vi "OP_Print_TPS_cluster20171206.vi"() -> ()   [LabVIEW 2013]
uses:
  <vilib>/addons/database/Connection.llb/DB Tools Open Connec (Path).vi
  <vilib>/addons/database/Connection.llb/Conn Execute.vi
  <vilib>/addons/database/Recordset.llb/Rec Fetch Recordset Data (R).vi
  <vilib>/addons/database/Recordset.llb/Rec Destroy - Connection.vi
  <userlib>/caLab/Private/Get_PV-1D.vi
  <vilib>/Utility/file.llb/Write To Spreadsheet File (string).vi
  <userlib>/caLab/Private/Get_PV.vi
  <vilib>/addons/database/NI_Database_API.lvlib
panel:
  in  "WindowsMediaPlayer":refnum<k7>(container)
  in  "Vol.":i32(slide)=12 min=0 max=100 step=1 scale=0.0..100.0
  out "index":i32
  in  "Play Button":bool
  in  "Skip Forward Button":bool
  in  "Skip Back Button":bool
  in  "Pause Button":bool
  out "appended path":path=path "C:/Users/TPSOP/Desktop/新增資料夾 (2)/musics/1.mp3"
  out "status":string="就緒"
  out "error out":errorcluster
  out "new picture":picture
  in  "T:Slow\nF:Fast":bool
  in  "Switch Tab":bool=TRUE
  out "Tab Control":enum32{"_____", "           "}(tab)
  out "Cluster":T1={"SR Fill Pattern"=[], "Beam Current(mA"=320.769453, "Beam Lifetime(min)"=354.3939151043138, "Beamsize X(um)"=63.15189373514937, "Beamsize Y(um)"=38.03691397287648, "Tune X(from BPM)"=0.1487279843444227, "Tune Y(from BPM)"=0.2309197651663405, "Mode"="Top-Up", "NuX(from BBF) "=0.15142063757609414, "NuY(from BBF)"=0.22496346361412184, "IU22-23gap(R)"=7.0, "IU22-05gap(R)"=7.372, "IU22-05M"=TRUE, "IU22A-09gap(R)"=8.05, "IU22A-09M"=TRUE, "IU22B-09gap(R)"=40.001, "IU22B-09M"=FALSE, "IUT22-21gap(R)"=7.0, "IUT22-21M"=TRUE, "IU22-23M"=TRUE, "IU22A-25gap(R)"=7.0, "IU22A-25M"=TRUE, "IU22B-25gap(R)"=40.0, "IU22B-25M"=FALSE, "EPU48A-41gap(R)"=65.00055, "EPU48A-41gM"=FALSE, "EPU48B-41gap(R)"=27.450000000000003, "EPU48B-41gM"=TRUE, "EPU46-45gap(R)"=44.99850000000001, "EPU46-45gM"=FALSE, "EPU48A-41phase(R)"=0.00055, "EPU48B-41phase(R)"=0.0, "EPU46-45phase(R)"=5e-05, "Grid volt.(V)[S]"=33.0, "Gun mode"="MBM", "Mod.3 HV(kV)[S]"=35.37999999999996, "SR"="SR_DMB_2017_1024_0300LOCO.data", "BR"="Booster_2017_1023_0900.data", "LI"="Linac_2017_0413_1015.data", "LTB"="LTB_JT_2017_0828_1050.data", "BTS"="BTS_2017_1023_0900.data", "RF2 remote"=TRUE, "RF2 OP mode"=TRUE, "RF2 phase.[S]"=-42.0, "RF Freq.(s)"=499655365.67399085, "RF2 gap volt[S]"=1600.0, "RF3 remote"=TRUE, "RF3 OP mode"=TRUE, "RF3 phase.[S]"=1.1999999999999995, "RF3 gap volt.[S]"=1600.0, "BBF V"=TRUE, "BBF H"=TRUE, "BR ext. kicker1(kV)"=17.666, "BR ext. kicker2(kV)"=17.666, "BR ext. sep.1(V)"=322.14, "BR ext. sep.2(V)"=441.1, "BR inj. sep.(V)"=104.95, "BR inj. kicker(kV)"=13.449999999999969, "SR kicker4(kV)"=7.945, "SR kicker3(kV)"=8.02, "SR kicker2(kV)"=8.142, "SR kicker1(kV)"=8.1, "SR inj. sep.2(V)"=397.2, "SR inj. sep.1(V)"=398.04, "Bucket Start"=100.0, "Bucket Last"=450.0, "Bucket Step"=10.0, "Orbit ILK(P)"=TRUE, "IU22-05 Hutch Enable"=TRUE, "IU22A-09M Hutch Enable"=TRUE, "IUT22-21M Hutch Enable"=TRUE, "IU22-23M Hutch Enable"=TRUE, "IU22A-25M Hutch Enable"=TRUE, "EPU48A-41M Hutch Enable"=TRUE, "EPU46-45M Hutch Enable"=FALSE, "EPU46-45 FE Enable"=TRUE, "EPU48A-41 FE Enable"=TRUE, "IU22A-25 FE Enable"=TRUE, "IU22-23 FE Enable"=TRUE, "IUT22-21 FE Enable"=TRUE, "IU22A-09 FE Enable"=TRUE, "IU22-05 FE Enable"=TRUE, "EPU48A-41pM"=FALSE, "EPU48B-41pM"=TRUE, "EPU46-45pM"=FALSE, "Gun volt.(V)[S]"=23.5, "Width count"=75.0, "2ns step"=2.0, "10ps delay"=150.0, "phase shifter"=130.0015, "Taper"=1.0899999999999999, "05XBPMX 1"=14.279, "09XBPMX 1"=-34.837, "21XBPMX 1"=-36.466, "23XBPMX 1"=-38.547000000000004, "25XBPMX 1"=-40.08, "41XBPMX 1"=-513.551, "45XBPMX 1"=-12.86, "05XBPMY 1"=51.999, "09XBPMY 1"=30.004, "21XBPMY 1"=-4.771, "23XBPMY 1"=19.080000000000002, "25XBPMY 1"=-4.366, "41XBPMY 1"=309.241, "45XBPMY 1"=1.842, "FOFB H"="On", "FOFB V"="On", "time string"="15:45:09", "date"="2017/10/28", "date (last kicker ON)"="", "time string (last kicker ON)"="", "Radio Buttons 2"=enum."absolute", "09XBPMX 2"="23.77", "09XBPMY 2"="-18.01", "05XBPMY 2"="-459.85", "05XBPMX 2"="-403.56", "21XBPMY 2"="-134.87", "21XBPMX 2"="-31.92", "23XBPMY 2"="233.82", "23XBPMX 2"="11.09", "25XBPMY 2"="5171.53", "25XBPMX 2"="2152.43", "41XBPMY 2"=" closed", "41XBPMX 2"=" PAB ", "45XBPMX 2"=" Hutch ", "45XBPMY 2"=" closed", "05 mode"="Follow", "09A mode"="Follow", "09B mode"="Follow", "21 mode"="Follow", "23 mode"="Follow", "25A mode"="Follow", "25B mode"="Follow", "41A mode"="Follow", "41B mode"="Follow", "46 mode"="Follow", "BeamCurrent History"={"BPM NO.  1_172"=array[4319 elements], array[4319 elements]}, "SR Beam Current in            hours"=12.0, "RF FB"="On", "gap value："=0, "BR Fill Pattern"=[], "time string (last INJ) "="", "BPMX Graph 2"={"Array of X axis  平均分配至各段"=[1.0, 1.1666666666666667, 1.3333333333333333, 1.5, 1.6666666666666665, 1.8333333333333333, 2.0, 2.142857142857143, 2.2857142857142856, 2.4285714285714284, 2.571428571428571, 2.7142857142857144, 2.857142857142857, 3.0, 3.142857142857143, 3.2857142857142856, 3.4285714285714284, 3.571428571428571, 3.7142857142857144, 3.857142857142857, 4.0, 4.125, 4.25, 4.375, 4.5, 4.625, 4.75, 4.875, 5.0, 5.125, 5.25, 5.375, 5.5, 5.625, 5.75, 5.875, 6.0, 6.142857142857143, 6.285714285714286, 6.428571428571429, 6.571428571428571, 6.714285714285714, 6.857142857142857, 7.0, 7.142857142857143, 7.285714285714286, 7.428571428571429, 7.571428571428571, 7.714285714285714, 7.857142857142857, 8.0, 8.142857142857142, 8.285714285714286, 8.428571428571429, 8.571428571428571, 8.714285714285714, 8.857142857142858, 9.0, 9.142857142857142, 9.285714285714286, 9.428571428571429, 9.571428571428571, 9.714285714285714, 9.857142857142858, 10.0, 10.142857142857142, 10.285714285714286, 10.428571428571429, 10.571428571428571, 10.714285714285714, 10.857142857142858, 11.0, 11.142857142857142, 11.285714285714286, 11.428571428571429, 11.571428571428571, 11.714285714285714, 11.857142857142858, 12.0, 12.125, 12.25, 12.375, 12.5, 12.625, 12.75, 12.875, 13.0, 13.125, 13.25, 13.375, 13.5, 13.625, 13.75, 13.875, 14.0, 14.142857142857142, 14.285714285714286, 14.428571428571429, 14.571428571428571, 14.714285714285714, 14.857142857142858, 15.0, 15.142857142857142, 15.285714285714286, 15.428571428571429, 15.571428571428571, 15.714285714285714, 15.857142857142858, 16.0, 16.142857142857142, 16.285714285714285, 16.428571428571427, 16.571428571428573, 16.714285714285715, 16.857142857142858, 17.0, 17.142857142857142, 17.285714285714285, 17.428571428571427, 17.571428571428573, 17.714285714285715, 17.857142857142858, 18.0, 18.142857142857142, 18.285714285714285, 18.428571428571427, 18.571428571428573, 18.714285714285715, 18.857142857142858, 19.0, 19.142857142857142, 19.285714285714285, 19.428571428571427, 19.571428571428573, 19.714285714285715, 19.857142857142858, 20.0, 20.125, 20.25, 20.375, 20.5, 20.625, 20.75, 20.875, 21.0, 21.125, 21.25, 21.375, 21.5, 21.625, 21.75, 21.875, 22.0, 22.142857142857142, 22.285714285714285, 22.428571428571427, 22.571428571428573, 22.714285714285715, 22.857142857142858, 23.0, 23.142857142857142, 23.285714285714285, 23.428571428571427, 23.571428571428573, 23.714285714285715, 23.857142857142858, 24.0, 24.166666666666668, 24.333333333333332, 24.5, 24.666666666666668, 24.833333333333332], [-104.35000000000001, -27.61, -81.269, 31.074, 6.062, -136.0, 99.494, -88.141, -46.889, -165.06900000000002, 6.021, -84.98, 1.75, -8.811, 8.532, -133.949, -96.848, 24.799, 5.059, -100.301, 144.643, -9.353, 21.271, -55.053000000000004, 53.308, 191.175, 158.868, 222.566, -123.501, -26.869, 534.8770000000001, 573.141, -225.076, -6.779, 120.711, -75.419, 85.256, 50.948, -59.4, -203.09900000000002, -20.847, 130.465, -112.508, 76.115, 15.039, -35.207, -105.659, -16.897000000000002, 68.91, -141.159, 107.378, 144.351, -55.053000000000004, -193.076, 129.21, 58.157000000000004, -162.566, 153.643, 28.149, 9.358, -84.211, 85.112, 22.422, -31.252, 89.379, -47.49, 54.793, -68.275, 110.611, -118.584, -371.90500000000003, -20.115000000000002, -329.103, -249.097, -146.817, 118.556, -25.749, -98.32600000000001, 55.269, -122.093, 50.967, -55.89, 88.019, -0.462, -608.1560000000001, -139.752, -304.999, -215.022, 93.23400000000001, 44.699, -65.235, 37.049, -3.491, -169.852, 216.458, 50.398, -92.285, -132.13400000000001, -12.869, 66.74, -188.53300000000002, 148.653, -5.112, -71.334, -177.681, 41.168, -12.532, -184.913, 194.919, 52.414, -75.628, -80.415, -36.814, 105.73100000000001, -104.36800000000001, 110.101, 49.669000000000004, -67.327, -157.372, 29.624000000000002, 22.156, -105.663, 47.799, 11.591000000000001, -75.285, -79.821, 34.331, -24.937, -158.703, 177.15, 200.872, -165.849, -60.67, 20.183, -15.311, -111.206, 107.58800000000001, 26.489, 69.547, -41.230000000000004, 81.986, 54.43, 253.076, 378.43600000000004, -117.003, -304.999, 131.013, 2.21, -158.435, 94.489, 63.017, -82.94500000000001, 99.147, 65.752, -37.261, -102.577, 41.791000000000004, 66.599, -163.73, 160.137, -7.15, -51.275, -140.353, 33.772, 54.203, -147.597, 128.696, 58.22, -47.144, -184.493, 56.980000000000004, 67.437, -54.227000000000004, -0.031]}, "BPMY Graph 2"={"Array of X axis  平均分配至各段"=[1.0, 1.1666666666666667, 1.3333333333333333, 1.5, 1.6666666666666665, 1.8333333333333333, 2.0, 2.142857142857143, 2.2857142857142856, 2.4285714285714284, 2.571428571428571, 2.7142857142857144, 2.857142857142857, 3.0, 3.142857142857143, 3.2857142857142856, 3.4285714285714284, 3.571428571428571, 3.7142857142857144, 3.857142857142857, 4.0, 4.125, 4.25, 4.375, 4.5, 4.625, 4.75, 4.875, 5.0, 5.125, 5.25, 5.375, 5.5, 5.625, 5.75, 5.875, 6.0, 6.142857142857143, 6.285714285714286, 6.428571428571429, 6.571428571428571, 6.714285714285714, 6.857142857142857, 7.0, 7.142857142857143, 7.285714285714286, 7.428571428571429, 7.571428571428571, 7.714285714285714, 7.857142857142857, 8.0, 8.142857142857142, 8.285714285714286, 8.428571428571429, 8.571428571428571, 8.714285714285714, 8.857142857142858, 9.0, 9.142857142857142, 9.285714285714286, 9.428571428571429, 9.571428571428571, 9.714285714285714, 9.857142857142858, 10.0, 10.142857142857142, 10.285714285714286, 10.428571428571429, 10.571428571428571, 10.714285714285714, 10.857142857142858, 11.0, 11.142857142857142, 11.285714285714286, 11.428571428571429, 11.571428571428571, 11.714285714285714, 11.857142857142858, 12.0, 12.125, 12.25, 12.375, 12.5, 12.625, 12.75, 12.875, 13.0, 13.125, 13.25, 13.375, 13.5, 13.625, 13.75, 13.875, 14.0, 14.142857142857142, 14.285714285714286, 14.428571428571429, 14.571428571428571, 14.714285714285714, 14.857142857142858, 15.0, 15.142857142857142, 15.285714285714286, 15.428571428571429, 15.571428571428571, 15.714285714285714, 15.857142857142858, 16.0, 16.142857142857142, 16.285714285714285, 16.428571428571427, 16.571428571428573, 16.714285714285715, 16.857142857142858, 17.0, 17.142857142857142, 17.285714285714285, 17.428571428571427, 17.571428571428573, 17.714285714285715, 17.857142857142858, 18.0, 18.142857142857142, 18.285714285714285, 18.428571428571427, 18.571428571428573, 18.714285714285715, 18.857142857142858, 19.0, 19.142857142857142, 19.285714285714285, 19.428571428571427, 19.571428571428573, 19.714285714285715, 19.857142857142858, 20.0, 20.125, 20.25, 20.375, 20.5, 20.625, 20.75, 20.875, 21.0, 21.125, 21.25, 21.375, 21.5, 21.625, 21.75, 21.875, 22.0, 22.142857142857142, 22.285714285714285, 22.428571428571427, 22.571428571428573, 22.714285714285715, 22.857142857142858, 23.0, 23.142857142857142, 23.285714285714285, 23.428571428571427, 23.571428571428573, 23.714285714285715, 23.857142857142858, 24.0, 24.166666666666668, 24.333333333333332, 24.5, 24.666666666666668, 24.833333333333332], [-143.858, -13.775, -13.785, 122.665, -66.475, 31.541, 2.118, -24.67, 28.275000000000002, 0.139, -36.578, -28.396, 48.925000000000004, 9.287, -3.412, 70.053, -21.479, 14.89, -7.234, 5.521, -3.164, 19.558, -37.538000000000004, 37.11, -77.159, -13.755, 77.63, 28.249000000000002, -209.114, -44.569, 92.851, 173.641, -70.156, -22.722, 17.795, -6.59, 25.654, -41.882, 53.713, 9.237, -26.164, 18.357, 63.695, -8.542, 5.183, -5.99, 9.508000000000001, -5.462, -29.446, 36.574, -52.552, 51.439, -48.502, 0.73, -23.836000000000002, -3.648, -9.628, -5.485, -68.679, 95.486, -62.041000000000004, 54.633, -58.791000000000004, 68.305, -49.682, 29.838, -8.459, 3.213, -5.561, -80.617, 58.144, 15.346, -158.743, -40.726, 5.259, 3.258, 41.128, -54.377, 5.01, 18.84, 11.403, -20.73, 21.792, -17.296, 27.29, 0.783, -6.804, -137.476, 116.70700000000001, -6.929, 17.846, -3.586, 11.754, 6.341, 0.292, -0.911, -8.236, -5.312, 14.939, -29.945, 30.573, -9.991, -49.344, 82.117, -27.45, 22.291, -6.636, -9.389, 10.034, -14.218, 14.215, -7.3, 12.409, -44.302, 50.197, -36.089, -9.120000000000001, 45.881, 14.836, -27.324, 10.765, -10.139, -33.252, 2.737, -9.99, -6.019, -53.329, -28.159, 2.676, -36.9, -2.372, 8.92, 13.599, -25.723, -16.436, 7.722, -0.088, -29.122, 32.814, -20.521, 30.155, -45.734, 36.611000000000004, 74.528, 68.482, -22.548000000000002, -31.398, 134.603, -45.587, -0.981, -40.156, 24.441, 20.477, -31.424, 19.5, -11.789, 16.394000000000002, -38.567, 9.523, 0.09, -0.058, -4.8500000000000005, 11.71, 25.637, -10.51, -18.101, -12.389000000000001, 95.417, -138.726, 30.355, 96.245, -48.666000000000004, 40.851, -0.71]}} {"SR Beam Current in            hours" min=1.0 max=24.0 step=1.0 format="%#_2f"; "45XBPMY 1" format="%#.2f"; "41XBPMY 1" format="%#.2f"; "25XBPMY 1" format="%#.2f"; "23XBPMY 1" format="%#.2f"; "21XBPMY 1" format="%#.2f"; "09XBPMY 1" format="%#.2f"; "05XBPMY 1" format="%#.2f"; "45XBPMX 1" format="%#.2f"; "41XBPMX 1" format="%#.2f"; "25XBPMX 1" format="%#.2f"; "23XBPMX 1" format="%#.2f"; "21XBPMX 1" format="%#.2f"; "09XBPMX 1" format="%#.2f"; "05XBPMX 1" format="%#.2f"; "Taper" format="%#.4f"; "phase shifter" format="%#.3f"; "10ps delay" format="%#.1f"; "2ns step" format="%#.1f"; "Width count" format="%#.1f"; "Gun volt.(V)[S]" format="%#.1f"; "Bucket Step" format="%#.2f"; "Bucket Last" format="%#.2f"; "Bucket Start" format="%#.2f"; "BR ext. kicker1(kV)" format="%#.2f"; "BR ext. kicker2(kV)" format="%#.2f"; "BR ext. sep.1(V)" format="%#.2f"; "BR ext. sep.2(V)" format="%#.2f"; "BR inj. sep.(V)" format="%#.3f"; "BR inj. kicker(kV)" format="%#.3f"; "SR kicker4(kV)" format="%#.2f"; "SR kicker3(kV)" format="%#.2f"; "SR kicker2(kV)" format="%#.2f"; "SR kicker1(kV)" format="%#.2f"; "SR inj. sep.2(V)" format="%#.2f"; "SR inj. sep.1(V)" format="%#.2f"; "RF3 gap volt.[S]" format="%#.0f"; "RF3 phase.[S]" format="%#.1f"; "RF2 gap volt[S]" format="%#.0f"; "RF Freq.(s)" format="%#.1f"; "RF2 phase.[S]" format="%#.1f"; "Mod.3 HV(kV)[S]" format="%#.3f"; "Grid volt.(V)[S]" format="%#.1f"; "EPU46-45phase(R)" format="%#.4f"; "EPU48B-41phase(R)" format="%#.4f"; "EPU48A-41phase(R)" format="%#.4f"; "EPU46-45gap(R)" format="%#.4f"; "EPU48B-41gap(R)" format="%#.4f"; "EPU48A-41gap(R)" format="%#.4f"; "IU22B-25gap(R)" format="%#.4f"; "IU22A-25gap(R)" format="%#.4f"; "IUT22-21gap(R)" format="%#.4f"; "IU22B-09gap(R)" format="%#.4f"; "IU22A-09gap(R)" format="%#.4f"; "IU22-05gap(R)" format="%#.4f"; "IU22-23gap(R)" format="%#.4f"; "NuY(from BBF)" format="%#.4f"; "NuX(from BBF)" format="%#.4f"; "Tune Y(from BPM)" format="%#.4f"; "Tune X(from BPM)" format="%#.4f"; "Beamsize Y(um)" format="%#.2f"; "Beamsize X(um)" format="%#.2f"; "Beam Lifetime(min)" format="%#.3f"; "Beam Current(mA" format="%#.3f"}
  out "Diff list":string[][](array[string])
  out "EVENTs":i32
  out "check loop":i32
  in  "Check period":i32=10 min=0 max=10
  out "Program Start Time":dbl=3592021508.642459
  out "dT":u32=325
  out "PV list":string[](array[string])=["LI-ES-CPS-01:SETMODE", "LI-ES-CPS-01:PULSEMODE", "LI-ES-BPS-01:SETU:GRID", "LI-ES-BPS-01:SETU:SBM", "LI-ES-BPS-01:SETU:MBM", "LI-RF-CAB-07:SET:MODE", "LI-RF-HVP-11:SET:U", "LI-RF-CAB-09:SET:MODE", "LI-RF-HVP-21:SET:U", "LI-RF-CAB-11:SET:MODE", "LI-RF-HVP-31:SET:U", "LI-RF-WGA-01:SET:POS", "LI-RF-WGA-02:SET:POS", "LI-RF-WGA-03:SET:POS", "LI-RF-SFT-01:SET:POS", "LI-RF-SFT-02:SET:POS", "LI-RF-SFT-03:SET:POS", "LI-RF-CTR-01:ES:SET:DEG", "LI-RF-CTR-01:SP:SET:DEG", "LI-RF-CTR-01:K123:SET:DEG", "LI-RF-CTR-01:K1:SET:DEG", "LI-RF-CTR-01:K3:SET:DEG", "LI-RF-AMP-01:SET:PWR", "LI-RF-AMP-02:SET:PWR", "LI-MA-SPS-01:SET:I", "LI-MA-SPS-02:SET:I", "LI-MA-SPS-03:SET:I", "LI-MA-SPS-04:SET:I", "LI-MA-SPS-05:SET:I", "LI-MA-SPS-06:SET:I", "LI-MA-SPS-07:SET:I", "LI-MA-SPS-08:SET:I", "LI-MA-SPS-09:SET:I", "LI-MA-SPS-10:SET:I", "LI-MA-SPS-11:SET:I", "LI-MA-SPS-12:SET:I", "LI-MA-SPS-13:SET:I", "LI-MA-SPS-14:SET:I", "LI-MA-SPS-15:SET:I", "LI-MA-SPS-16:SET:I", "LI-MA-STP-01:SET:I", "LI-MA-STP-02:SET:I", "LI-MA-STP-03:SET:I", "LI-MA-STP-04:SET:I", "LI-MA-STP-05:SET:I", "LI-MA-STP-06:SET:I", "LI-MA-STP-07:SET:I", "LI-MA-STP-08:SET:I", "LI-MA-STP-09:SET:I", "LI-MA-STP-10:SET:I", "LI-MA-STP-11:SET:I", "LI-MA-STP-12:SET:I", "LI-MA-STP-13:SET:I", "LI-MA-STP-14:SET:I", "LI-MA-STP-15:SET:I", "LI-MA-STP-16:SET:I", "LI-MA-QPS-01:SET:I", "LI-MA-QPS-02:SET:I", "LI-MA-QPS-03:SET:I", "LI-MA-QPS-04:SET:I", "LI-MA-QPS-05:SET:I", "LI-MA-QPS-06:SET:I", "CPCITM-TI-EVRTG:Pulse7DelaySet", "CPCITM-TI-EVRTG:Pulse7WidthSet", "CPCITM-TI-EVRTG:GTX7CtrlGTXPHSet", "CPCITM-TI-EVRTG:GTX7DlySet", "CPCITM-TI-EVRTG:Pulse6DelaySet", "CPCITM-TI-EVRTG:Pulse6WidthSet", "CPCITM-TI-EVRTG:GTX6CtrlGTXPHSet", "CPCITM-TI-EVRTG:GTX6DlySet", "CPCILI-TI-EVR:Pulse2DelaySet", "CPCILI-TI-EVR:Pulse2WidthSet", "CPCILI-TI-EVR:Pulse3DelaySet", "CPCILI-TI-EVR:Pulse3WidthSet", "CPCILI-TI-EVR:Pulse4DelaySet", "CPCILI-TI-EVR:Pulse4WidthSet", "CPCILI-TI-EVR:Pulse5DelaySet", "CPCILI-TI-EVR:Pulse5WidthSet", "CPCILI-TI-EVR:Pulse6DelaySet", "CPCILI-TI-EVR:Pulse6WidthSet", "CPCILI-TI-EVR:Pulse7DelaySet", "CPCILI-TI-EVR:Pulse7WidthSet", "CPCILI-TI-EVR:Pulse8DelaySet", "CPCILI-TI-EVR:Pulse8WidthSet", "CPCILI-TI-EVR:Pulse9DelaySet", "CPCILI-TI-EVR:Pulse9WidthSet", "CPCITM-TI-EVRTG:GTX6DlySet", "CPCITM-TI-EVRTG:GTX7DlySet", "LTB-PS-HC-1:setI", "LTB-PS-HC-2:setI", "LTB-PS-HC-3:setI", "LTB-PS-HC-4:setI", "LTB-PS-HC-5:setI", "LTB-PS-VC-1:setI", "LTB-PS-VC-2:setI", "LTB-PS-VC-3:setI", "LTB-PS-VC-4:setI", "LTB-PS-VC-5:setI", "LTB-PS-VC-6:setI", "LTB-PS-VC-7:setI", "LTB-PS-Q1A:setI", "LTB-PS-Q1B:setI", "LTB-PS-Q1C:setI", "LTB-PS-Q2A:setI", "LTB-PS-Q2B:setI", "LTB-PS-Q2C:setI", "LTB-PS-Q3A:setI", "LTB-PS-Q3B:setI", "LTB-PS-Q4A:setI", "LTB-PS-Q4B:setI", "LTB-PS-QQ:setI", "LTB-PS-BEND-1:setI", "LTB-PS-VC-2a:setI", "LTB-PS-HC-3a:setI", "LTB-PS-HC-3b:setI", "LTB-PS-HC-4a:setI", "LTB-PS-HC-5a:setI", "LI-DI-SLIT-motor:axis2Position1", "LI-DI-SLIT-motor:axis1Position1", "BR-PS-HC-101:setI", "BR-PS-HC-102:setI", "BR-PS-HC-103:setI", "BR-PS-HC-104:setI", "BR-PS-HC-105:setI", "BR-PS-HC-106:setI", "BR-PS-HC-107:setI", "BR-PS-HC-108:setI", "BR-PS-HC-109:setI", "BR-PS-HC-110:setI", "BR-PS-HC-201:setI", "BR-PS-HC-202:setI", "BR-PS-HC-203:setI", "BR-PS-HC-204:setI", "BR-PS-HC-205:setI", "BR-PS-HC-206:setI", "BR-PS-HC-207:setI", "BR-PS-HC-208:setI", "BR-PS-HC-209:setI", "BR-PS-HC-210:setI", "BR-PS-HC-301:setI", "BR-PS-HC-302:setI", "BR-PS-HC-303:setI", "BR-PS-HC-304:setI", "BR-PS-HC-305:setI", "BR-PS-HC-306:setI", "BR-PS-HC-307:setI", "BR-PS-HC-308:setI", "BR-PS-HC-309:setI", "BR-PS-HC-310:setI", "BR-PS-HC-401:setI", "BR-PS-HC-402:setI", "BR-PS-HC-403:setI", "BR-PS-HC-404:setI", "BR-PS-HC-405:setI", "BR-PS-HC-406:setI", "BR-PS-HC-407:setI", "BR-PS-HC-408:setI", "BR-PS-HC-409:setI", "BR-PS-HC-410:setI", "BR-PS-HC-501:setI", "BR-PS-HC-502:setI", "BR-PS-HC-503:setI", "BR-PS-HC-504:setI", "BR-PS-HC-505:setI", "BR-PS-HC-506:setI", "BR-PS-HC-507:setI", "BR-PS-HC-508:setI", "BR-PS-HC-509:setI", "BR-PS-HC-510:setI", "BR-PS-HC-601:setI", "BR-PS-HC-602:setI", "BR-PS-HC-603:setI", "BR-PS-HC-603a:setI", "BR-PS-HC-604:setI", "BR-PS-HC-605:setI", "BR-PS-HC-606:setI", "BR-PS-HC-606a:setI", "BR-PS-HC-607:setI", "BR-PS-HC-608:setI", "BR-PS-HC-609:setI", "BR-PS-HC-610:setI", "BR-PS-VC-101:setI", "BR-PS-VC-102:setI", "BR-PS-VC-103:setI", "BR-PS-VC-104:setI", "BR-PS-VC-105:setI", "BR-PS-VC-106:setI", "BR-PS-VC-201:setI", "BR-PS-VC-202:setI", "BR-PS-VC-203:setI", "BR-PS-VC-204:setI", "BR-PS-VC-205:setI", "BR-PS-VC-206:setI", "BR-PS-VC-301:setI", "BR-PS-VC-302:setI", "BR-PS-VC-303:setI", "BR-PS-VC-304:setI", "BR-PS-VC-305:setI", "BR-PS-VC-306:setI", "BR-PS-VC-401:setI", "BR-PS-VC-402:setI", "BR-PS-VC-403:setI", "BR-PS-VC-404:setI", "BR-PS-VC-405:setI", "BR-PS-VC-406:setI", "BR-PS-VC-501:setI", "BR-PS-VC-502:setI", "BR-PS-VC-503:setI", "BR-PS-VC-504:setI", "BR-PS-VC-505:setI", "BR-PS-VC-506:setI", "BR-PS-VC-601:setI", "BR-PS-VC-602:setI", "BR-PS-VC-602a:setI", "BR-PS-VC-603:setI", "BR-PS-VC-604:setI", "BR-PS-VC-604a:setI", "BR-PS-VC-605:setI", "BR-PS-VC-606:setI", "BR-PS-VC-100a:setI", "BR-PS-SD:setI", "BR-PS-SF:setI", "cpsc_027:AO:SLOW_SET:CH:1", "cpsc_037:AO:SLOW_SET:CH:3", "BR-RF-LLRF:setStationPhase", "TI-INJ-PROC:setTinj", "BR-PS-INJ-SE:setHV", "CPCIPM-TI-EVR:Pulse1DelaySet", "BR-PS-INJ-KI:setHV", "CPCIPM-TI-EVR:Pulse2DelaySet", "BR-PS-QF:setWfDC", "BR-PS-QM:setWfDC", "BR-PS-Q1:setWfDC", "BR-PS-Q2:setWfDC", "BR-PS-BEND:setWfDC", "BTS-PS-HC-1:setI", "BTS-PS-HC-2:setI", "BTS-PS-HC-3:setI", "BTS-PS-HC-4:setI", "BTS-PS-HC-5:setI", "BTS-PS-VC-2:setI", "BTS-PS-VC-3:setI", "BTS-PS-VC-4:setI", "BTS-PS-VC-5:setI", "BTS-PS-VC-6:setI", "BTS-PS-Q1A:setI", "BTS-PS-Q1B:setI", "BTS-PS-Q1C:setI", "BTS-PS-Q2A:setI", "BTS-PS-Q2B:setI", "BTS-PS-Q2C:setI", "BTS-PS-Q3A:setI", "BTS-PS-BEND-1:setI", "BTS-PS-BEND-2:setI", "BR-PS-EXT-K1:setHV", "BR-PS-EXT-K2:setHV", "SR-PS-INJ-SE1:setHV", "SR-PS-INJ-SE2:setHV", "SR-PS-INJ-K1:setHV", "SR-PS-INJ-K2:setHV", "SR-PS-INJ-K3:setHV", "SR-PS-INJ-K4:setHV", "CPCIPM-TI-EVR:Pulse4DelaySet", "CPCIPM-TI-EVR:Pulse5DelaySet", "CPCIPM-TI-EVR:Pulse3DelaySet", "CPCIPM-TI-EVR:Pulse6DelaySet", "CPCIPM-TI-EVR:Pulse7DelaySet", "T560:setADelay", "T560:setBDelay", "T560:setCDelay", "T560:setDDelay", "CPCIPM-TI-EVR:Pulse4DelaySet", "CPCIPM-TI-EVR:Pulse5DelaySet", "BR-PS-EXT-SE1:setHV", "BR-PS-EXT-SE2:setHV", "CPCIPM-TI-EVR:Pulse3DelaySet", "CPCIPM-TI-EVR:Pulse11DelaySet", "SR-PS-BEND:setI", "SR-PS-HC-011:setI", "SR-PS-HC-012:setI", "SR-PS-HC-013:setI", "SR-PS-HC-014:setI", "SR-PS-HC-015:setI", "SR-PS-HC-016:setI", "SR-PS-HC-017:setI", "SR-PS-HC-021:setI", "SR-PS-HC-022:setI", "SR-PS-HC-023:setI", "SR-PS-HC-024:setI", "SR-PS-HC-025:setI", "SR-PS-HC-026:setI", "SR-PS-HC-027:setI", "SR-PS-HC-031:setI", "SR-PS-HC-032:setI", "SR-PS-HC-033:setI", "SR-PS-HC-034:setI", "SR-PS-HC-035:setI", "SR-PS-HC-036:setI", "SR-PS-HC-037:setI", "SR-PS-HC-041:setI", "SR-PS-HC-042:setI", "SR-PS-HC-043:setI", "SR-PS-HC-044:setI", "SR-PS-HC-045:setI", "SR-PS-HC-046:setI", "SR-PS-HC-047:setI", "SR-PS-HC-051:setI", "SR-PS-HC-052:setI", "SR-PS-HC-053:setI", "SR-PS-HC-054:setI", "SR-PS-HC-055:setI", "SR-PS-HC-056:setI", "SR-PS-HC-057:setI", "SR-PS-HC-061:setI", "SR-PS-HC-062:setI", "SR-PS-HC-063:setI", "SR-PS-HC-064:setI", "SR-PS-HC-065:setI", "SR-PS-HC-066:setI", "SR-PS-HC-067:setI", "SR-PS-HC-071:setI", "SR-PS-HC-072:setI", "SR-PS-HC-073:setI", "SR-PS-HC-074:setI", "SR-PS-HC-075:setI", "SR-PS-HC-076:setI", "SR-PS-HC-077:setI", "SR-PS-HC-081:setI", "SR-PS-HC-082:setI", "SR-PS-HC-083:setI", "SR-PS-HC-084:setI", "SR-PS-HC-085:setI", "SR-PS-HC-086:setI", "SR-PS-HC-087:setI", "SR-PS-HC-091:setI", "SR-PS-HC-092:setI", "SR-PS-HC-093:setI", "SR-PS-HC-094:setI", "SR-PS-HC-095:setI", "SR-PS-HC-096:setI", "SR-PS-HC-097:setI", "SR-PS-HC-101:setI", "SR-PS-HC-102:setI", "SR-PS-HC-103:setI", "SR-PS-HC-104:setI", "SR-PS-HC-105:setI", "SR-PS-HC-106:setI", "SR-PS-HC-107:setI", "SR-PS-HC-111:setI", "SR-PS-HC-112:setI", "SR-PS-HC-113:setI", "SR-PS-HC-114:setI", "SR-PS-HC-115:setI", "SR-PS-HC-116:setI", "SR-PS-HC-117:setI", "SR-PS-HC-121:setI", "SR-PS-HC-122:setI", "SR-PS-HC-123:setI", "SR-PS-HC-124:setI", "SR-PS-HC-125:setI", "SR-PS-HC-126:setI", "SR-PS-HC-127:setI", "SR-PS-HC-131:setI", "SR-PS-HC-132:setI", "SR-PS-HC-133:setI", "SR-PS-HC-134:setI", "SR-PS-HC-135:setI", "SR-PS-HC-136:setI", "SR-PS-HC-137:setI", "SR-PS-HC-141:setI", "SR-PS-HC-142:setI", "SR-PS-HC-143:setI", "SR-PS-HC-144:setI", "SR-PS-HC-145:setI", "SR-PS-HC-146:setI", "SR-PS-HC-147:setI", "SR-PS-HC-151:setI", "SR-PS-HC-152:setI", "SR-PS-HC-153:setI", "SR-PS-HC-154:setI", "SR-PS-HC-155:setI", "SR-PS-HC-156:setI", "SR-PS-HC-157:setI", "SR-PS-HC-161:setI", "SR-PS-HC-162:setI", "SR-PS-HC-163:setI", "SR-PS-HC-164:setI", "SR-PS-HC-165:setI", "SR-PS-HC-166:setI", "SR-PS-HC-167:setI", "SR-PS-HC-171:setI", "SR-PS-HC-172:setI", "SR-PS-HC-173:setI", "SR-PS-HC-174:setI", "SR-PS-HC-175:setI", "SR-PS-HC-176:setI", "SR-PS-HC-177:setI", "SR-PS-HC-181:setI", "SR-PS-HC-182:setI", "SR-PS-HC-183:setI", "SR-PS-HC-184:setI", "SR-PS-HC-185:setI", "SR-PS-HC-186:setI", "SR-PS-HC-187:setI", "SR-PS-HC-191:setI", "SR-PS-HC-192:setI", "SR-PS-HC-193:setI", "SR-PS-HC-194:setI", "SR-PS-HC-195:setI", "SR-PS-HC-196:setI", "SR-PS-HC-197:setI", "SR-PS-HC-201:setI", "SR-PS-HC-202:setI", "SR-PS-HC-203:setI", "SR-PS-HC-204:setI", "SR-PS-HC-205:setI", "SR-PS-HC-206:setI", "SR-PS-HC-207:setI", "SR-PS-HC-211:setI", "SR-PS-HC-212:setI", "SR-PS-HC-213:setI", "SR-PS-HC-214:setI", "SR-PS-HC-215:setI", "SR-PS-HC-216:setI", "SR-PS-HC-217:setI", "SR-PS-HC-221:setI", "SR-PS-HC-222:setI", "SR-PS-HC-223:setI", "SR-PS-HC-224:setI", "SR-PS-HC-225:setI", "SR-PS-HC-226:setI", "SR-PS-HC-227:setI", "SR-PS-HC-231:setI", "SR-PS-HC-232:setI", "SR-PS-HC-233:setI", "SR-PS-HC-234:setI", "SR-PS-HC-235:setI", "SR-PS-HC-236:setI", "SR-PS-HC-237:setI", "SR-PS-HC-241:setI", "SR-PS-HC-242:setI", "SR-PS-HC-243:setI", "SR-PS-HC-244:setI", "SR-PS-HC-245:setI", "SR-PS-HC-246:setI", "SR-PS-HC-247:setI", "SR-PS-VC-011:setI", "SR-PS-VC-012:setI", "SR-PS-VC-013:setI", "SR-PS-VC-014:setI", "SR-PS-VC-015:setI", "SR-PS-VC-016:setI", "SR-PS-VC-017:setI", "SR-PS-VC-021:setI", "SR-PS-VC-022:setI", "SR-PS-VC-023:setI", "SR-PS-VC-024:setI", "SR-PS-VC-025:setI", "SR-PS-VC-026:setI", "SR-PS-VC-027:setI", "SR-PS-VC-031:setI", "SR-PS-VC-032:setI", "SR-PS-VC-033:setI", "SR-PS-VC-034:setI", "SR-PS-VC-035:setI", "SR-PS-VC-036:setI", "SR-PS-VC-037:setI", "SR-PS-VC-041:setI", "SR-PS-VC-042:setI", "SR-PS-VC-043:setI", "SR-PS-VC-044:setI", "SR-PS-VC-045:setI", "SR-PS-VC-046:setI", "SR-PS-VC-047:setI", "SR-PS-VC-051:setI", "SR-PS-VC-052:setI", "SR-PS-VC-053:setI", "SR-PS-VC-054:setI", "SR-PS-VC-055:setI", "SR-PS-VC-056:setI", "SR-PS-VC-057:setI", "SR-PS-VC-061:setI", "SR-PS-VC-062:setI", "SR-PS-VC-063:setI", "SR-PS-VC-064:setI", "SR-PS-VC-065:setI", "SR-PS-VC-066:setI", "SR-PS-VC-067:setI", "SR-PS-VC-071:setI", "SR-PS-VC-072:setI", "SR-PS-VC-073:setI", "SR-PS-VC-074:setI", "SR-PS-VC-075:setI", "SR-PS-VC-076:setI", "SR-PS-VC-077:setI", "SR-PS-VC-081:setI", "SR-PS-VC-082:setI", "SR-PS-VC-083:setI", "SR-PS-VC-084:setI", "SR-PS-VC-085:setI", "SR-PS-VC-086:setI", "SR-PS-VC-087:setI", "SR-PS-VC-091:setI", "SR-PS-VC-092:setI", "SR-PS-VC-093:setI", "SR-PS-VC-094:setI", "SR-PS-VC-095:setI", "SR-PS-VC-096:setI", "SR-PS-VC-097:setI", "SR-PS-VC-101:setI", "SR-PS-VC-102:setI", "SR-PS-VC-103:setI", "SR-PS-VC-104:setI", "SR-PS-VC-105:setI", "SR-PS-VC-106:setI", "SR-PS-VC-107:setI", "SR-PS-VC-111:setI", "SR-PS-VC-112:setI", "SR-PS-VC-113:setI", "SR-PS-VC-114:setI", "SR-PS-VC-115:setI", "SR-PS-VC-116:setI", "SR-PS-VC-117:setI", "SR-PS-VC-121:setI", "SR-PS-VC-122:setI", "SR-PS-VC-123:setI", "SR-PS-VC-124:setI", "SR-PS-VC-125:setI", "SR-PS-VC-126:setI", "SR-PS-VC-127:setI", "SR-PS-VC-131:setI", "SR-PS-VC-132:setI", "SR-PS-VC-133:setI", "SR-PS-VC-134:setI", "SR-PS-VC-135:setI", "SR-PS-VC-136:setI", "SR-PS-VC-137:setI", "SR-PS-VC-141:setI", "SR-PS-VC-142:setI", "SR-PS-VC-143:setI", "SR-PS-VC-144:setI", "SR-PS-VC-145:setI", "SR-PS-VC-146:setI", "SR-PS-VC-147:setI", "SR-PS-VC-151:setI", "SR-PS-VC-152:setI", "SR-PS-VC-153:setI", "SR-PS-VC-154:setI", "SR-PS-VC-155:setI", "SR-PS-VC-156:setI", "SR-PS-VC-157:setI", "SR-PS-VC-161:setI", "SR-PS-VC-162:setI", "SR-PS-VC-163:setI", "SR-PS-VC-164:setI", "SR-PS-VC-165:setI", "SR-PS-VC-166:setI", "SR-PS-VC-167:setI", "SR-PS-VC-171:setI", "SR-PS-VC-172:setI", "SR-PS-VC-173:setI", "SR-PS-VC-174:setI", "SR-PS-VC-175:setI", "SR-PS-VC-176:setI", "SR-PS-VC-177:setI", "SR-PS-VC-181:setI", "SR-PS-VC-182:setI", "SR-PS-VC-183:setI", "SR-PS-VC-184:setI", "SR-PS-VC-185:setI", "SR-PS-VC-186:setI", "SR-PS-VC-187:setI", "SR-PS-VC-191:setI", "SR-PS-VC-192:setI", "SR-PS-VC-193:setI", "SR-PS-VC-194:setI", "SR-PS-VC-195:setI", "SR-PS-VC-196:setI", "SR-PS-VC-197:setI", "SR-PS-VC-201:setI", "SR-PS-VC-202:setI", "SR-PS-VC-203:setI", "SR-PS-VC-204:setI", "SR-PS-VC-205:setI", "SR-PS-VC-206:setI", "SR-PS-VC-207:setI", "SR-PS-VC-211:setI", "SR-PS-VC-212:setI", "SR-PS-VC-213:setI", "SR-PS-VC-214:setI", "SR-PS-VC-215:setI", "SR-PS-VC-216:setI", "SR-PS-VC-217:setI", "SR-PS-VC-221:setI", "SR-PS-VC-222:setI", "SR-PS-VC-223:setI", "SR-PS-VC-224:setI", "SR-PS-VC-225:setI", "SR-PS-VC-226:setI", "SR-PS-VC-227:setI", "SR-PS-VC-231:setI", "SR-PS-VC-232:setI", "SR-PS-VC-233:setI", "SR-PS-VC-234:setI", "SR-PS-VC-235:setI", "SR-PS-VC-236:setI", "SR-PS-VC-237:setI", "SR-PS-VC-241:setI", "SR-PS-VC-242:setI", "SR-PS-VC-243:setI", "SR-PS-VC-244:setI", "SR-PS-VC-245:setI", "SR-PS-VC-246:setI", "SR-PS-VC-247:setI", "SR-PS-QL1-0101:setI", "SR-PS-QL2-0102:setI", "SR-PS-QL3-0103:setI", "SR-PS-QS4-0104:setI", "SR-PS-QS5-0105:setI", "SR-PS-QS5-0106:setI", "SR-PS-QS4-0107:setI", "SR-PS-QS3-0108:setI", "SR-PS-QS2-0109:setI", "SR-PS-QS1-0110:setI", "SR-PS-QS1-0201:setI", "SR-PS-QS2-0202:setI", "SR-PS-QS3-0203:setI", "SR-PS-QS4-0204:setI", "SR-PS-QS5-0205:setI", "SR-PS-QS5-0206:setI", "SR-PS-QS4-0207:setI", "SR-PS-QS3-0208:setI", "SR-PS-QS2-0209:setI", "SR-PS-QS1-0210:setI", "SR-PS-QS1-0301:setI", "SR-PS-QS2-0302:setI", "SR-PS-QS3-0303:setI", "SR-PS-QS4-0304:setI", "SR-PS-QS5-0305:setI", "SR-PS-QS5-0306:setI", "SR-PS-QS4-0307:setI", "SR-PS-QS3-0308:setI", "SR-PS-QS2-0309:setI", "SR-PS-QS1-0310:setI", "SR-PS-QS1-0401:setI", "SR-PS-QS2-0402:setI", "SR-PS-QS3-0403:setI", "SR-PS-QS4-0404:setI", "SR-PS-QS5-0405:setI", "SR-PS-QS5-0406:setI", "SR-PS-QS4-0407:setI", "SR-PS-QL3-0408:setI", "SR-PS-QL2-0409:setI", "SR-PS-QL1-0410:setI", "SR-PS-QL1-0501:setI", "SR-PS-QL2-0502:setI", "SR-PS-QL3-0503:setI", "SR-PS-QS4-0504:setI", "SR-PS-QS5-0505:setI", "SR-PS-QS5-0506:setI", "SR-PS-QS4-0507:setI", "SR-PS-QS3-0508:setI", "SR-PS-QS2-0509:setI", "SR-PS-QS1-0510:setI", "SR-PS-QS1-0601:setI", "SR-PS-QS2-0602:setI", "SR-PS-QS3-0603:setI", "SR-PS-QS4-0604:setI", "SR-PS-QS5-0605:setI", "SR-PS-QS5-0606:setI", "SR-PS-QS4-0607:setI", "SR-PS-QS3-0608:setI", "SR-PS-QS2-0609:setI", "SR-PS-QS1-0610:setI", "SR-PS-QS1-0701:setI", "SR-PS-QS2-0702:setI", "SR-PS-QS3-0703:setI", "SR-PS-QS4-0704:setI", "SR-PS-QS5-0705:setI", "SR-PS-QS5-0706:setI", "SR-PS-QS4-0707:setI", "SR-PS-QS3-0708:setI", "SR-PS-QS2-0709:setI", "SR-PS-QS1-0710:setI", "SR-PS-QS1-0801:setI", "SR-PS-QS2-0802:setI", "SR-PS-QS3-0803:setI", "SR-PS-QS4-0804:setI", "SR-PS-QS5-0805:setI", "SR-PS-QS5-0806:setI", "SR-PS-QS4-0807:setI", "SR-PS-QL3-0808:setI", "SR-PS-QL2-0809:setI", "SR-PS-QL1-0810:setI", "SR-PS-QL1-0901:setI", "SR-PS-QL2-0902:setI", "SR-PS-QL3-0903:setI", "SR-PS-QS4-0904:setI", "SR-PS-QS5-0905:setI", "SR-PS-QS5-0906:setI", "SR-PS-QS4-0907:setI", "SR-PS-QS3-0908:setI", "SR-PS-QS2-0909:setI", "SR-PS-QS1-0910:setI", "SR-PS-QS1-1001:setI", "SR-PS-QS2-1002:setI", "SR-PS-QS3-1003:setI", "SR-PS-QS4-1004:setI", "SR-PS-QS5-1005:setI", "SR-PS-QS5-1006:setI", "SR-PS-QS4-1007:setI", "SR-PS-QS3-1008:setI", "SR-PS-QS2-1009:setI", "SR-PS-QS1-1010:setI", "SR-PS-QS1-1101:setI", "SR-PS-QS2-1102:setI", "SR-PS-QS3-1103:setI", "SR-PS-QS4-1104:setI", "SR-PS-QS5-1105:setI", "SR-PS-QS5-1106:setI", "SR-PS-QS4-1107:setI", "SR-PS-QS3-1108:setI", "SR-PS-QS2-1109:setI", "SR-PS-QS1-1110:setI", "SR-PS-QS1-1201:setI", "SR-PS-QS2-1202:setI", "SR-PS-QS3-1203:setI", "SR-PS-QS4-1204:setI", "SR-PS-QS5-1205:setI", "SR-PS-QS5-1206:setI", "SR-PS-QS4-1207:setI", "SR-PS-QL3-1208:setI", "SR-PS-QL2-1209:setI", "SR-PS-QL1-1210:setI", "SR-PS-QL1-1301:setI", "SR-PS-QL2-1302:setI", "SR-PS-QL3-1303:setI", "SR-PS-QS4-1304:setI", "SR-PS-QS5-1305:setI", "SR-PS-QS5-1306:setI", "SR-PS-QS4-1307:setI", "SR-PS-QS3-1308:setI", "SR-PS-QS2-1309:setI", "SR-PS-QS1-1310:setI", "SR-PS-QS1-1401:setI", "SR-PS-QS2-1402:setI", "SR-PS-QS3-1403:setI", "SR-PS-QS4-1404:setI", "SR-PS-QS5-1405:setI", "SR-PS-QS5-1406:setI", "SR-PS-QS4-1407:setI", "SR-PS-QS3-1408:setI", "SR-PS-QS2-1409:setI", "SR-PS-QS1-1410:setI", "SR-PS-QS1-1501:setI", "SR-PS-QS2-1502:setI", "SR-PS-QS3-1503:setI", "SR-PS-QS4-1504:setI", "SR-PS-QS5-1505:setI", "SR-PS-QS5-1506:setI", "SR-PS-QS4-1507:setI", "SR-PS-QS3-1508:setI", "SR-PS-QS2-1509:setI", "SR-PS-QS1-1510:setI", "SR-PS-QS1-1601:setI", "SR-PS-QS2-1602:setI", "SR-PS-QS3-1603:setI", "SR-PS-QS4-1604:setI", "SR-PS-QS5-1605:setI", "SR-PS-QS5-1606:setI", "SR-PS-QS4-1607:setI", "SR-PS-QL3-1608:setI", "SR-PS-QL2-1609:setI", "SR-PS-QL1-1610:setI", "SR-PS-QL1-1701:setI", "SR-PS-QL2-1702:setI", "SR-PS-QL3-1703:setI", "SR-PS-QS4-1704:setI", "SR-PS-QS5-1705:setI", "SR-PS-QS5-1706:setI", "SR-PS-QS4-1707:setI", "SR-PS-QS3-1708:setI", "SR-PS-QS2-1709:setI", "SR-PS-QS1-1710:setI", "SR-PS-QS1-1801:setI", "SR-PS-QS2-1802:setI", "SR-PS-QS3-1803:setI", "SR-PS-QS4-1804:setI", "SR-PS-QS5-1805:setI", "SR-PS-QS5-1806:setI", "SR-PS-QS4-1807:setI", "SR-PS-QS3-1808:setI", "SR-PS-QS2-1809:setI", "SR-PS-QS1-1810:setI", "SR-PS-QS1-1901:setI", "SR-PS-QS2-1902:setI", "SR-PS-QS3-1903:setI", "SR-PS-QS4-1904:setI", "SR-PS-QS5-1905:setI", "SR-PS-QS5-1906:setI", "SR-PS-QS4-1907:setI", "SR-PS-QS3-1908:setI", "SR-PS-QS2-1909:setI", "SR-PS-QS1-1910:setI", "SR-PS-QS1-2001:setI", "SR-PS-QS2-2002:setI", "SR-PS-QS3-2003:setI", "SR-PS-QS4-2004:setI", "SR-PS-QS5-2005:setI", "SR-PS-QS5-2006:setI", "SR-PS-QS4-2007:setI", "SR-PS-QL3-2008:setI", "SR-PS-QL2-2009:setI", "SR-PS-QL1-2010:setI", "SR-PS-QL1-2101:setI", "SR-PS-QL2-2102:setI", "SR-PS-QL3-2103:setI", "SR-PS-QS4-2104:setI", "SR-PS-QS5-2105:setI", "SR-PS-QS5-2106:setI", "SR-PS-QS4-2107:setI", "SR-PS-QS3-2108:setI", "SR-PS-QS2-2109:setI", "SR-PS-QS1-2110:setI", "SR-PS-QS1-2201:setI", "SR-PS-QS2-2202:setI", "SR-PS-QS3-2203:setI", "SR-PS-QS4-2204:setI", "SR-PS-QS5-2205:setI", "SR-PS-QS5-2206:setI", "SR-PS-QS4-2207:setI", "SR-PS-QS3-2208:setI", "SR-PS-QS2-2209:setI", "SR-PS-QS1-2210:setI", "SR-PS-QS1-2301:setI", "SR-PS-QS2-2302:setI", "SR-PS-QS3-2303:setI", "SR-PS-QS4-2304:setI", "SR-PS-QS5-2305:setI", "SR-PS-QS5-2306:setI", "SR-PS-QS4-2307:setI", "SR-PS-QS3-2308:setI", "SR-PS-QS2-2309:setI", "SR-PS-QS1-2310:setI", "SR-PS-QS1-2401:setI", "SR-PS-QS2-2402:setI", "SR-PS-QS3-2403:setI", "SR-PS-QS4-2404:setI", "SR-PS-QS5-2405:setI", "SR-PS-QS5-2406:setI", "SR-PS-QS4-2407:setI", "SR-PS-QL3-2408:setI", "SR-PS-QL2-2409:setI", "SR-PS-QL1-2410:setI", "SR-PS-S1-011:setI", "SR-PS-S2-012:setI", "SR-PS-SD-013:setI", "SR-PS-SF-014:setI", "SR-PS-SD-015:setI", "SR-PS-S4-016:setI", "SR-PS-S3-017:setI", "SR-PS-S5-021:setI", "SR-PS-S6-022:setI", "SR-PS-SD-023:setI", "SR-PS-SF-024:setI", "SR-PS-SD-025:setI", "SR-PS-S6-026:setI", "SR-PS-S5-027:setI", "SR-PS-S5-031:setI", "SR-PS-S6-032:setI", "SR-PS-SD-033:setI", "SR-PS-SF-034:setI", "SR-PS-SD-035:setI", "SR-PS-S6-036:setI", "SR-PS-S5-037:setI", "SR-PS-S3-041:setI", "SR-PS-S4-042:setI", "SR-PS-SD-043:setI", "SR-PS-SF-044:setI", "SR-PS-SD-045:setI", "SR-PS-S2-046:setI", "SR-PS-S1-047:setI", "SR-PS-S1-051:setI", "SR-PS-S2-052:setI", "SR-PS-SD-053:setI", "SR-PS-SF-054:setI", "SR-PS-SD-055:setI", "SR-PS-S4-056:setI", "SR-PS-S3-057:setI", "SR-PS-S5-061:setI", "SR-PS-S6-062:setI", "SR-PS-SD-063:setI", "SR-PS-SF-064:setI", "SR-PS-SD-065:setI", "SR-PS-S6-066:setI", "SR-PS-S5-067:setI", "SR-PS-S5-071:setI", "SR-PS-S6-072:setI", "SR-PS-SD-073:setI", "SR-PS-SF-074:setI", "SR-PS-SD-075:setI", "SR-PS-S6-076:setI", "SR-PS-S5-077:setI", "SR-PS-S3-081:setI", "SR-PS-S4-082:setI", "SR-PS-SD-083:setI", "SR-PS-SF-084:setI", "SR-PS-SD-085:setI", "SR-PS-S2-086:setI", "SR-PS-S1-087:setI", "SR-PS-S1-091:setI", "SR-PS-S2-092:setI", "SR-PS-SD-093:setI", "SR-PS-SF-094:setI", "SR-PS-SD-095:setI", "SR-PS-S4-096:setI", "SR-PS-S3-097:setI", "SR-PS-S5-101:setI", "SR-PS-S6-102:setI", "SR-PS-SD-103:setI", "SR-PS-SF-104:setI", "SR-PS-SD-105:setI", "SR-PS-S6-106:setI", "SR-PS-S5-107:setI", "SR-PS-S5-111:setI", "SR-PS-S6-112:setI", "SR-PS-SD-113:setI", "SR-PS-SF-114:setI", "SR-PS-SD-115:setI", "SR-PS-S6-116:setI", "SR-PS-S5-117:setI", "SR-PS-S3-121:setI", "SR-PS-S4-122:setI", "SR-PS-SD-123:setI", "SR-PS-SF-124:setI", "SR-PS-SD-125:setI", "SR-PS-S2-126:setI", "SR-PS-S1-127:setI", "SR-PS-S1-131:setI", "SR-PS-S2-132:setI", "SR-PS-SD-133:setI", "SR-PS-SF-134:setI", "SR-PS-SD-135:setI", "SR-PS-S4-136:setI", "SR-PS-S3-137:setI", "SR-PS-S5-141:setI", "SR-PS-S6-142:setI", "SR-PS-SD-143:setI", "SR-PS-SF-144:setI", "SR-PS-SD-145:setI", "SR-PS-S6-146:setI", "SR-PS-S5-147:setI", "SR-PS-S5-151:setI", "SR-PS-S6-152:setI", "SR-PS-SD-153:setI", "SR-PS-SF-154:setI", "SR-PS-SD-155:setI", "SR-PS-S6-156:setI", "SR-PS-S5-157:setI", "SR-PS-S3-161:setI", "SR-PS-S4-162:setI", "SR-PS-SD-163:setI", "SR-PS-SF-164:setI", "SR-PS-SD-165:setI", "SR-PS-S2-166:setI", "SR-PS-S1-167:setI", "SR-PS-S1-171:setI", "SR-PS-S2-172:setI", "SR-PS-SD-173:setI", "SR-PS-SF-174:setI", "SR-PS-SD-175:setI", "SR-PS-S4-176:setI", "SR-PS-S3-177:setI", "SR-PS-S5-181:setI", "SR-PS-S6-182:setI", "SR-PS-SD-183:setI", "SR-PS-SF-184:setI", "SR-PS-SD-185:setI", "SR-PS-S6-186:setI", "SR-PS-S5-187:setI", "SR-PS-S5-191:setI", "SR-PS-S6-192:setI", "SR-PS-SD-193:setI", "SR-PS-SF-194:setI", "SR-PS-SD-195:setI", "SR-PS-S6-196:setI", "SR-PS-S5-197:setI", "SR-PS-S3-201:setI", "SR-PS-S4-202:setI", "SR-PS-SD-203:setI", "SR-PS-SF-204:setI", "SR-PS-SD-205:setI", "SR-PS-S2-206:setI", "SR-PS-S1-207:setI", "SR-PS-S1-211:setI", "SR-PS-S2-212:setI", "SR-PS-SD-213:setI", "SR-PS-SF-214:setI", "SR-PS-SD-215:setI", "SR-PS-S4-216:setI", "SR-PS-S3-217:setI", "SR-PS-S5-221:setI", "SR-PS-S6-222:setI", "SR-PS-SD-223:setI", "SR-PS-SF-224:setI", "SR-PS-SD-225:setI", "SR-PS-S6-226:setI", "SR-PS-S5-227:setI", "SR-PS-S5-231:setI", "SR-PS-S6-232:setI", "SR-PS-SD-233:setI", "SR-PS-SF-234:setI", "SR-PS-SD-235:setI", "SR-PS-S6-236:setI", "SR-PS-S5-237:setI", "SR-PS-S3-241:setI", "SR-PS-S4-242:setI", "SR-PS-SD-243:setI", "SR-PS-SF-244:setI", "SR-PS-SD-245:setI", "SR-PS-S2-246:setI", "SR-PS-S1-247:setI", "SR-PS-SKEW-011:setI", "SR-PS-SKEW-012:setI", "SR-PS-SKEW-013:setI", "SR-PS-SKEW-014:setI", "SR-PS-SKEW-015:setI", "SR-PS-SKEW-016:setI", "SR-PS-SKEW-017:setI", "SR-PS-SKEW-021:setI", "SR-PS-SKEW-022:setI", "SR-PS-SKEW-023:setI", "SR-PS-SKEW-024:setI", "SR-PS-SKEW-025:setI", "SR-PS-SKEW-026:setI", "SR-PS-SKEW-027:setI", "SR-PS-SKEW-031:setI", "SR-PS-SKEW-032:setI", "SR-PS-SKEW-033:setI", "SR-PS-SKEW-034:setI", "SR-PS-SKEW-035:setI", "SR-PS-SKEW-036:setI", "SR-PS-SKEW-037:setI", "SR-PS-SKEW-041:setI", "SR-PS-SKEW-042:setI", "SR-PS-SKEW-043:setI", "SR-PS-SKEW-044:setI", "SR-PS-SKEW-045:setI", "SR-PS-SKEW-046:setI", "SR-PS-SKEW-047:setI", "SR-PS-SKEW-051:setI", "SR-PS-SKEW-052:setI", "SR-PS-SKEW-053:setI", "SR-PS-SKEW-054:setI", "SR-PS-SKEW-055:setI", "SR-PS-SKEW-056:setI", "SR-PS-SKEW-057:setI", "SR-PS-SKEW-061:setI", "SR-PS-SKEW-062:setI", "SR-PS-SKEW-063:setI", "SR-PS-SKEW-064:setI", "SR-PS-SKEW-065:setI", "SR-PS-SKEW-066:setI", "SR-PS-SKEW-067:setI", "SR-PS-SKEW-071:setI", "SR-PS-SKEW-072:setI", "SR-PS-SKEW-073:setI", "SR-PS-SKEW-074:setI", "SR-PS-SKEW-075:setI", "SR-PS-SKEW-076:setI", "SR-PS-SKEW-077:setI", "SR-PS-SKEW-081:setI", "SR-PS-SKEW-082:setI", "SR-PS-SKEW-083:setI", "SR-PS-SKEW-084:setI", "SR-PS-SKEW-085:setI", "SR-PS-SKEW-086:setI", "SR-PS-SKEW-087:setI", "SR-PS-SKEW-091:setI", "SR-PS-SKEW-092:setI", "SR-PS-SKEW-093:setI", "SR-PS-SKEW-094:setI", "SR-PS-SKEW-095:setI", "SR-PS-SKEW-096:setI", "SR-PS-SKEW-097:setI", "SR-PS-SKEW-101:setI", "SR-PS-SKEW-102:setI", "SR-PS-SKEW-103:setI", "SR-PS-SKEW-104:setI", "SR-PS-SKEW-105:setI", "SR-PS-SKEW-106:setI", "SR-PS-SKEW-107:setI", "SR-PS-SKEW-111:setI", "SR-PS-SKEW-112:setI", "SR-PS-SKEW-113:setI", "SR-PS-SKEW-114:setI", "SR-PS-SKEW-115:setI", "SR-PS-SKEW-116:setI", "SR-PS-SKEW-117:setI", "SR-PS-SKEW-121:setI", "SR-PS-SKEW-122:setI", "SR-PS-SKEW-123:setI", "SR-PS-SKEW-124:setI", "SR-PS-SKEW-125:setI", "SR-PS-SKEW-126:setI", "SR-PS-SKEW-127:setI", "SR-PS-SKEW-131:setI", "SR-PS-SKEW-132:setI", "SR-PS-SKEW-133:setI", "SR-PS-SKEW-134:setI", "SR-PS-SKEW-135:setI", "SR-PS-SKEW-136:setI", "SR-PS-SKEW-137:setI", "SR-PS-SKEW-141:setI", "SR-PS-SKEW-142:setI", "SR-PS-SKEW-143:setI", "SR-PS-SKEW-144:setI", "SR-PS-SKEW-145:setI", "SR-PS-SKEW-146:setI", "SR-PS-SKEW-147:setI", "SR-PS-SKEW-151:setI", "SR-PS-SKEW-152:setI", "SR-PS-SKEW-153:setI", "SR-PS-SKEW-154:setI", "SR-PS-SKEW-155:setI", "SR-PS-SKEW-156:setI", "SR-PS-SKEW-157:setI", "SR-PS-SKEW-161:setI", "SR-PS-SKEW-162:setI", "SR-PS-SKEW-163:setI", "SR-PS-SKEW-164:setI", "SR-PS-SKEW-165:setI", "SR-PS-SKEW-166:setI", "SR-PS-SKEW-167:setI", "SR-PS-SKEW-171:setI", "SR-PS-SKEW-172:setI", "SR-PS-SKEW-173:setI", "SR-PS-SKEW-174:setI", "SR-PS-SKEW-175:setI", "SR-PS-SKEW-176:setI", "SR-PS-SKEW-177:setI", "SR-PS-SKEW-181:setI", "SR-PS-SKEW-182:setI", "SR-PS-SKEW-183:setI", "SR-PS-SKEW-184:setI", "SR-PS-SKEW-185:setI", "SR-PS-SKEW-186:setI", "SR-PS-SKEW-187:setI", "SR-PS-SKEW-191:setI", "SR-PS-SKEW-192:setI", "SR-PS-SKEW-193:setI", "SR-PS-SKEW-194:setI", "SR-PS-SKEW-195:setI", "SR-PS-SKEW-196:setI", "SR-PS-SKEW-197:setI", "SR-PS-SKEW-201:setI", "SR-PS-SKEW-202:setI", "SR-PS-SKEW-203:setI", "SR-PS-SKEW-204:setI", "SR-PS-SKEW-205:setI", "SR-PS-SKEW-206:setI", "SR-PS-SKEW-207:setI", "SR-PS-SKEW-211:setI", "SR-PS-SKEW-212:setI", "SR-PS-SKEW-213:setI", "SR-PS-SKEW-214:setI", "SR-PS-SKEW-215:setI", "SR-PS-SKEW-216:setI", "SR-PS-SKEW-217:setI", "SR-PS-SKEW-221:setI", "SR-PS-SKEW-222:setI", "SR-PS-SKEW-223:setI", "SR-PS-SKEW-224:setI", "SR-PS-SKEW-225:setI", "SR-PS-SKEW-226:setI", "SR-PS-SKEW-227:setI", "SR-PS-SKEW-231:setI", "SR-PS-SKEW-232:setI", "SR-PS-SKEW-233:setI", "SR-PS-SKEW-234:setI", "SR-PS-SKEW-235:setI", "SR-PS-SKEW-236:setI", "SR-PS-SKEW-237:setI", "SR-PS-SKEW-241:setI", "SR-PS-SKEW-242:setI", "SR-PS-SKEW-243:setI", "SR-PS-SKEW-244:setI", "SR-PS-SKEW-245:setI", "SR-PS-SKEW-246:setI", "SR-PS-SKEW-247:setI", "SR-RF2-LLRF:setGapVoltage", "SR-RF2-LLRF:setStationPhase", "SR-RF3-LLRF:setGapVoltage", "SR-RF3-LLRF:setStationPhase", "SR-PS-DMB09-Q1:setI", "SR-PS-DMB09-Q2:setI", "SR-PS-DMB09-Q3:setI", "SR-PS-DMB25-Q1:setI", "SR-PS-DMB25-Q2:setI", "SR-PS-DMB25-Q3:setI", "SR-PS-DMB41-Q1:setI", "SR-PS-DMB41-Q2:setI", "SR-PS-DMB41-Q3:setI", "SR-PS-DMB09-HC1:setI", "SR-PS-DMB09-HC2:setI", "SR-PS-DMB09-VC1:setI", "SR-PS-DMB09-VC2:setI", "SR-PS-DMB25-HC1:setI", "SR-PS-DMB25-HC2:setI", "SR-PS-DMB25-VC1:setI", "SR-PS-DMB25-VC2:setI", "SR-PS-DMB41-HC1:setI", "SR-PS-DMB41-HC2:setI", "SR-PS-DMB41-VC1:setI", "SR-PS-DMB41-VC2:setI", "SR-ID-IU22-05:setGap", "SR-ID-IU22A-09:setGap", "SR-ID-IU22B-09:setGap", "SR-ID-IUT22-21:setGap", "SR-ID-IU22-23:setGap", "SR-ID-IU22A-25:setGap", "SR-ID-IU22B-25:setGap", "SR-ID-EPU48A-41:setGap", "SR-ID-EPU48A-41:setPhase", "SR-ID-EPU48B-41:setGap", "SR-ID-EPU48B-41:setPhase", "SR-ID-EPU46-45:setGap", "SR-ID-EPU46-45:setPhase", "SR-ID-IUT22-21:setGapTaper", "SR-ID-EPU48PS-41:setGap", "SR-ID-IU22-05:gapMotorOff", "SR-ID-IU22A-09:gapMotorOff", "SR-ID-IU22B-09:gapMotorOff", "SR-ID-IUT22-21:gapMotorOff", "SR-ID-IU22-23:gapMotorOff", "SR-ID-IU22A-25:gapMotorOff", "SR-ID-IU22B-25:gapMotorOff", "SR-ID-EPU48A-41:gapMotorOff", "SR-ID-EPU48B-41:gapMotorOff", "SR-ID-EPU46-45:gapMotorOff", "SR-ID-EPU48A-41:phaseMotorOff", "SR-ID-EPU48B-41:phaseMotorOff", "SR-ID-EPU46-45:phaseMotorOff", "SR-DI-FOFB-H:setStatus", "SR-DI-FOFB-V:setStatus", "IGPF:TPSX:FBCTRL", "IGPF:TPSY:FBCTRL", "TPS-SR-022:bpm3:ilk:enabled", "SR-DI-ANGLE-ILK:StatusX", "SR-DI-ANGLE-ILK:StatusY", "SR-DI-RF-FB:setStatus", "SR-ID-EPU48-TFF:status", "SR-ID-EPU48-CFF:status", "SR-ID-EPU46-TFF:status", "SR-ID-EPU46-CFF:status", "TI-INJ-PROC:TopupHiLowStart"]
  out "result":string="Beam Trip Events \nTatal Counts: 0"
  in  "last ? Hrs":dbl=12.0 min=1.0 max=24.0 step=1.0
  in  "Trip Evt B":bool
  in  "Show Check list Button":bool=TRUE
  in  "View Diff Button":bool
  in  "Save Lattice Button":bool
  in  "Refresh B":bool
  out "x = y?":bool
  out "NOW time":string="15:45:10"
  out "NOW date":string="2017/10/28"
  in  "Save Button":bool
  out "error out 3":errorcluster
  in  "stop":bool
  out "time kickeron":string="15:43:52"
  out "date kickeron":string="2017/10/28"
  out "Orbit ILK(A)":bool
  out "Orbit INT. Ang Active":bool
  out "Orbit INT.Ang. On":bool
  out "Orbit INT. Pos Active":bool
  out "Orbit INT.Pos. On":bool
  in  "Copy Button":bool
  in  "Print Button":bool
  in  "Help Button":bool
  in  "Open Button":bool
  # "TPS OP Handover Information"
  # "Others"
  # "Additional Functions"
  # "Time："
  # "follow"
  # "歷史電流圖\ntrip次數?\n輻射劑量?\n平均氣壓\n目前最高累計劑量\n最近一次觸發時BR電流及WCM數值"
  # "Valve  Status"
  # "TFF"
  # "CFF"
  # "SM Status"
  # "TPS Operational Handover Information v1.5.0"
  # "SR Status"
  # "Feedback"
  # "Pulse Mag"
  # "LINAC"
  # "x8(ns)"
  # "x2(ns)"
  # "x0.01(ns)"
  # "RF Status"
  # "Hz"
  # "(kV)"
  # "(kV)"
  # "Changeliang@LOP.NSRRC"
  # "BR Fill Pattern"
  # "SR Fill Pattern"
  # "Lattice Files in Using"
  # "ID &Beamline [R]"
  # "Gap\nmm"
  # "Motor"
  # "Phase"
  # "FE/Hutch"
  # "Mode"
  # "Phase\nShifter"
  # "XBPM1X\num"
  # "XBPM1Y\num"
  # "XBPM2X\num"
  # "XBPM2Y\num"
  # "Note"
  # "05"
  # "09"
  # "Taper(enc)"
  # "21"
  # "23"
  # "25"
  # "41"
  # "45"
  # "SR Orbit"
  # "BPMX"
  # "BPMY"
  # "SR Beam Current History"
  # "ns"
  # "threshold:0.05mA"
  # "Adjusted History\n#Note: This file recorded PVs(set values) that were changed during this time.\n#(RF frequency was not recorded in this file)"
  # "Event Time"
  # "PV_name"
  # "Ori_Value"
  # "New_Value"
  # "hrs"
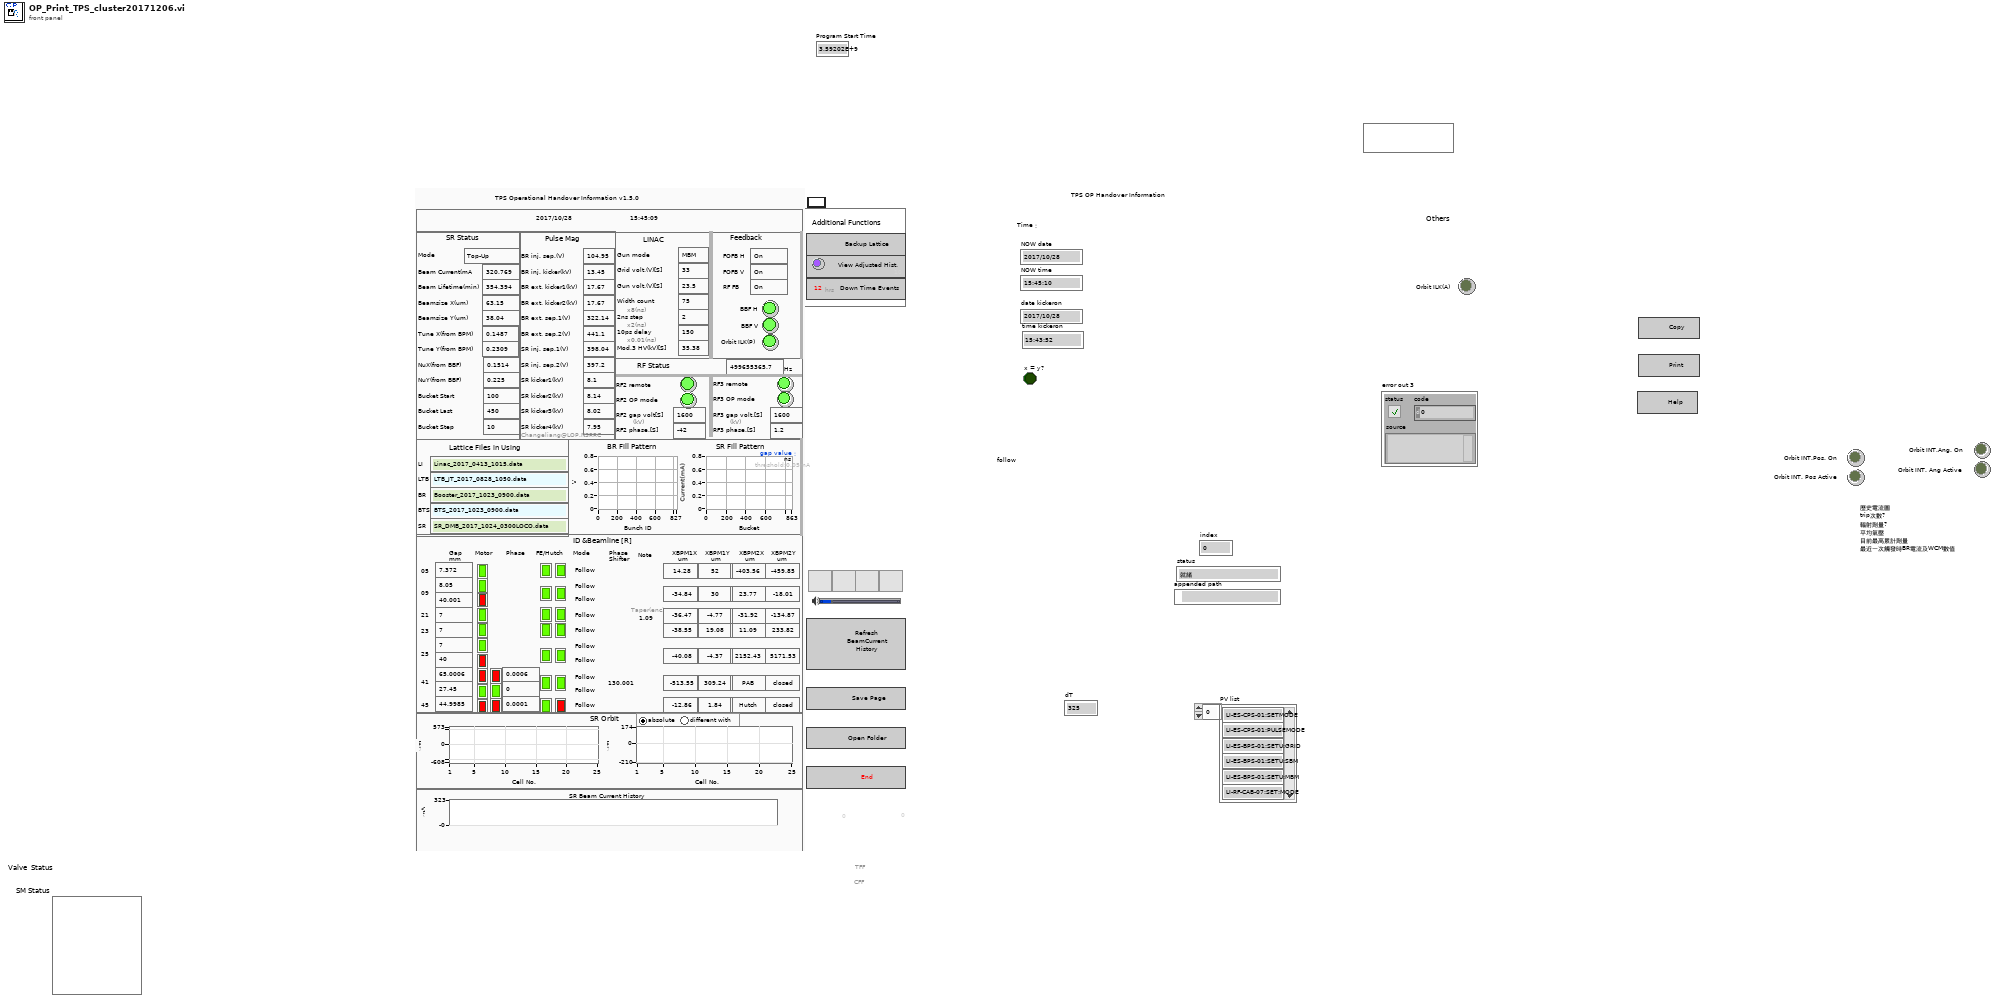
[diagram p1: front panel]
types:
  T1 = cluster{"SR Fill Pattern":dbl[], "Beam Current(mA":dbl, "Beam Lifetime(min)":dbl, "Beamsize X(um)":dbl, "Beamsize Y(um)":dbl, "Tune X(from BPM)":dbl, "Tune Y(from BPM)":dbl, "Mode":string, "NuX(from BBF) ":dbl, "NuY(from BBF)":dbl, "IU22-23gap(R)":dbl, "IU22-05gap(R)":dbl, "IU22-05M":bool, "IU22A-09gap(R)":dbl, "IU22A-09M":bool, "IU22B-09gap(R)":dbl, "IU22B-09M":bool, "IUT22-21gap(R)":dbl, "IUT22-21M":bool, "IU22-23M":bool, "IU22A-25gap(R)":dbl, "IU22A-25M":bool, "IU22B-25gap(R)":dbl, "IU22B-25M":bool, "EPU48A-41gap(R)":dbl, "EPU48A-41gM":bool, "EPU48B-41gap(R)":dbl, "EPU48B-41gM":bool, "EPU46-45gap(R)":dbl, "EPU46-45gM":bool, "EPU48A-41phase(R)":dbl, "EPU48B-41phase(R)":dbl, "EPU46-45phase(R)":dbl, "Grid volt.(V)[S]":dbl, "Gun mode":string, "Mod.3 HV(kV)[S]":dbl, "SR":string, "BR":string, "LI":string, "LTB":string, "BTS":string, "RF2 remote":bool, "RF2 OP mode":bool, "RF2 phase.[S]":dbl, "RF Freq.(s)":dbl, "RF2 gap volt[S]":dbl, "RF3 remote":bool, "RF3 OP mode":bool, "RF3 phase.[S]":dbl, "RF3 gap volt.[S]":dbl, "BBF V":bool, "BBF H":bool, "BR ext. kicker1(kV)":dbl, "BR ext. kicker2(kV)":dbl, "BR ext. sep.1(V)":dbl, "BR ext. sep.2(V)":dbl, "BR inj. sep.(V)":dbl, "BR inj. kicker(kV)":dbl, "SR kicker4(kV)":dbl, "SR kicker3(kV)":dbl, "SR kicker2(kV)":dbl, "SR kicker1(kV)":dbl, "SR inj. sep.2(V)":dbl, "SR inj. sep.1(V)":dbl, "Bucket Start":dbl, "Bucket Last":dbl, "Bucket Step":dbl, "Orbit ILK(P)":bool, "IU22-05 Hutch Enable":bool, "IU22A-09M Hutch Enable":bool, "IUT22-21M Hutch Enable":bool, "IU22-23M Hutch Enable":bool, "IU22A-25M Hutch Enable":bool, "EPU48A-41M Hutch Enable":bool, "EPU46-45M Hutch Enable":bool, "EPU46-45 FE Enable":bool, "EPU48A-41 FE Enable":bool, "IU22A-25 FE Enable":bool, "IU22-23 FE Enable":bool, "IUT22-21 FE Enable":bool, "IU22A-09 FE Enable":bool, "IU22-05 FE Enable":bool, "EPU48A-41pM":bool, "EPU48B-41pM":bool, "EPU46-45pM":bool, "Gun volt.(V)[S]":dbl, "Width count":dbl, "2ns step":dbl, "10ps delay":dbl, "phase shifter":dbl, "Taper":dbl, "05XBPMX 1":dbl, "09XBPMX 1":dbl, "21XBPMX 1":dbl, "23XBPMX 1":dbl, "25XBPMX 1":dbl, "41XBPMX 1":dbl, "45XBPMX 1":dbl, "05XBPMY 1":dbl, "09XBPMY 1":dbl, "21XBPMY 1":dbl, "23XBPMY 1":dbl, "25XBPMY 1":dbl, "41XBPMY 1":dbl, "45XBPMY 1":dbl, "FOFB H":string, "FOFB V":string, "time string":string, "date":string, "date (last kicker ON)":string, "time string (last kicker ON)":string, "Radio Buttons 2":enum32{"absolute", "different with"}, "09XBPMX 2":string, "09XBPMY 2":string, "05XBPMY 2":string, "05XBPMX 2":string, "21XBPMY 2":string, "21XBPMX 2":string, "23XBPMY 2":string, "23XBPMX 2":string, "25XBPMY 2":string, "25XBPMX 2":string, "41XBPMY 2":string, "41XBPMX 2":string, "45XBPMX 2":string, "45XBPMY 2":string, "05 mode":string, "09A mode":string, "09B mode":string, "21 mode":string, "23 mode":string, "25A mode":string, "25B mode":string, "41A mode":string, "41B mode":string, "46 mode":string, "BeamCurrent History":cluster{"BPM NO.  1_172":dbl[], dbl[]}, "SR Beam Current in            hours":dbl, "RF FB":string, "gap value：":i32, "BR Fill Pattern":dbl[], "time string (last INJ) ":string, "BPMX Graph 2":cluster{"Array of X axis  平均分配至各段":dbl[], dbl[]}, "BPMY Graph 2":cluster{"Array of X axis  平均分配至各段":dbl[], dbl[]}}
  T2 = typedef "NI_Database_API.lvlib/Conn ObjectReference.ctl" = refnum<k1>
  T3 = typedef "NI_Database_API.lvlib/Rec ObjectReference.ctl" = refnum<k1>
  T4 = typedef "imagedata.ctl" = cluster{"image type":i32, "image depth":i32, "image":u8[], "mask":u8[], "colors":u32[], "Rectangle":cluster{"left":i16, "top":i16, "right":i16, "bottom":i16}}
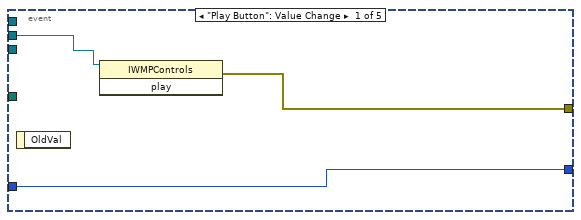
[diagram p3: hidden frame]
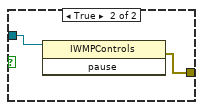
[diagram p4: hidden frame]
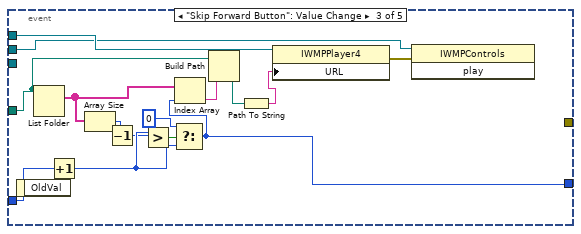
[diagram p5: hidden frame]
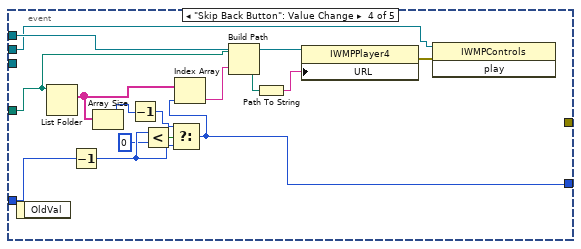
[diagram p6: hidden frame]
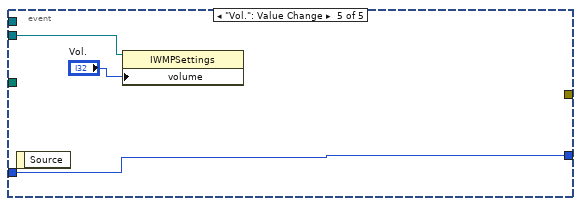
[diagram p7: hidden frame]
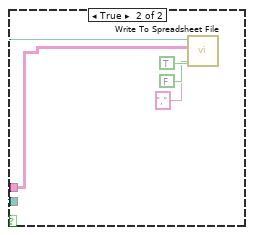
[diagram p8: hidden frame]
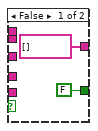
[diagram p11: hidden frame]
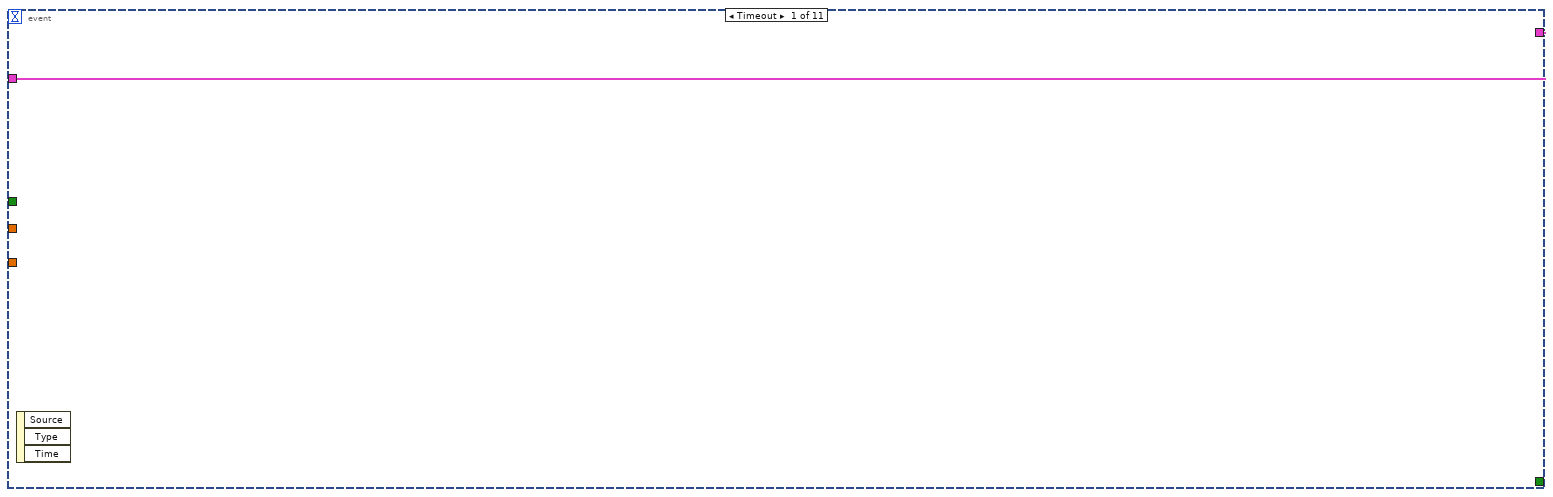
[diagram p15: hidden frame]
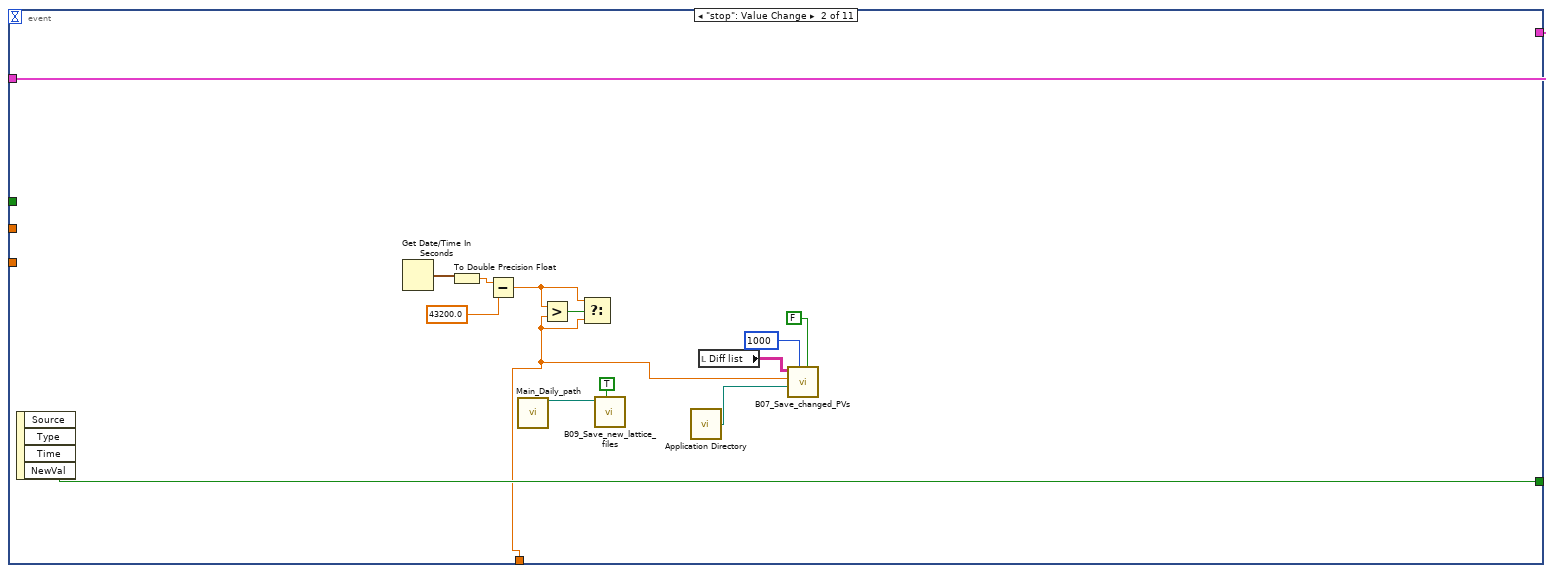
[diagram p16: hidden frame]
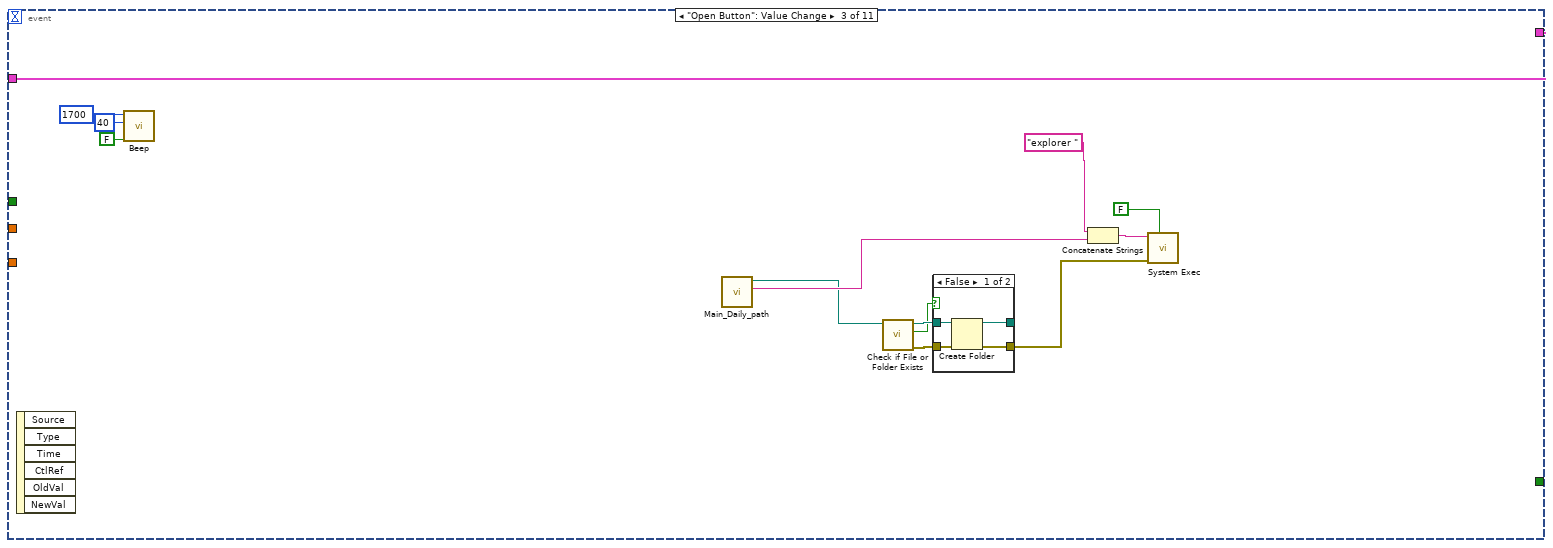
[diagram p17: hidden frame]
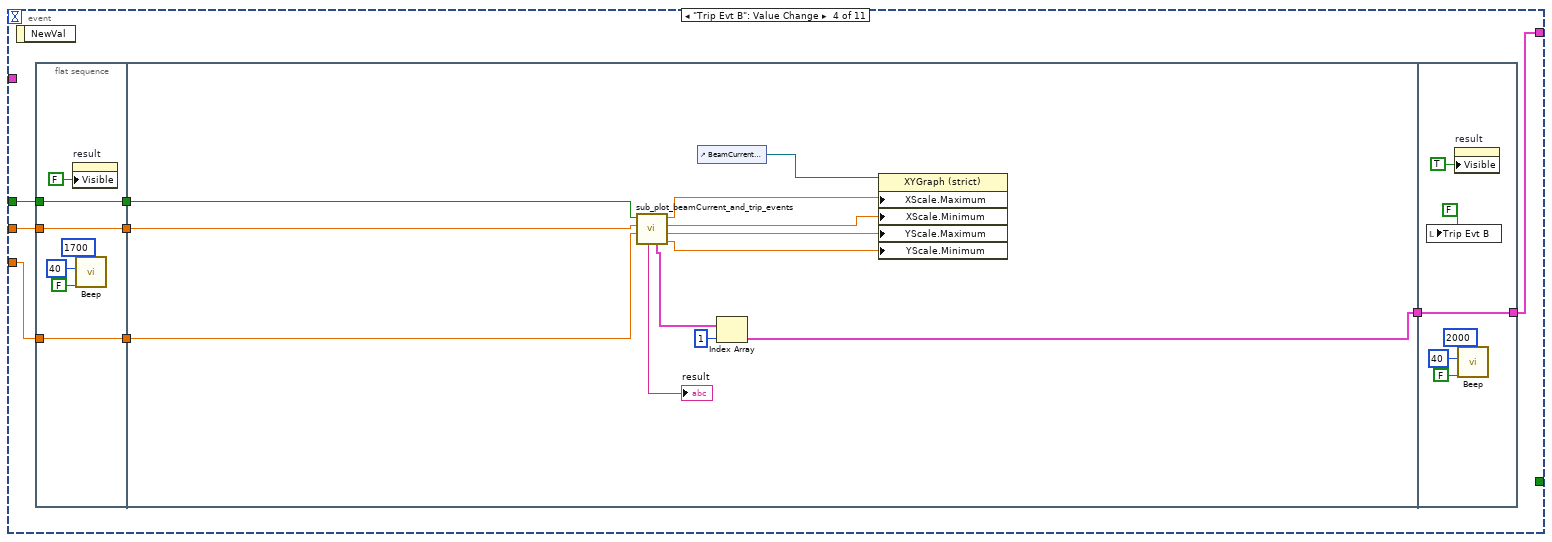
[diagram p19: hidden frame]
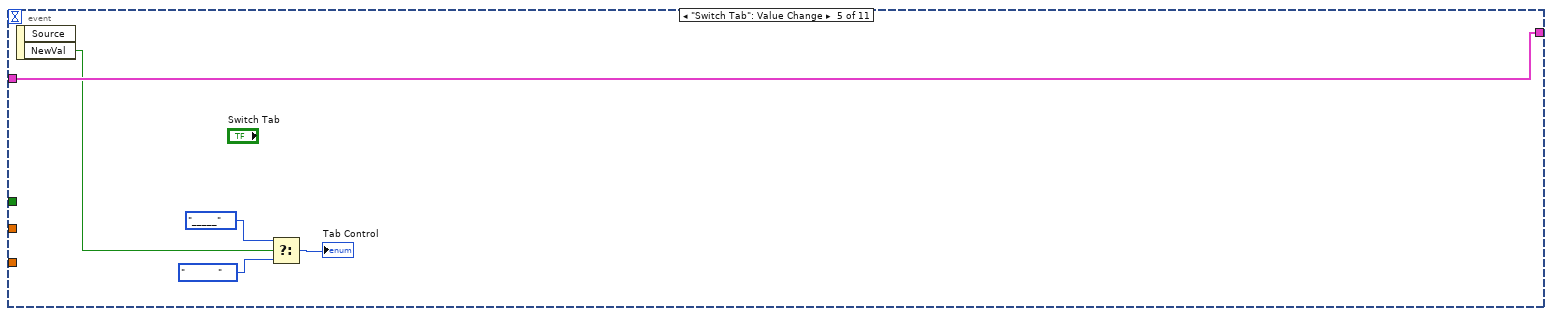
[diagram p20: hidden frame]
diagram:
  w16 = 0 ("index")
  w22 = string[] ["BR-PS-HC-101:setI", "BR-PS-HC-102:setI", "BR-PS-HC-103:setI", "BR-PS-HC-104:setI", "BR-PS-HC-105:setI", "BR-PS-HC-106:setI", "BR-PS-HC-107:setI", "BR-PS-HC-108:setI", "BR-PS-HC-109:setI", "BR-PS-HC-110:setI", "BR-PS-HC-201:setI", "BR-PS-HC-202:setI", "BR-PS-HC-203:setI", "BR-PS-HC-204:setI", "BR-PS-HC-205:setI", "BR-PS-HC-206:setI", "BR-PS-HC-207:setI", "BR-PS-HC-208:setI", "BR-PS-HC-209:setI", "BR-PS-HC-210:setI", "BR-PS-HC-301:setI", "BR-PS-HC-302:setI", "BR-PS-HC-303:setI", "BR-PS-HC-304:setI", "BR-PS-HC-305:setI", "BR-PS-HC-306:setI", "BR-PS-HC-307:setI", "BR-PS-HC-308:setI", "BR-PS-HC-309:setI", "BR-PS-HC-310:setI", "BR-PS-HC-401:setI", "BR-PS-HC-402:setI", "BR-PS-HC-403:setI", "BR-PS-HC-404:setI", "BR-PS-HC-405:setI", "BR-PS-HC-406:setI", "BR-PS-HC-407:setI", "BR-PS-HC-408:setI", "BR-PS-HC-409:setI", "BR-PS-HC-410:setI", "BR-PS-HC-501:setI", "BR-PS-HC-502:setI", "BR-PS-HC-503:setI", "BR-PS-HC-504:setI", "BR-PS-HC-505:setI", "BR-PS-HC-506:setI", "BR-PS-HC-507:setI", "BR-PS-HC-508:setI", "BR-PS-HC-509:setI", "BR-PS-HC-510:setI", "BR-PS-HC-601:setI", "BR-PS-HC-602:setI", "BR-PS-HC-603:setI", "BR-PS-HC-603a:setI", "BR-PS-HC-604:setI", "BR-PS-HC-605:setI", "BR-PS-HC-606:setI", "BR-PS-HC-606a:setI", "BR-PS-HC-607:setI", "BR-PS-HC-608:setI", "BR-PS-HC-609:setI", "BR-PS-HC-610:setI", "BR-PS-VC-101:setI", "BR-PS-VC-102:setI", "BR-PS-VC-103:setI", "BR-PS-VC-104:setI", "BR-PS-VC-105:setI", "BR-PS-VC-106:setI", "BR-PS-VC-201:setI", "BR-PS-VC-202:setI", "BR-PS-VC-203:setI", "BR-PS-VC-204:setI", "BR-PS-VC-205:setI", "BR-PS-VC-206:setI", "BR-PS-VC-301:setI", "BR-PS-VC-302:setI", "BR-PS-VC-303:setI", "BR-PS-VC-304:setI", "BR-PS-VC-305:setI", "BR-PS-VC-306:setI", "BR-PS-VC-401:setI", "BR-PS-VC-402:setI", "BR-PS-VC-403:setI", "BR-PS-VC-404:setI", "BR-PS-VC-405:setI", "BR-PS-VC-406:setI", "BR-PS-VC-501:setI", "BR-PS-VC-502:setI", "BR-PS-VC-503:setI", "BR-PS-VC-504:setI", "BR-PS-VC-505:setI", "BR-PS-VC-506:setI", "BR-PS-VC-601:setI", "BR-PS-VC-602:setI", "BR-PS-VC-602a:setI", "BR-PS-VC-603:setI", "BR-PS-VC-604:setI", "BR-PS-VC-604a:setI", "BR-PS-VC-605:setI", "BR-PS-VC-606:setI", "BR-PS-VC-100a:setI", "BR-PS-SD:setI", "BR-PS-SF:setI", "cpsc_027:AO:SLOW_SET:CH:1", "BR-RF-LLRF:setStationPhase", "TI-INJ-PROC:setTinj", "BR-PS-INJ-SE:setHV", "CPCIPM-TI-EVR:Pulse1DelaySet", "BR-PS-INJ-KI:setHV", "CPCIPM-TI-EVR:Pulse2DelaySet", "BR-PS-QF:setWfDC", "BR-PS-QM:setWfDC", "BR-PS-Q1:setWfDC", "BR-PS-Q2:setWfDC", "BR-PS-BEND:setWfDC"]  # PV nanes (BR_without_Wf, cpsc_037:AO:SLOW_SET:CH:3)
  w23 = string[] ["LI-ES-CPS-01:SETMODE", "LI-ES-CPS-01:PULSEMODE", "LI-ES-BPS-01:SETU:GRID", "LI-ES-BPS-01:SETU:SBM", "LI-ES-BPS-01:SETU:MBM", "LI-RF-CAB-07:SET:MODE", "LI-RF-HVP-11:SET:U", "LI-RF-CAB-09:SET:MODE", "LI-RF-HVP-21:SET:U", "LI-RF-HVP-31:SET:U", "LI-RF-WGA-01:SET:POS", "LI-RF-WGA-02:SET:POS", "LI-RF-WGA-03:SET:POS", "LI-RF-SFT-01:SET:POS", "LI-RF-SFT-02:SET:POS", "LI-RF-SFT-03:SET:POS", "LI-RF-CTR-01:ES:SET:DEG", "LI-RF-CTR-01:SP:SET:DEG", "LI-RF-CTR-01:K123:SET:DEG", "LI-RF-CTR-01:K1:SET:DEG", "LI-RF-CTR-01:K3:SET:DEG", "LI-RF-AMP-01:SET:PWR", "LI-RF-AMP-02:SET:PWR", "LI-MA-SPS-01:SET:I", "LI-MA-SPS-02:SET:I", "LI-MA-SPS-03:SET:I", "LI-MA-SPS-04:SET:I", "LI-MA-SPS-05:SET:I", "LI-MA-SPS-06:SET:I", "LI-MA-SPS-07:SET:I", "LI-MA-SPS-08:SET:I", "LI-MA-SPS-09:SET:I", "LI-MA-SPS-10:SET:I", "LI-MA-SPS-11:SET:I", "LI-MA-SPS-12:SET:I", "LI-MA-SPS-13:SET:I", "LI-MA-SPS-14:SET:I", "LI-MA-SPS-15:SET:I", "LI-MA-SPS-16:SET:I", "LI-MA-STP-01:SET:I", "LI-MA-STP-02:SET:I", "LI-MA-STP-03:SET:I", "LI-MA-STP-04:SET:I", "LI-MA-STP-05:SET:I", "LI-MA-STP-06:SET:I", "LI-MA-STP-07:SET:I", "LI-MA-STP-08:SET:I", "LI-MA-STP-09:SET:I", "LI-MA-STP-10:SET:I", "LI-MA-STP-11:SET:I", "LI-MA-STP-12:SET:I", "LI-MA-STP-13:SET:I", "LI-MA-STP-14:SET:I", "LI-MA-STP-15:SET:I", "LI-MA-STP-16:SET:I", "LI-MA-QPS-01:SET:I", "LI-MA-QPS-02:SET:I", "LI-MA-QPS-03:SET:I", "LI-MA-QPS-04:SET:I", "LI-MA-QPS-05:SET:I", "LI-MA-QPS-06:SET:I", "CPCITM-TI-EVRTG:Pulse7DelaySet", "CPCITM-TI-EVRTG:Pulse7WidthSet", "CPCITM-TI-EVRTG:GTX7DlySet", "CPCITM-TI-EVRTG:Pulse6DelaySet", "CPCITM-TI-EVRTG:Pulse6WidthSet", "CPCITM-TI-EVRTG:GTX6DlySet", "CPCILI-TI-EVR:Pulse2DelaySet", "CPCILI-TI-EVR:Pulse2WidthSet", "CPCILI-TI-EVR:Pulse3DelaySet", "CPCILI-TI-EVR:Pulse3WidthSet", "CPCILI-TI-EVR:Pulse4DelaySet", "CPCILI-TI-EVR:Pulse4WidthSet", "CPCILI-TI-EVR:Pulse5DelaySet", "CPCILI-TI-EVR:Pulse5WidthSet", "CPCILI-TI-EVR:Pulse6DelaySet", "CPCILI-TI-EVR:Pulse6WidthSet", "CPCILI-TI-EVR:Pulse7DelaySet", "CPCILI-TI-EVR:Pulse7WidthSet", "CPCILI-TI-EVR:Pulse8DelaySet", "CPCILI-TI-EVR:Pulse8WidthSet", "CPCILI-TI-EVR:Pulse9DelaySet", "CPCILI-TI-EVR:Pulse9WidthSet", "CPCITM-TI-EVRTG:GTX6DlySet", "CPCITM-TI-EVRTG:GTX7DlySet"]  # PV nanes(LINAC) without 3 set
  w24 = string[] ["TI-INJ-PROC:TopupHiLowStart", "TI-INJ-PROC:setBucketAddressStart", "TI-INJ-PROC:setBucketAddressLast", "TI-INJ-PROC:setBucketAddressStep", "TI-INJ-PROC:setPreCycle", "TI-INJ-PROC:setPostCycle", "TI-INJ-PROC:setBeamCurrentTopupHi", "TI-INJ-PROC:setBeamCurrentTopupLo", "TI-INJ-PROC:setSingleBunchAddr", "TI-INJ-PROC:setSingleInjCycle", "TI-INJ-PROC:setSingleBeamCurrent"]  # PV nanes(Others)
  w25 = string[] ["SR-ID-IU22-05:setECMode", "SR-ID-IU22A-09:setECMode", "SR-ID-IU22B-09:setECMode", "SR-ID-IUT22-21:setECMode", "SR-ID-IU22-23:setECMode", "SR-ID-IU22A-25:setECMode", "SR-ID-IU22B-25:setECMode", "SR-ID-EPU48A-41:setECMode", "SR-ID-EPU48B-41:setECMode", "SR-ID-EPU46-45:setECMode"]  # ID_mode
  (unwired) "cpsc_037:AO:SLOW_SET:CH:3" ("regular expression")
  w26 = string[] ["SR-DI-XPC-40:cam:AcquireTime", "SR-DI-XPC-40:cam:Gain"]  # Port40
  w27 = string[] ["LI:controlState0", "TI-INJ-PROC:trig-BRAC-ONOFF", "SR:controlState0"]  # Power Saving
  (unwired) "CPCITM-TI-EVRTG:GTX6CtrlGTXPHSet" ("regular expression")
  (unwired) "CPCITM-TI-EVRTG:GTX7CtrlGTXPHSet" ("regular expression")
  w30 = string[] ["SR-ID-IU22-05:gapMotorOff", "SR-ID-IU22A-09:gapMotorOff", "SR-ID-IU22B-09:gapMotorOff", "SR-ID-IUT22-21:gapMotorOff", "SR-ID-IU22-23:gapMotorOff", "SR-ID-IU22A-25:gapMotorOff", "SR-ID-IU22B-25:gapMotorOff", "SR-ID-EPU48A-41:gapMotorOff", "SR-ID-EPU48B-41:gapMotorOff", "SR-ID-EPU46-45:gapMotorOff", "SR-ID-EPU48A-41:phaseMotorOff", "SR-ID-EPU48B-41:phaseMotorOff", "SR-ID-EPU46-45:phaseMotorOff"]  # ID MO
  w29 = string[] ["SR-ID-IU22-05:setGap", "SR-ID-IU22A-09:setGap", "SR-ID-IU22B-09:setGap", "SR-ID-IUT22-21:setGap", "SR-ID-IU22-23:setGap", "SR-ID-IU22A-25:setGap", "SR-ID-IU22B-25:setGap", "SR-ID-EPU48A-41:setGap", "SR-ID-EPU48A-41:setPhase", "SR-ID-EPU48B-41:setGap", "SR-ID-EPU48B-41:setPhase", "SR-ID-EPU46-45:setGap", "SR-ID-EPU46-45:setPhase", "SR-ID-IUT22-21:getGapTaper", "SR-ID-EPU48PS-41:setGap", "SR-ID-IUT22-21:setGapMode"]  # PV nanes(ID gap_phase_Taper_)
  w38 = string[] ["SR-PS-BEND:setI", "SR-PS-HC-011:setI", "SR-PS-HC-012:setI", "SR-PS-HC-013:setI", "SR-PS-HC-014:setI", "SR-PS-HC-015:setI", "SR-PS-HC-016:setI", "SR-PS-HC-017:setI", "SR-PS-HC-021:setI", "SR-PS-HC-022:setI", "SR-PS-HC-023:setI", "SR-PS-HC-024:setI", "SR-PS-HC-025:setI", "SR-PS-HC-026:setI", "SR-PS-HC-027:setI", "SR-PS-HC-031:setI", "SR-PS-HC-032:setI", "SR-PS-HC-033:setI", "SR-PS-HC-034:setI", "SR-PS-HC-035:setI", "SR-PS-HC-036:setI", "SR-PS-HC-037:setI", "SR-PS-HC-041:setI", "SR-PS-HC-042:setI", "SR-PS-HC-043:setI", "SR-PS-HC-044:setI", "SR-PS-HC-045:setI", "SR-PS-HC-046:setI", "SR-PS-HC-047:setI", "SR-PS-HC-051:setI", "SR-PS-HC-052:setI", "SR-PS-HC-053:setI", "SR-PS-HC-054:setI", "SR-PS-HC-055:setI", "SR-PS-HC-056:setI", "SR-PS-HC-057:setI", "SR-PS-HC-061:setI", "SR-PS-HC-062:setI", "SR-PS-HC-063:setI", "SR-PS-HC-064:setI", "SR-PS-HC-065:setI", "SR-PS-HC-066:setI", "SR-PS-HC-067:setI", "SR-PS-HC-071:setI", "SR-PS-HC-072:setI", "SR-PS-HC-073:setI", "SR-PS-HC-074:setI", "SR-PS-HC-075:setI", "SR-PS-HC-076:setI", "SR-PS-HC-077:setI", "SR-PS-HC-081:setI", "SR-PS-HC-082:setI", "SR-PS-HC-083:setI", "SR-PS-HC-084:setI", "SR-PS-HC-085:setI", "SR-PS-HC-086:setI", "SR-PS-HC-087:setI", "SR-PS-HC-091:setI", "SR-PS-HC-092:setI", "SR-PS-HC-093:setI", "SR-PS-HC-094:setI", "SR-PS-HC-095:setI", "SR-PS-HC-096:setI", "SR-PS-HC-097:setI", "SR-PS-HC-101:setI", "SR-PS-HC-102:setI", "SR-PS-HC-103:setI", "SR-PS-HC-104:setI", "SR-PS-HC-105:setI", "SR-PS-HC-106:setI", "SR-PS-HC-107:setI", "SR-PS-HC-111:setI", "SR-PS-HC-112:setI", "SR-PS-HC-113:setI", "SR-PS-HC-114:setI", "SR-PS-HC-115:setI", "SR-PS-HC-116:setI", "SR-PS-HC-117:setI", "SR-PS-HC-121:setI", "SR-PS-HC-122:setI", "SR-PS-HC-123:setI", "SR-PS-HC-124:setI", "SR-PS-HC-125:setI", "SR-PS-HC-126:setI", "SR-PS-HC-127:setI", "SR-PS-HC-131:setI", "SR-PS-HC-132:setI", "SR-PS-HC-133:setI", "SR-PS-HC-134:setI", "SR-PS-HC-135:setI", "SR-PS-HC-136:setI", "SR-PS-HC-137:setI", "SR-PS-HC-141:setI", "SR-PS-HC-142:setI", "SR-PS-HC-143:setI", "SR-PS-HC-144:setI", "SR-PS-HC-145:setI", "SR-PS-HC-146:setI", "SR-PS-HC-147:setI", "SR-PS-HC-151:setI", "SR-PS-HC-152:setI", "SR-PS-HC-153:setI", "SR-PS-HC-154:setI", "SR-PS-HC-155:setI", "SR-PS-HC-156:setI", "SR-PS-HC-157:setI", "SR-PS-HC-161:setI", "SR-PS-HC-162:setI", "SR-PS-HC-163:setI", "SR-PS-HC-164:setI", "SR-PS-HC-165:setI", "SR-PS-HC-166:setI", "SR-PS-HC-167:setI", "SR-PS-HC-171:setI", "SR-PS-HC-172:setI", "SR-PS-HC-173:setI", "SR-PS-HC-174:setI", "SR-PS-HC-175:setI", "SR-PS-HC-176:setI", "SR-PS-HC-177:setI", "SR-PS-HC-181:setI", "SR-PS-HC-182:setI", "SR-PS-HC-183:setI", "SR-PS-HC-184:setI", "SR-PS-HC-185:setI", "SR-PS-HC-186:setI", "SR-PS-HC-187:setI", "SR-PS-HC-191:setI", "SR-PS-HC-192:setI", "SR-PS-HC-193:setI", "SR-PS-HC-194:setI", "SR-PS-HC-195:setI", "SR-PS-HC-196:setI", "SR-PS-HC-197:setI", "SR-PS-HC-201:setI", "SR-PS-HC-202:setI", "SR-PS-HC-203:setI", "SR-PS-HC-204:setI", "SR-PS-HC-205:setI", "SR-PS-HC-206:setI", "SR-PS-HC-207:setI", "SR-PS-HC-211:setI", "SR-PS-HC-212:setI", "SR-PS-HC-213:setI", "SR-PS-HC-214:setI", "SR-PS-HC-215:setI", "SR-PS-HC-216:setI", "SR-PS-HC-217:setI", "SR-PS-HC-221:setI", "SR-PS-HC-222:setI", "SR-PS-HC-223:setI", "SR-PS-HC-224:setI", "SR-PS-HC-225:setI", "SR-PS-HC-226:setI", "SR-PS-HC-227:setI", "SR-PS-HC-231:setI", "SR-PS-HC-232:setI", "SR-PS-HC-233:setI", "SR-PS-HC-234:setI", "SR-PS-HC-235:setI", "SR-PS-HC-236:setI", "SR-PS-HC-237:setI", "SR-PS-HC-241:setI", "SR-PS-HC-242:setI", "SR-PS-HC-243:setI", "SR-PS-HC-244:setI", "SR-PS-HC-245:setI", "SR-PS-HC-246:setI", "SR-PS-HC-247:setI", "SR-PS-VC-011:setI", "SR-PS-VC-012:setI", "SR-PS-VC-013:setI", "SR-PS-VC-014:setI", "SR-PS-VC-015:setI", "SR-PS-VC-016:setI", "SR-PS-VC-017:setI", "SR-PS-VC-021:setI", "SR-PS-VC-022:setI", "SR-PS-VC-023:setI", "SR-PS-VC-024:setI", "SR-PS-VC-025:setI", "SR-PS-VC-026:setI", "SR-PS-VC-027:setI", "SR-PS-VC-031:setI", "SR-PS-VC-032:setI", "SR-PS-VC-033:setI", "SR-PS-VC-034:setI", "SR-PS-VC-035:setI", "SR-PS-VC-036:setI", "SR-PS-VC-037:setI", "SR-PS-VC-041:setI", "SR-PS-VC-042:setI", "SR-PS-VC-043:setI", "SR-PS-VC-044:setI", "SR-PS-VC-045:setI", "SR-PS-VC-046:setI", "SR-PS-VC-047:setI", "SR-PS-VC-051:setI", "SR-PS-VC-052:setI", "SR-PS-VC-053:setI", "SR-PS-VC-054:setI", "SR-PS-VC-055:setI", "SR-PS-VC-056:setI", "SR-PS-VC-057:setI", "SR-PS-VC-061:setI", "SR-PS-VC-062:setI", "SR-PS-VC-063:setI", "SR-PS-VC-064:setI", "SR-PS-VC-065:setI", "SR-PS-VC-066:setI", "SR-PS-VC-067:setI", "SR-PS-VC-071:setI", "SR-PS-VC-072:setI", "SR-PS-VC-073:setI", "SR-PS-VC-074:setI", "SR-PS-VC-075:setI", "SR-PS-VC-076:setI", "SR-PS-VC-077:setI", "SR-PS-VC-081:setI", "SR-PS-VC-082:setI", "SR-PS-VC-083:setI", "SR-PS-VC-084:setI", "SR-PS-VC-085:setI", "SR-PS-VC-086:setI", "SR-PS-VC-087:setI", "SR-PS-VC-091:setI", "SR-PS-VC-092:setI", "SR-PS-VC-093:setI", "SR-PS-VC-094:setI", "SR-PS-VC-095:setI", "SR-PS-VC-096:setI", "SR-PS-VC-097:setI", "SR-PS-VC-101:setI", "SR-PS-VC-102:setI", "SR-PS-VC-103:setI", "SR-PS-VC-104:setI", "SR-PS-VC-105:setI", "SR-PS-VC-106:setI", "SR-PS-VC-107:setI", "SR-PS-VC-111:setI", "SR-PS-VC-112:setI", "SR-PS-VC-113:setI", "SR-PS-VC-114:setI", "SR-PS-VC-115:setI", "SR-PS-VC-116:setI", "SR-PS-VC-117:setI", "SR-PS-VC-121:setI", "SR-PS-VC-122:setI", "SR-PS-VC-123:setI", "SR-PS-VC-124:setI", "SR-PS-VC-125:setI", "SR-PS-VC-126:setI", "SR-PS-VC-127:setI", "SR-PS-VC-131:setI", "SR-PS-VC-132:setI", "SR-PS-VC-133:setI", "SR-PS-VC-134:setI", "SR-PS-VC-135:setI", "SR-PS-VC-136:setI", "SR-PS-VC-137:setI", "SR-PS-VC-141:setI", "SR-PS-VC-142:setI", "SR-PS-VC-143:setI", "SR-PS-VC-144:setI", "SR-PS-VC-145:setI", "SR-PS-VC-146:setI", "SR-PS-VC-147:setI", "SR-PS-VC-151:setI", "SR-PS-VC-152:setI", "SR-PS-VC-153:setI", "SR-PS-VC-154:setI", "SR-PS-VC-155:setI", "SR-PS-VC-156:setI", "SR-PS-VC-157:setI", "SR-PS-VC-161:setI", "SR-PS-VC-162:setI", "SR-PS-VC-163:setI", "SR-PS-VC-164:setI", "SR-PS-VC-165:setI", "SR-PS-VC-166:setI", "SR-PS-VC-167:setI", "SR-PS-VC-171:setI", "SR-PS-VC-172:setI", "SR-PS-VC-173:setI", "SR-PS-VC-174:setI", "SR-PS-VC-175:setI", "SR-PS-VC-176:setI", "SR-PS-VC-177:setI", "SR-PS-VC-181:setI", "SR-PS-VC-182:setI", "SR-PS-VC-183:setI", "SR-PS-VC-184:setI", "SR-PS-VC-185:setI", "SR-PS-VC-186:setI", "SR-PS-VC-187:setI", "SR-PS-VC-191:setI", "SR-PS-VC-192:setI", "SR-PS-VC-193:setI", "SR-PS-VC-194:setI", "SR-PS-VC-195:setI", "SR-PS-VC-196:setI", "SR-PS-VC-197:setI", "SR-PS-VC-201:setI", "SR-PS-VC-202:setI", "SR-PS-VC-203:setI", "SR-PS-VC-204:setI", "SR-PS-VC-205:setI", "SR-PS-VC-206:setI", "SR-PS-VC-207:setI", "SR-PS-VC-211:setI", "SR-PS-VC-212:setI", "SR-PS-VC-213:setI", "SR-PS-VC-214:setI", "SR-PS-VC-215:setI", "SR-PS-VC-216:setI", "SR-PS-VC-217:setI", "SR-PS-VC-221:setI", "SR-PS-VC-222:setI", "SR-PS-VC-223:setI", "SR-PS-VC-224:setI", "SR-PS-VC-225:setI", "SR-PS-VC-226:setI", "SR-PS-VC-227:setI", "SR-PS-VC-231:setI", "SR-PS-VC-232:setI", "SR-PS-VC-233:setI", "SR-PS-VC-234:setI", "SR-PS-VC-235:setI", "SR-PS-VC-236:setI", "SR-PS-VC-237:setI", "SR-PS-VC-241:setI", "SR-PS-VC-242:setI", "SR-PS-VC-243:setI", "SR-PS-VC-244:setI", "SR-PS-VC-245:setI", "SR-PS-VC-246:setI", "SR-PS-VC-247:setI", "SR-PS-QL1-0101:setI", "SR-PS-QL2-0102:setI", "SR-PS-QL3-0103:setI", "SR-PS-QS4-0104:setI", "SR-PS-QS5-0105:setI", "SR-PS-QS5-0106:setI", "SR-PS-QS4-0107:setI", "SR-PS-QS3-0108:setI", "SR-PS-QS2-0109:setI", "SR-PS-QS1-0110:setI", "SR-PS-QS1-0201:setI", "SR-PS-QS2-0202:setI", "SR-PS-QS3-0203:setI", "SR-PS-QS4-0204:setI", "SR-PS-QS5-0205:setI", "SR-PS-QS5-0206:setI", "SR-PS-QS4-0207:setI", "SR-PS-QS3-0208:setI", "SR-PS-QS2-0209:setI", "SR-PS-QS1-0210:setI", "SR-PS-QS1-0301:setI", "SR-PS-QS2-0302:setI", "SR-PS-QS3-0303:setI", "SR-PS-QS4-0304:setI", "SR-PS-QS5-0305:setI", "SR-PS-QS5-0306:setI", "SR-PS-QS4-0307:setI", "SR-PS-QS3-0308:setI", "SR-PS-QS2-0309:setI", "SR-PS-QS1-0310:setI", "SR-PS-QS1-0401:setI", "SR-PS-QS2-0402:setI", "SR-PS-QS3-0403:setI", "SR-PS-QS4-0404:setI", "SR-PS-QS5-0405:setI", "SR-PS-QS5-0406:setI", "SR-PS-QS4-0407:setI", "SR-PS-QL3-0408:setI", "SR-PS-QL2-0409:setI", "SR-PS-QL1-0410:setI", "SR-PS-QL1-0501:setI", "SR-PS-QL2-0502:setI", "SR-PS-QL3-0503:setI", "SR-PS-QS4-0504:setI", "SR-PS-QS5-0505:setI", "SR-PS-QS5-0506:setI", "SR-PS-QS4-0507:setI", "SR-PS-QS3-0508:setI", "SR-PS-QS2-0509:setI", "SR-PS-QS1-0510:setI", "SR-PS-QS1-0601:setI", "SR-PS-QS2-0602:setI", "SR-PS-QS3-0603:setI", "SR-PS-QS4-0604:setI", "SR-PS-QS5-0605:setI", "SR-PS-QS5-0606:setI", "SR-PS-QS4-0607:setI", "SR-PS-QS3-0608:setI", "SR-PS-QS2-0609:setI", "SR-PS-QS1-0610:setI", "SR-PS-QS1-0701:setI", "SR-PS-QS2-0702:setI", "SR-PS-QS3-0703:setI", "SR-PS-QS4-0704:setI", "SR-PS-QS5-0705:setI", "SR-PS-QS5-0706:setI", "SR-PS-QS4-0707:setI", "SR-PS-QS3-0708:setI", "SR-PS-QS2-0709:setI", "SR-PS-QS1-0710:setI", "SR-PS-QS1-0801:setI", "SR-PS-QS2-0802:setI", "SR-PS-QS3-0803:setI", "SR-PS-QS4-0804:setI", "SR-PS-QS5-0805:setI", "SR-PS-QS5-0806:setI", "SR-PS-QS4-0807:setI", "SR-PS-QL3-0808:setI", "SR-PS-QL2-0809:setI", "SR-PS-QL1-0810:setI", "SR-PS-QL1-0901:setI", "SR-PS-QL2-0902:setI", "SR-PS-QL3-0903:setI", "SR-PS-QS4-0904:setI", "SR-PS-QS5-0905:setI", "SR-PS-QS5-0906:setI", "SR-PS-QS4-0907:setI", "SR-PS-QS3-0908:setI", "SR-PS-QS2-0909:setI", "SR-PS-QS1-0910:setI", "SR-PS-QS1-1001:setI", "SR-PS-QS2-1002:setI", "SR-PS-QS3-1003:setI", "SR-PS-QS4-1004:setI", "SR-PS-QS5-1005:setI", "SR-PS-QS5-1006:setI", "SR-PS-QS4-1007:setI", "SR-PS-QS3-1008:setI", "SR-PS-QS2-1009:setI", "SR-PS-QS1-1010:setI", "SR-PS-QS1-1101:setI", "SR-PS-QS2-1102:setI", "SR-PS-QS3-1103:setI", "SR-PS-QS4-1104:setI", "SR-PS-QS5-1105:setI", "SR-PS-QS5-1106:setI", "SR-PS-QS4-1107:setI", "SR-PS-QS3-1108:setI", "SR-PS-QS2-1109:setI", "SR-PS-QS1-1110:setI", "SR-PS-QS1-1201:setI", "SR-PS-QS2-1202:setI", "SR-PS-QS3-1203:setI", "SR-PS-QS4-1204:setI", "SR-PS-QS5-1205:setI", "SR-PS-QS5-1206:setI", "SR-PS-QS4-1207:setI", "SR-PS-QL3-1208:setI", "SR-PS-QL2-1209:setI", "SR-PS-QL1-1210:setI", "SR-PS-QL1-1301:setI", "SR-PS-QL2-1302:setI", "SR-PS-QL3-1303:setI", "SR-PS-QS4-1304:setI", "SR-PS-QS5-1305:setI", "SR-PS-QS5-1306:setI", "SR-PS-QS4-1307:setI", "SR-PS-QS3-1308:setI", "SR-PS-QS2-1309:setI", "SR-PS-QS1-1310:setI", "SR-PS-QS1-1401:setI", "SR-PS-QS2-1402:setI", "SR-PS-QS3-1403:setI", "SR-PS-QS4-1404:setI", "SR-PS-QS5-1405:setI", "SR-PS-QS5-1406:setI", "SR-PS-QS4-1407:setI", "SR-PS-QS3-1408:setI", "SR-PS-QS2-1409:setI", "SR-PS-QS1-1410:setI", "SR-PS-QS1-1501:setI", "SR-PS-QS2-1502:setI", "SR-PS-QS3-1503:setI", "SR-PS-QS4-1504:setI", "SR-PS-QS5-1505:setI", "SR-PS-QS5-1506:setI", "SR-PS-QS4-1507:setI", "SR-PS-QS3-1508:setI", "SR-PS-QS2-1509:setI", "SR-PS-QS1-1510:setI", "SR-PS-QS1-1601:setI", "SR-PS-QS2-1602:setI", "SR-PS-QS3-1603:setI", "SR-PS-QS4-1604:setI", "SR-PS-QS5-1605:setI", "SR-PS-QS5-1606:setI", "SR-PS-QS4-1607:setI", "SR-PS-QL3-1608:setI", "SR-PS-QL2-1609:setI", "SR-PS-QL1-1610:setI", "SR-PS-QL1-1701:setI", "SR-PS-QL2-1702:setI", "SR-PS-QL3-1703:setI", "SR-PS-QS4-1704:setI", "SR-PS-QS5-1705:setI", "SR-PS-QS5-1706:setI", "SR-PS-QS4-1707:setI", "SR-PS-QS3-1708:setI", "SR-PS-QS2-1709:setI", "SR-PS-QS1-1710:setI", "SR-PS-QS1-1801:setI", "SR-PS-QS2-1802:setI", "SR-PS-QS3-1803:setI", "SR-PS-QS4-1804:setI", "SR-PS-QS5-1805:setI", "SR-PS-QS5-1806:setI", "SR-PS-QS4-1807:setI", "SR-PS-QS3-1808:setI", "SR-PS-QS2-1809:setI", "SR-PS-QS1-1810:setI", "SR-PS-QS1-1901:setI", "SR-PS-QS2-1902:setI", "SR-PS-QS3-1903:setI", "SR-PS-QS4-1904:setI", "SR-PS-QS5-1905:setI", "SR-PS-QS5-1906:setI", "SR-PS-QS4-1907:setI", "SR-PS-QS3-1908:setI", "SR-PS-QS2-1909:setI", "SR-PS-QS1-1910:setI", "SR-PS-QS1-2001:setI", "SR-PS-QS2-2002:setI", "SR-PS-QS3-2003:setI", "SR-PS-QS4-2004:setI", "SR-PS-QS5-2005:setI", "SR-PS-QS5-2006:setI", "SR-PS-QS4-2007:setI", "SR-PS-QL3-2008:setI", "SR-PS-QL2-2009:setI", "SR-PS-QL1-2010:setI", "SR-PS-QL1-2101:setI", "SR-PS-QL2-2102:setI", "SR-PS-QL3-2103:setI", "SR-PS-QS4-2104:setI", "SR-PS-QS5-2105:setI", "SR-PS-QS5-2106:setI", "SR-PS-QS4-2107:setI", "SR-PS-QS3-2108:setI", "SR-PS-QS2-2109:setI", "SR-PS-QS1-2110:setI", "SR-PS-QS1-2201:setI", "SR-PS-QS2-2202:setI", "SR-PS-QS3-2203:setI", "SR-PS-QS4-2204:setI", "SR-PS-QS5-2205:setI", "SR-PS-QS5-2206:setI", "SR-PS-QS4-2207:setI", "SR-PS-QS3-2208:setI", "SR-PS-QS2-2209:setI", "SR-PS-QS1-2210:setI", "SR-PS-QS1-2301:setI", "SR-PS-QS2-2302:setI", "SR-PS-QS3-2303:setI", "SR-PS-QS4-2304:setI", "SR-PS-QS5-2305:setI", "SR-PS-QS5-2306:setI", "SR-PS-QS4-2307:setI", "SR-PS-QS3-2308:setI", "SR-PS-QS2-2309:setI", "SR-PS-QS1-2310:setI", "SR-PS-QS1-2401:setI", "SR-PS-QS2-2402:setI", "SR-PS-QS3-2403:setI", "SR-PS-QS4-2404:setI", "SR-PS-QS5-2405:setI", "SR-PS-QS5-2406:setI", "SR-PS-QS4-2407:setI", "SR-PS-QL3-2408:setI", "SR-PS-QL2-2409:setI", "SR-PS-QL1-2410:setI", "SR-PS-S1-011:setI", "SR-PS-S2-012:setI", "SR-PS-SD-013:setI", "SR-PS-SF-014:setI", "SR-PS-SD-015:setI", "SR-PS-S4-016:setI", "SR-PS-S3-017:setI", "SR-PS-S5-021:setI", "SR-PS-S6-022:setI", "SR-PS-SD-023:setI", "SR-PS-SF-024:setI", "SR-PS-SD-025:setI", "SR-PS-S6-026:setI", "SR-PS-S5-027:setI", "SR-PS-S5-031:setI", "SR-PS-S6-032:setI", "SR-PS-SD-033:setI", "SR-PS-SF-034:setI", "SR-PS-SD-035:setI", "SR-PS-S6-036:setI", "SR-PS-S5-037:setI", "SR-PS-S3-041:setI", "SR-PS-S4-042:setI", "SR-PS-SD-043:setI", "SR-PS-SF-044:setI", "SR-PS-SD-045:setI", "SR-PS-S2-046:setI", "SR-PS-S1-047:setI", "SR-PS-S1-051:setI", "SR-PS-S2-052:setI", "SR-PS-SD-053:setI", "SR-PS-SF-054:setI", "SR-PS-SD-055:setI", "SR-PS-S4-056:setI", "SR-PS-S3-057:setI", "SR-PS-S5-061:setI", "SR-PS-S6-062:setI", "SR-PS-SD-063:setI", "SR-PS-SF-064:setI", "SR-PS-SD-065:setI", "SR-PS-S6-066:setI", "SR-PS-S5-067:setI", "SR-PS-S5-071:setI", "SR-PS-S6-072:setI", "SR-PS-SD-073:setI", "SR-PS-SF-074:setI", "SR-PS-SD-075:setI", "SR-PS-S6-076:setI", "SR-PS-S5-077:setI", "SR-PS-S3-081:setI", "SR-PS-S4-082:setI", "SR-PS-SD-083:setI", "SR-PS-SF-084:setI", "SR-PS-SD-085:setI", "SR-PS-S2-086:setI", "SR-PS-S1-087:setI", "SR-PS-S1-091:setI", "SR-PS-S2-092:setI", "SR-PS-SD-093:setI", "SR-PS-SF-094:setI", "SR-PS-SD-095:setI", "SR-PS-S4-096:setI", "SR-PS-S3-097:setI", "SR-PS-S5-101:setI", "SR-PS-S6-102:setI", "SR-PS-SD-103:setI", "SR-PS-SF-104:setI", "SR-PS-SD-105:setI", "SR-PS-S6-106:setI", "SR-PS-S5-107:setI", "SR-PS-S5-111:setI", "SR-PS-S6-112:setI", "SR-PS-SD-113:setI", "SR-PS-SF-114:setI", "SR-PS-SD-115:setI", "SR-PS-S6-116:setI", "SR-PS-S5-117:setI", "SR-PS-S3-121:setI", "SR-PS-S4-122:setI", "SR-PS-SD-123:setI", "SR-PS-SF-124:setI", "SR-PS-SD-125:setI", "SR-PS-S2-126:setI", "SR-PS-S1-127:setI", "SR-PS-S1-131:setI", "SR-PS-S2-132:setI", "SR-PS-SD-133:setI", "SR-PS-SF-134:setI", "SR-PS-SD-135:setI", "SR-PS-S4-136:setI", "SR-PS-S3-137:setI", "SR-PS-S5-141:setI", "SR-PS-S6-142:setI", "SR-PS-SD-143:setI", "SR-PS-SF-144:setI", "SR-PS-SD-145:setI", "SR-PS-S6-146:setI", "SR-PS-S5-147:setI", "SR-PS-S5-151:setI", "SR-PS-S6-152:setI", "SR-PS-SD-153:setI", "SR-PS-SF-154:setI", "SR-PS-SD-155:setI", "SR-PS-S6-156:setI", "SR-PS-S5-157:setI", "SR-PS-S3-161:setI", "SR-PS-S4-162:setI", "SR-PS-SD-163:setI", "SR-PS-SF-164:setI", "SR-PS-SD-165:setI", "SR-PS-S2-166:setI", "SR-PS-S1-167:setI", "SR-PS-S1-171:setI", "SR-PS-S2-172:setI", "SR-PS-SD-173:setI", "SR-PS-SF-174:setI", "SR-PS-SD-175:setI", "SR-PS-S4-176:setI", "SR-PS-S3-177:setI", "SR-PS-S5-181:setI", "SR-PS-S6-182:setI", "SR-PS-SD-183:setI", "SR-PS-SF-184:setI", "SR-PS-SD-185:setI", "SR-PS-S6-186:setI", "SR-PS-S5-187:setI", "SR-PS-S5-191:setI", "SR-PS-S6-192:setI", "SR-PS-SD-193:setI", "SR-PS-SF-194:setI", "SR-PS-SD-195:setI", "SR-PS-S6-196:setI", "SR-PS-S5-197:setI", "SR-PS-S3-201:setI", "SR-PS-S4-202:setI", "SR-PS-SD-203:setI", "SR-PS-SF-204:setI", "SR-PS-SD-205:setI", "SR-PS-S2-206:setI", "SR-PS-S1-207:setI", "SR-PS-S1-211:setI", "SR-PS-S2-212:setI", "SR-PS-SD-213:setI", "SR-PS-SF-214:setI", "SR-PS-SD-215:setI", "SR-PS-S4-216:setI", "SR-PS-S3-217:setI", "SR-PS-S5-221:setI", "SR-PS-S6-222:setI", "SR-PS-SD-223:setI", "SR-PS-SF-224:setI", "SR-PS-SD-225:setI", "SR-PS-S6-226:setI", "SR-PS-S5-227:setI", "SR-PS-S5-231:setI", "SR-PS-S6-232:setI", "SR-PS-SD-233:setI", "SR-PS-SF-234:setI", "SR-PS-SD-235:setI", "SR-PS-S6-236:setI", "SR-PS-S5-237:setI", "SR-PS-S3-241:setI", "SR-PS-S4-242:setI", "SR-PS-SD-243:setI", "SR-PS-SF-244:setI", "SR-PS-SD-245:setI", "SR-PS-S2-246:setI", "SR-PS-S1-247:setI", "SR-PS-SKEW-011:setI", "SR-PS-SKEW-012:setI", "SR-PS-SKEW-013:setI", "SR-PS-SKEW-014:setI", "SR-PS-SKEW-015:setI", "SR-PS-SKEW-016:setI", "SR-PS-SKEW-017:setI", "SR-PS-SKEW-021:setI", "SR-PS-SKEW-022:setI", "SR-PS-SKEW-023:setI", "SR-PS-SKEW-024:setI", "SR-PS-SKEW-025:setI", "SR-PS-SKEW-026:setI", "SR-PS-SKEW-027:setI", "SR-PS-SKEW-031:setI", "SR-PS-SKEW-032:setI", "SR-PS-SKEW-033:setI", "SR-PS-SKEW-034:setI", "SR-PS-SKEW-035:setI", "SR-PS-SKEW-036:setI", "SR-PS-SKEW-037:setI", "SR-PS-SKEW-041:setI", "SR-PS-SKEW-042:setI", "SR-PS-SKEW-043:setI", "SR-PS-SKEW-044:setI", "SR-PS-SKEW-045:setI", "SR-PS-SKEW-046:setI", "SR-PS-SKEW-047:setI", "SR-PS-SKEW-051:setI", "SR-PS-SKEW-052:setI", "SR-PS-SKEW-053:setI", "SR-PS-SKEW-054:setI", "SR-PS-SKEW-055:setI", "SR-PS-SKEW-056:setI", "SR-PS-SKEW-057:setI", "SR-PS-SKEW-061:setI", "SR-PS-SKEW-062:setI", "SR-PS-SKEW-063:setI", "SR-PS-SKEW-064:setI", "SR-PS-SKEW-065:setI", "SR-PS-SKEW-066:setI", "SR-PS-SKEW-067:setI", "SR-PS-SKEW-071:setI", "SR-PS-SKEW-072:setI", "SR-PS-SKEW-073:setI", "SR-PS-SKEW-074:setI", "SR-PS-SKEW-075:setI", "SR-PS-SKEW-076:setI", "SR-PS-SKEW-077:setI", "SR-PS-SKEW-081:setI", "SR-PS-SKEW-082:setI", "SR-PS-SKEW-083:setI", "SR-PS-SKEW-084:setI", "SR-PS-SKEW-085:setI", "SR-PS-SKEW-086:setI", "SR-PS-SKEW-087:setI", "SR-PS-SKEW-091:setI", "SR-PS-SKEW-092:setI", "SR-PS-SKEW-093:setI", "SR-PS-SKEW-094:setI", "SR-PS-SKEW-095:setI", "SR-PS-SKEW-096:setI", "SR-PS-SKEW-097:setI", "SR-PS-SKEW-101:setI", "SR-PS-SKEW-102:setI", "SR-PS-SKEW-103:setI", "SR-PS-SKEW-104:setI", "SR-PS-SKEW-105:setI", "SR-PS-SKEW-106:setI", "SR-PS-SKEW-107:setI", "SR-PS-SKEW-111:setI", "SR-PS-SKEW-112:setI", "SR-PS-SKEW-113:setI", "SR-PS-SKEW-114:setI", "SR-PS-SKEW-115:setI", "SR-PS-SKEW-116:setI", "SR-PS-SKEW-117:setI", "SR-PS-SKEW-121:setI", "SR-PS-SKEW-122:setI", "SR-PS-SKEW-123:setI", "SR-PS-SKEW-124:setI", "SR-PS-SKEW-125:setI", "SR-PS-SKEW-126:setI", "SR-PS-SKEW-127:setI", "SR-PS-SKEW-131:setI", "SR-PS-SKEW-132:setI", "SR-PS-SKEW-133:setI", "SR-PS-SKEW-134:setI", "SR-PS-SKEW-135:setI", "SR-PS-SKEW-136:setI", "SR-PS-SKEW-137:setI", "SR-PS-SKEW-141:setI", "SR-PS-SKEW-142:setI", "SR-PS-SKEW-143:setI", "SR-PS-SKEW-144:setI", "SR-PS-SKEW-145:setI", "SR-PS-SKEW-146:setI", "SR-PS-SKEW-147:setI", "SR-PS-SKEW-151:setI", "SR-PS-SKEW-152:setI", "SR-PS-SKEW-153:setI", "SR-PS-SKEW-154:setI", "SR-PS-SKEW-155:setI", "SR-PS-SKEW-156:setI", "SR-PS-SKEW-157:setI", "SR-PS-SKEW-161:setI", "SR-PS-SKEW-162:setI", "SR-PS-SKEW-163:setI", "SR-PS-SKEW-164:setI", "SR-PS-SKEW-165:setI", "SR-PS-SKEW-166:setI", "SR-PS-SKEW-167:setI", "SR-PS-SKEW-171:setI", "SR-PS-SKEW-172:setI", "SR-PS-SKEW-173:setI", "SR-PS-SKEW-174:setI", "SR-PS-SKEW-175:setI", "SR-PS-SKEW-176:setI", "SR-PS-SKEW-177:setI", "SR-PS-SKEW-181:setI", "SR-PS-SKEW-182:setI", "SR-PS-SKEW-183:setI", "SR-PS-SKEW-184:setI", "SR-PS-SKEW-185:setI", "SR-PS-SKEW-186:setI", "SR-PS-SKEW-187:setI", "SR-PS-SKEW-191:setI", "SR-PS-SKEW-192:setI", "SR-PS-SKEW-193:setI", "SR-PS-SKEW-194:setI", "SR-PS-SKEW-195:setI", "SR-PS-SKEW-196:setI", "SR-PS-SKEW-197:setI", "SR-PS-SKEW-201:setI", "SR-PS-SKEW-202:setI", "SR-PS-SKEW-203:setI", "SR-PS-SKEW-204:setI", "SR-PS-SKEW-205:setI", "SR-PS-SKEW-206:setI", "SR-PS-SKEW-207:setI", "SR-PS-SKEW-211:setI", "SR-PS-SKEW-212:setI", "SR-PS-SKEW-213:setI", "SR-PS-SKEW-214:setI", "SR-PS-SKEW-215:setI", "SR-PS-SKEW-216:setI", "SR-PS-SKEW-217:setI", "SR-PS-SKEW-221:setI", "SR-PS-SKEW-222:setI", "SR-PS-SKEW-223:setI", "SR-PS-SKEW-224:setI", "SR-PS-SKEW-225:setI", "SR-PS-SKEW-226:setI", "SR-PS-SKEW-227:setI", "SR-PS-SKEW-231:setI", "SR-PS-SKEW-232:setI", "SR-PS-SKEW-233:setI", "SR-PS-SKEW-234:setI", "SR-PS-SKEW-235:setI", "SR-PS-SKEW-236:setI", "SR-PS-SKEW-237:setI", "SR-PS-SKEW-241:setI", "SR-PS-SKEW-242:setI", "SR-PS-SKEW-243:setI", "SR-PS-SKEW-244:setI", "SR-PS-SKEW-245:setI", "SR-PS-SKEW-246:setI", "SR-PS-SKEW-247:setI", "SR-RF2-LLRF:setGapVoltage", "SR-RF2-LLRF:setStationPhase", "SR-RF3-LLRF:setGapVoltage", "SR-RF3-LLRF:setStationPhase", "SR-PS-DMB09-Q1:setI", "SR-PS-DMB09-Q2:setI", "SR-PS-DMB09-Q3:setI", "SR-PS-DMB25-Q1:setI", "SR-PS-DMB25-Q2:setI", "SR-PS-DMB25-Q3:setI", "SR-PS-DMB41-Q1:setI", "SR-PS-DMB41-Q2:setI", "SR-PS-DMB41-Q3:setI", "SR-PS-DMB09-HC1:setI", "SR-PS-DMB09-HC2:setI", "SR-PS-DMB09-VC1:setI", "SR-PS-DMB09-VC2:setI", "SR-PS-DMB25-HC1:setI", "SR-PS-DMB25-HC2:setI", "SR-PS-DMB25-VC1:setI", "SR-PS-DMB25-VC2:setI", "SR-PS-DMB41-HC1:setI", "SR-PS-DMB41-HC2:setI", "SR-PS-DMB41-VC1:setI", "SR-PS-DMB41-VC2:setI"]  # PV nanes(SR)
  w36 = string[] ["LTB-PS-HC-1:setI", "LTB-PS-HC-2:setI", "LTB-PS-HC-3:setI", "LTB-PS-HC-4:setI", "LTB-PS-HC-5:setI", "LTB-PS-VC-1:setI", "LTB-PS-VC-2:setI", "LTB-PS-VC-3:setI", "LTB-PS-VC-4:setI", "LTB-PS-VC-5:setI", "LTB-PS-VC-6:setI", "LTB-PS-VC-7:setI", "LTB-PS-Q1A:setI", "LTB-PS-Q1B:setI", "LTB-PS-Q1C:setI", "LTB-PS-Q2A:setI", "LTB-PS-Q2B:setI", "LTB-PS-Q2C:setI", "LTB-PS-Q3A:setI", "LTB-PS-Q3B:setI", "LTB-PS-Q4A:setI", "LTB-PS-Q4B:setI", "LTB-PS-QQ:setI", "LTB-PS-BEND-1:setI", "LTB-PS-VC-2a:setI", "LTB-PS-HC-3a:setI", "LTB-PS-HC-3b:setI", "LTB-PS-HC-4a:setI", "LTB-PS-HC-5a:setI", "LI-DI-SLIT-motor:axis2Position1", "LI-DI-SLIT-motor:axis1Position1"]  # PV nanes(LTB)
  w37 = string[] ["BTS-PS-HC-1:setI", "BTS-PS-HC-2:setI", "BTS-PS-HC-3:setI", "BTS-PS-HC-4:setI", "BTS-PS-HC-5:setI", "BTS-PS-VC-2:setI", "BTS-PS-VC-3:setI", "BTS-PS-VC-4:setI", "BTS-PS-VC-5:setI", "BTS-PS-VC-6:setI", "BTS-PS-Q1A:setI", "BTS-PS-Q1B:setI", "BTS-PS-Q1C:setI", "BTS-PS-Q2A:setI", "BTS-PS-Q2B:setI", "BTS-PS-Q2C:setI", "BTS-PS-Q3A:setI", "BTS-PS-BEND-1:setI", "BTS-PS-BEND-2:setI", "BR-PS-EXT-K1:setHV", "BR-PS-EXT-K2:setHV", "SR-PS-INJ-SE1:setHV", "SR-PS-INJ-SE2:setHV", "SR-PS-INJ-K1:setHV", "SR-PS-INJ-K2:setHV", "SR-PS-INJ-K3:setHV", "SR-PS-INJ-K4:setHV", "CPCIPM-TI-EVR:Pulse4DelaySet", "CPCIPM-TI-EVR:Pulse5DelaySet", "CPCIPM-TI-EVR:Pulse3DelaySet", "CPCIPM-TI-EVR:Pulse6DelaySet", "CPCIPM-TI-EVR:Pulse7DelaySet", "T560:setADelay", "T560:setBDelay", "T560:setCDelay", "T560:setDDelay", "CPCIPM-TI-EVR:Pulse4DelaySet", "CPCIPM-TI-EVR:Pulse5DelaySet", "BR-PS-EXT-SE1:setHV", "BR-PS-EXT-SE2:setHV", "CPCIPM-TI-EVR:Pulse3DelaySet", "CPCIPM-TI-EVR:Pulse11DelaySet"]  # PV nanes(BTS)
  w40 = FALSE ("Trip Evt B")
  (unwired) string[] ["FE-DI-XBPM-051:SA:SA_X_MONITOR", "FE-DI-XBPM-051:SA:SA_Y_MONITOR", "FE-DI-XBPM-091:SA:SA_X_MONITOR", "FE-DI-XBPM-091:SA:SA_Y_MONITOR", "FE-DI-XBPM-211:SA:SA_X_MONITOR", "FE-DI-XBPM-211:SA:SA_Y_MONITOR", "FE-DI-XBPM-231:SA:SA_X_MONITOR", "FE-DI-XBPM-231:SA:SA_Y_MONITOR", "FE-DI-XBPM-251:SA:SA_X_MONITOR", "FE-DI-XBPM-251:SA:SA_Y_MONITOR", "FE-DI-XBPM-411:SA:SA_X_MONITOR", "FE-DI-XBPM-411:SA:SA_Y_MONITOR", "FE-DI-XBPM-451:SA:SA_X_MONITOR", "FE-DI-XBPM-451:SA:SA_Y_MONITOR"]
  (unwired) string[] ["LI-VA-VAL-01:STA:POS", "LI-VA-VAL-02:STA:POS", "LI-VA-VAL-03:STA:POS", "LI-VA-VAL-04:STA:POS", "LI-VA-VAL-05:STA:POS"]
  (unwired) string[] ["SR-DI-SOFB-H:getStatus", "SR-DI-SOFB-V:getStatus", "IGPF:TPSX:FBCTRL", "IGPF:TPSY:FBCTRL", "SR-DI-FOFB-H:getStatus", "SR-DI-FOFB-V:getStatus"]
  # "V1.4.5 \n修改shift register 儲存筆數上限(之前沒有)，改成5000\n增加fill pattern的gap值\n檢查處加入ID 的mode"
  # "這3個變動太頻繁，不紀錄"
  # "PV nanes(ID gap_phase_Taper_)"
  # "PV nanes(Feedback_ILK)"
  # "V1.4.2 改成直接用最大最小值當作scale的最大最小值"
  # "1.4.1\n將BeamCurrent 圖形的Y軸上下限\n改成取最大值的1.01倍，再無條件進位取整數\n最小值的0.99倍，再無條件捨去取整數"
  # "FE-DI-XBPM-051:SA:SA_Y_MONITOR"
  # "FE-DI-XBPM-051:SA:SA_X_MONITOR"
  # "TPS-SR-052:bpm4:ilk:enabled"
  # "0 為OPEN"
  # "VALVE(EPICS)"
  n1 = local read "last ? Hrs"() -> (w50:dbl)
  n2 = Multiply(x=3600.0 ("y"), y=w50) -> (x*y=w74:dbl)
  n3 = Get Date/Time In Seconds() -> (seconds since 1Jan1904=w45:timestamp)
  n4 = Subtract(x=w45, y=w74) -> (x-y=w44:timestamp)
  n5 = call "TimeToString.vi"("Time Stamp Control"=w45) -> ("result string"=w76:string)
  n6 = call "TimeToString.vi"("Time Stamp Control"=w44) -> ("result string"=w75:string)
  n7 = call <vilib>:"Application Directory.vi"() -> ("Application Directory"=w77:path)
  n8 = Build Path(base path=w77, name or relative path="DSN\\172-18-0-32.dsn") -> (appended path=w79:path)
  n9 = call-poly <vilib>:"DB Tools Open Connection.vi"("connection information"=w79) -> ("error out"=w68:errorcluster, "connection reference"=w67:T2)  [unwired: 7 in]
  n10 = Concatenate Strings("SELECT  float_val , smpl_time\nFROM sample \nwhere  channel_id = 104 and smpl_time between '" ("result string"), w75, "' ::timestamp and '" ("result string"), w76, "' ::timestamp" ("result string")) -> (w52:string)
  n11 = call-poly <vilib>:"DB Tools Execute Query.vi"("error in (no error)"=w68, "SQL query"=w52, "connection reference"=w67) -> ("error out"=w65:errorcluster, "recordset reference"=w66:T3)  [unwired: 5 in]
  n12 = call-poly <vilib>:"DB Tools Fetch Recordset Data.vi"("error in (no error)"=w65, "recordset reference"=w66) -> ("error out"=w63:errorcluster, "recordset data"=w60:variant[][], "recordset reference out"=w64:T3)  [unwired: 3 in]
  n13 = call-poly <vilib>:"DB Tools Free Object.vi"("error in (no error)"=w63, "recordset reference"=w64) -> ("error out"=w61:errorcluster, "connection reference"=w62:T2)  [unwired: 8 in]
  n14 = Variant To Data(type=string[][] [], Variant=w60) -> (data=w58:string[][])  [unwired: 1 in, 1 out]
  n15 = call <vilib>:"DB Tools Close Connection.vi"("error in (no error)"=w61, "connection reference"=w62) -> ()  [unwired: 5 in, 1 out]
  n16 = Transpose 2D Array(2D array=w58) -> (transposed array=w56:string[][])
  n17 = Index Array(array=w56, index (row) #1=0 ("index (row)"), index (row) #2=1 ("index (row)")) -> (element #1=w70:string[], element #2=w72:string[])  [unwired: 2 in]
  n18 = Fract/Exp String To Number(string=w70) -> (number=w46:dbl[])  [unwired: 3 in, 1 out]
  n19 = Array Max & Min(array=w46) -> (max value=w42:dbl, min value=w41:dbl)  [unwired: 2 out]
  n20 = for {
    tunnel: w72 -> [w83] mode=indexing
    tunnel: [w82] -> w71 mode=indexing
    n21 = Scan From String "Scan From String"(format string="%<%Y/%m/%d %p %I:%M:%S>T", input string=w83, initial scan location=u32 0, default 1=timestamp(-73814400 s since 1904-01-01)) -> (output 1=w86:timestamp)  [unwired: 1 in, 3 out]
    n22 = To Double Precision Float(number=w86) -> (double precision float=w82:dbl)
  }
  n23 = To Double Precision Float(number=w45) -> (double precision float=w48:dbl)
  n24 = To Double Precision Float(number=w44) -> (double precision float=w47:dbl)
  n25 = control-ref of="BeamCurrent History"() -> (w49:refnum<vi>)
  n26 = property on="Property Node" class="XYGraph (strict)"(reference=w49, "XScale.Maximum"=w48, "XScale.Minimum"=w47, "YScale.Maximum"=w42, "YScale.Minimum"=w41) -> ()  [unwired: 1 in, 2 out]
  n27 = local write "Refresh B"(w40) -> ()
  n28 = local write "Trip Evt B"(w40) -> ()
  n29 = Bundle(w71, w46) -> (w51:cluster{dbl[], dbl[]})  [unwired: 1 in]
  n30 = property on="result" class="Str"("Visible"=FALSE) -> ()  [unwired: 2 in, 2 out]
  n31 = Build Array (concatenate)(w29, w30, w25) -> (w28:string[])
  n32 = Build Array (concatenate)(w23, w36, w22, w37, w38, w28, string[] ["SR-DI-FOFB-H:setStatus", "SR-DI-FOFB-V:setStatus", "IGPF:TPSX:FBCTRL", "IGPF:TPSY:FBCTRL", "TPS-SR-022:bpm3:ilk:enabled", "SR-DI-ANGLE-ILK:StatusX", "SR-DI-ANGLE-ILK:StatusY", "SR-DI-RF-FB:setStatus", "SR-ID-EPU48-TFF:status", "SR-ID-EPU48-CFF:status", "SR-ID-EPU46-TFF:status", "SR-ID-EPU46-CFF:status"], w24, w27, w26) -> (w39:string[])
  "PV list" <- w39
  n33 = call <vilib>:"Application Directory.vi"() -> ("Application Directory"=w7:path)
  n34 = Get Date/Time In Seconds() -> (seconds since 1Jan1904=w33:timestamp)
  n35 = Build Path(base path=w7, name or relative path="musics") -> (appended path=w19:path)
  n36 = To Double Precision Float(number=w33) -> (double precision float=w31:dbl)
  "Program Start Time" <- w31
  n37 = while {
    shift-right: [w261] -> _
    shift-left: _ -> [w259]
    shift-right: [w260] -> _
    shift-left: _ -> [w258]
    shift-right: [w129] -> _
    shift-left: w51 -> [w128]
    tunnel: w31 -> [w124]
    shift-right: [w105] -> _
    shift-left: _ -> [w106]
    shift-right: [w87] -> _
    shift-left: _ -> [w88]
    stop <- "stop" stop-if-true
    (unwired) string[] ["Event Time      ", "PV_name        ", "Ori_Value", "New_Value "] ("diff_Value")
    w123 = dbl[] [1.0, 1.1666666666666667, 1.3333333333333333, 1.5, 1.6666666666666665, 1.8333333333333333, 2.0, 2.142857142857143, 2.2857142857142856, 2.4285714285714284, 2.571428571428571, 2.7142857142857144, 2.857142857142857, 3.0, 3.142857142857143, 3.2857142857142856, 3.4285714285714284, 3.571428571428571, 3.7142857142857144, 3.857142857142857, 4.0, 4.125, 4.25, 4.375, 4.5, 4.625, 4.75, 4.875, 5.0, 5.125, 5.25, 5.375, 5.5, 5.625, 5.75, 5.875, 6.0, 6.142857142857143, 6.285714285714286, 6.428571428571429, 6.571428571428571, 6.714285714285714, 6.857142857142857, 7.0, 7.142857142857143, 7.285714285714286, 7.428571428571429, 7.571428571428571, 7.714285714285714, 7.857142857142857, 8.0, 8.142857142857142, 8.285714285714286, 8.428571428571429, 8.571428571428571, 8.714285714285714, 8.857142857142858, 9.0, 9.142857142857142, 9.285714285714286, 9.428571428571429, 9.571428571428571, 9.714285714285714, 9.857142857142858, 10.0, 10.142857142857142, 10.285714285714286, 10.428571428571429, 10.571428571428571, 10.714285714285714, 10.857142857142858, 11.0, 11.142857142857142, 11.285714285714286, 11.428571428571429, 11.571428571428571, 11.714285714285714, 11.857142857142858, 12.0, 12.125, 12.25, 12.375, 12.5, 12.625, 12.75, 12.875, 13.0, 13.125, 13.25, 13.375, 13.5, 13.625, 13.75, 13.875, 14.0, 14.142857142857142, 14.285714285714286, 14.428571428571429, 14.571428571428571, 14.714285714285714, 14.857142857142858, 15.0, 15.142857142857142, 15.285714285714286, 15.428571428571429, 15.571428571428571, 15.714285714285714, 15.857142857142858, 16.0, 16.142857142857142, 16.285714285714285, 16.428571428571427, 16.571428571428573, 16.714285714285715, 16.857142857142858, 17.0, 17.142857142857142, 17.285714285714285, 17.428571428571427, 17.571428571428573, 17.714285714285715, 17.857142857142858, 18.0, 18.142857142857142, 18.285714285714285, 18.428571428571427, 18.571428571428573, 18.714285714285715, 18.857142857142858, 19.0, 19.142857142857142, 19.285714285714285, 19.428571428571427, 19.571428571428573, 19.714285714285715, 19.857142857142858, 20.0, 20.125, 20.25, 20.375, 20.5, 20.625, 20.75, 20.875, 21.0, 21.125, 21.25, 21.375, 21.5, 21.625, 21.75, 21.875, 22.0, 22.142857142857142, 22.285714285714285, 22.428571428571427, 22.571428571428573, 22.714285714285715, 22.857142857142858, 23.0, 23.142857142857142, 23.285714285714285, 23.428571428571427, 23.571428571428573, 23.714285714285715, 23.857142857142858, 24.0, 24.166666666666668, 24.333333333333332, 24.5, 24.666666666666668, 24.833333333333332]  # Array of X axis  平均分配至各段
    w154 = string[] ["SR-ID-IU22-05:setECMode", "SR-ID-IU22A-09:setECMode", "SR-ID-IU22B-09:setECMode", "SR-ID-IUT22-21:setECMode", "SR-ID-IU22-23:setECMode", "SR-ID-IU22A-25:setECMode", "SR-ID-IU22B-25:setECMode", "SR-ID-EPU48A-41:setECMode", "SR-ID-EPU48B-41:setECMode", "SR-ID-EPU46-45:setECMode"]  # ID_mode
    w240 = string[] ["FE-05-PAB:Open", "FE-05-MGV:Open", "FE-05-FCV:Open", "FE-09-PAB:Open", "FE-09-MGV:Open", "FE-09-FCV:Open", "FE-21-PAB:Open", "FE-21-MGV:Open", "FE-21-FCV:Open", "FE-23-PAB:Open", "FE-23-PAB:Open", "FE-23-FCV:Open", "FE-25-PAB:Open", "FE-25-MGV:Open", "FE-25-FCV:Open", "FE-41-PAB:Open", "FE-41-MGV:Open", "FE-41-FCV:Open", "FE-45-PAB:Open", "FE-45-MGV:Open", "FE-45-FCV:Open"]  # PAB_MGV_FCV enable
    (unwired) "LI-DI-WCM:getWfCh1"
    (unwired) "SR-DI-FP:CurrentBuffer"
    w375 = 0.001
    w373 = string[] ["SR-DI-BPM-011:Y", "SR-DI-BPM-012:Y", "SR-DI-BPM-013:Y", "SR-DI-BPM-014:Y", "SR-DI-BPM-015:Y", "SR-DI-BPM-016:Y", "SR-DI-BPM-017:Y", "SR-DI-BPM-021:Y", "SR-DI-BPM-022:Y", "SR-DI-BPM-023:Y", "SR-DI-BPM-024:Y", "SR-DI-BPM-025:Y", "SR-DI-BPM-026:Y", "SR-DI-BPM-027:Y", "SR-DI-BPM-031:Y", "SR-DI-BPM-032:Y", "SR-DI-BPM-033:Y", "SR-DI-BPM-034:Y", "SR-DI-BPM-035:Y", "SR-DI-BPM-036:Y", "SR-DI-BPM-037:Y", "SR-DI-BPM-041:Y", "SR-DI-BPM-042:Y", "SR-DI-BPM-043:Y", "SR-DI-BPM-044:Y", "SR-DI-BPM-045:Y", "SR-DI-BPM-046:Y", "SR-DI-BPM-047:Y", "SR-DI-BPM-048:Y", "SR-DI-BPM-050:Y", "SR-DI-BPM-051:Y", "SR-DI-BPM-052:Y", "SR-DI-BPM-053:Y", "SR-DI-BPM-054:Y", "SR-DI-BPM-055:Y", "SR-DI-BPM-056:Y", "SR-DI-BPM-057:Y", "SR-DI-BPM-061:Y", "SR-DI-BPM-062:Y", "SR-DI-BPM-063:Y", "SR-DI-BPM-064:Y", "SR-DI-BPM-065:Y", "SR-DI-BPM-066:Y", "SR-DI-BPM-067:Y", "SR-DI-BPM-071:Y", "SR-DI-BPM-072:Y", "SR-DI-BPM-073:Y", "SR-DI-BPM-074:Y", "SR-DI-BPM-075:Y", "SR-DI-BPM-076:Y", "SR-DI-BPM-077:Y", "SR-DI-BPM-081:Y", "SR-DI-BPM-082:Y", "SR-DI-BPM-083:Y", "SR-DI-BPM-084:Y", "SR-DI-BPM-085:Y", "SR-DI-BPM-086:Y", "SR-DI-BPM-087:Y", "SR-DI-BPM-091:Y", "SR-DI-BPM-092:Y", "SR-DI-BPM-093:Y", "SR-DI-BPM-094:Y", "SR-DI-BPM-095:Y", "SR-DI-BPM-096:Y", "SR-DI-BPM-097:Y", "SR-DI-BPM-101:Y", "SR-DI-BPM-102:Y", "SR-DI-BPM-103:Y", "SR-DI-BPM-104:Y", "SR-DI-BPM-105:Y", "SR-DI-BPM-106:Y", "SR-DI-BPM-107:Y", "SR-DI-BPM-111:Y", "SR-DI-BPM-112:Y", "SR-DI-BPM-113:Y", "SR-DI-BPM-114:Y", "SR-DI-BPM-115:Y", "SR-DI-BPM-116:Y", "SR-DI-BPM-117:Y", "SR-DI-BPM-121:Y", "SR-DI-BPM-122:Y", "SR-DI-BPM-123:Y", "SR-DI-BPM-124:Y", "SR-DI-BPM-125:Y", "SR-DI-BPM-126:Y", "SR-DI-BPM-127:Y", "SR-DI-BPM-128:Y", "SR-DI-BPM-130:Y", "SR-DI-BPM-131:Y", "SR-DI-BPM-132:Y", "SR-DI-BPM-133:Y", "SR-DI-BPM-134:Y", "SR-DI-BPM-135:Y", "SR-DI-BPM-136:Y", "SR-DI-BPM-137:Y", "SR-DI-BPM-141:Y", "SR-DI-BPM-142:Y", "SR-DI-BPM-143:Y", "SR-DI-BPM-144:Y", "SR-DI-BPM-145:Y", "SR-DI-BPM-146:Y", "SR-DI-BPM-147:Y", "SR-DI-BPM-151:Y", "SR-DI-BPM-152:Y", "SR-DI-BPM-153:Y", "SR-DI-BPM-154:Y", "SR-DI-BPM-155:Y", "SR-DI-BPM-156:Y", "SR-DI-BPM-157:Y", "SR-DI-BPM-161:Y", "SR-DI-BPM-162:Y", "SR-DI-BPM-163:Y", "SR-DI-BPM-164:Y", "SR-DI-BPM-165:Y", "SR-DI-BPM-166:Y", "SR-DI-BPM-167:Y", "SR-DI-BPM-171:Y", "SR-DI-BPM-172:Y", "SR-DI-BPM-173:Y", "SR-DI-BPM-174:Y", "SR-DI-BPM-175:Y", "SR-DI-BPM-176:Y", "SR-DI-BPM-177:Y", "SR-DI-BPM-181:Y", "SR-DI-BPM-182:Y", "SR-DI-BPM-183:Y", "SR-DI-BPM-184:Y", "SR-DI-BPM-185:Y", "SR-DI-BPM-186:Y", "SR-DI-BPM-187:Y", "SR-DI-BPM-191:Y", "SR-DI-BPM-192:Y", "SR-DI-BPM-193:Y", "SR-DI-BPM-194:Y", "SR-DI-BPM-195:Y", "SR-DI-BPM-196:Y", "SR-DI-BPM-197:Y", "SR-DI-BPM-201:Y", "SR-DI-BPM-202:Y", "SR-DI-BPM-203:Y", "SR-DI-BPM-204:Y", "SR-DI-BPM-205:Y", "SR-DI-BPM-206:Y", "SR-DI-BPM-207:Y", "SR-DI-BPM-208:Y", "SR-DI-BPM-210:Y", "SR-DI-BPM-211:Y", "SR-DI-BPM-212:Y", "SR-DI-BPM-213:Y", "SR-DI-BPM-214:Y", "SR-DI-BPM-215:Y", "SR-DI-BPM-216:Y", "SR-DI-BPM-217:Y", "SR-DI-BPM-221:Y", "SR-DI-BPM-222:Y", "SR-DI-BPM-223:Y", "SR-DI-BPM-224:Y", "SR-DI-BPM-225:Y", "SR-DI-BPM-226:Y", "SR-DI-BPM-227:Y", "SR-DI-BPM-231:Y", "SR-DI-BPM-232:Y", "SR-DI-BPM-233:Y", "SR-DI-BPM-234:Y", "SR-DI-BPM-235:Y", "SR-DI-BPM-236:Y", "SR-DI-BPM-237:Y", "SR-DI-BPM-241:Y", "SR-DI-BPM-242:Y", "SR-DI-BPM-243:Y", "SR-DI-BPM-244:Y", "SR-DI-BPM-245:Y", "SR-DI-BPM-246:Y", "SR-DI-BPM-247:Y"]  # sorted BPMY_174
    w372 = string[] ["SR-DI-BPM-011:X", "SR-DI-BPM-012:X", "SR-DI-BPM-013:X", "SR-DI-BPM-014:X", "SR-DI-BPM-015:X", "SR-DI-BPM-016:X", "SR-DI-BPM-017:X", "SR-DI-BPM-021:X", "SR-DI-BPM-022:X", "SR-DI-BPM-023:X", "SR-DI-BPM-024:X", "SR-DI-BPM-025:X", "SR-DI-BPM-026:X", "SR-DI-BPM-027:X", "SR-DI-BPM-031:X", "SR-DI-BPM-032:X", "SR-DI-BPM-033:X", "SR-DI-BPM-034:X", "SR-DI-BPM-035:X", "SR-DI-BPM-036:X", "SR-DI-BPM-037:X", "SR-DI-BPM-041:X", "SR-DI-BPM-042:X", "SR-DI-BPM-043:X", "SR-DI-BPM-044:X", "SR-DI-BPM-045:X", "SR-DI-BPM-046:X", "SR-DI-BPM-047:X", "SR-DI-BPM-048:X", "SR-DI-BPM-050:X", "SR-DI-BPM-051:X", "SR-DI-BPM-052:X", "SR-DI-BPM-053:X", "SR-DI-BPM-054:X", "SR-DI-BPM-055:X", "SR-DI-BPM-056:X", "SR-DI-BPM-057:X", "SR-DI-BPM-061:X", "SR-DI-BPM-062:X", "SR-DI-BPM-063:X", "SR-DI-BPM-064:X", "SR-DI-BPM-065:X", "SR-DI-BPM-066:X", "SR-DI-BPM-067:X", "SR-DI-BPM-071:X", "SR-DI-BPM-072:X", "SR-DI-BPM-073:X", "SR-DI-BPM-074:X", "SR-DI-BPM-075:X", "SR-DI-BPM-076:X", "SR-DI-BPM-077:X", "SR-DI-BPM-081:X", "SR-DI-BPM-082:X", "SR-DI-BPM-083:X", "SR-DI-BPM-084:X", "SR-DI-BPM-085:X", "SR-DI-BPM-086:X", "SR-DI-BPM-087:X", "SR-DI-BPM-091:X", "SR-DI-BPM-092:X", "SR-DI-BPM-093:X", "SR-DI-BPM-094:X", "SR-DI-BPM-095:X", "SR-DI-BPM-096:X", "SR-DI-BPM-097:X", "SR-DI-BPM-101:X", "SR-DI-BPM-102:X", "SR-DI-BPM-103:X", "SR-DI-BPM-104:X", "SR-DI-BPM-105:X", "SR-DI-BPM-106:X", "SR-DI-BPM-107:X", "SR-DI-BPM-111:X", "SR-DI-BPM-112:X", "SR-DI-BPM-113:X", "SR-DI-BPM-114:X", "SR-DI-BPM-115:X", "SR-DI-BPM-116:X", "SR-DI-BPM-117:X", "SR-DI-BPM-121:X", "SR-DI-BPM-122:X", "SR-DI-BPM-123:X", "SR-DI-BPM-124:X", "SR-DI-BPM-125:X", "SR-DI-BPM-126:X", "SR-DI-BPM-127:X", "SR-DI-BPM-128:X", "SR-DI-BPM-130:X", "SR-DI-BPM-131:X", "SR-DI-BPM-132:X", "SR-DI-BPM-133:X", "SR-DI-BPM-134:X", "SR-DI-BPM-135:X", "SR-DI-BPM-136:X", "SR-DI-BPM-137:X", "SR-DI-BPM-141:X", "SR-DI-BPM-142:X", "SR-DI-BPM-143:X", "SR-DI-BPM-144:X", "SR-DI-BPM-145:X", "SR-DI-BPM-146:X", "SR-DI-BPM-147:X", "SR-DI-BPM-151:X", "SR-DI-BPM-152:X", "SR-DI-BPM-153:X", "SR-DI-BPM-154:X", "SR-DI-BPM-155:X", "SR-DI-BPM-156:X", "SR-DI-BPM-157:X", "SR-DI-BPM-161:X", "SR-DI-BPM-162:X", "SR-DI-BPM-163:X", "SR-DI-BPM-164:X", "SR-DI-BPM-165:X", "SR-DI-BPM-166:X", "SR-DI-BPM-167:X", "SR-DI-BPM-171:X", "SR-DI-BPM-172:X", "SR-DI-BPM-173:X", "SR-DI-BPM-174:X", "SR-DI-BPM-175:X", "SR-DI-BPM-176:X", "SR-DI-BPM-177:X", "SR-DI-BPM-181:X", "SR-DI-BPM-182:X", "SR-DI-BPM-183:X", "SR-DI-BPM-184:X", "SR-DI-BPM-185:X", "SR-DI-BPM-186:X", "SR-DI-BPM-187:X", "SR-DI-BPM-191:X", "SR-DI-BPM-192:X", "SR-DI-BPM-193:X", "SR-DI-BPM-194:X", "SR-DI-BPM-195:X", "SR-DI-BPM-196:X", "SR-DI-BPM-197:X", "SR-DI-BPM-201:X", "SR-DI-BPM-202:X", "SR-DI-BPM-203:X", "SR-DI-BPM-204:X", "SR-DI-BPM-205:X", "SR-DI-BPM-206:X", "SR-DI-BPM-207:X", "SR-DI-BPM-208:X", "SR-DI-BPM-210:X", "SR-DI-BPM-211:X", "SR-DI-BPM-212:X", "SR-DI-BPM-213:X", "SR-DI-BPM-214:X", "SR-DI-BPM-215:X", "SR-DI-BPM-216:X", "SR-DI-BPM-217:X", "SR-DI-BPM-221:X", "SR-DI-BPM-222:X", "SR-DI-BPM-223:X", "SR-DI-BPM-224:X", "SR-DI-BPM-225:X", "SR-DI-BPM-226:X", "SR-DI-BPM-227:X", "SR-DI-BPM-231:X", "SR-DI-BPM-232:X", "SR-DI-BPM-233:X", "SR-DI-BPM-234:X", "SR-DI-BPM-235:X", "SR-DI-BPM-236:X", "SR-DI-BPM-237:X", "SR-DI-BPM-241:X", "SR-DI-BPM-242:X", "SR-DI-BPM-243:X", "SR-DI-BPM-244:X", "SR-DI-BPM-245:X", "SR-DI-BPM-246:X", "SR-DI-BPM-247:X"]  # sorted BPMX_174
    w431 = string[] ["BL-05A:HutchA_Enable", "BL-09A:HutchA_Enable", "BL-21A:HutchA_Enable", "BL-23A:HutchA_Enable", "BL-25A:HutchA_Enable", "BL-41A:HutchA_Enable", "BL-45A:HutchA_Enable"]  # Hutch enable
    w450 = string[] ["CPCI03-adl7452-0:doBank0Ch5", "CPCI05-adl7452-0:doBank0Ch5", "CPCI11-adl7452-0:doBank0Ch5", "CPCI12-adl7452-0:doBank0Ch5", "CPCI13-adl7452-0:doBank0Ch5", "CPCI21-adl7452-0:doBank0Ch5", "CPCI23-adl7452-0:doBank0Ch5"]  # FE enable
    w527 = 578.303 ("y")
    w532 = 1.202 ("y")
    # "SR-DI-RF-FB:getStatus"
    # "V1.4.2 改成直接用最大最小值當作scale的最大最小值"
    # "D:\\LOG運轉紀錄\\2016"
    # "45"
    # "41"
    # "25"
    # "23"
    # "21"
    # "09"
    # "05"
    # "05\n09\n21\n23\n25\n41\n45"
    # "gapMotorOff"
    n38 = event shown="[10] \"Save Button\": Value Change" {
      selector: _ -> [_ _ _ _ _ _ _ _ _ _ _]
      dyn-events: _ -> [_ _ _ _ _ _ _ _ _ _ _]
      timeout: 233 -> [_ _ _ _ _ _ _ _ _ _ _]
      tunnel: [_ w592 _ _ _ _ _ _ _ _ _] -> w130
      tunnel: [w578 w591 w598 w612 w649 w656 w683 w695 w721 w752 w773] -> w129
      tunnel: w128 -> [w578 w591 w598 _ w649 _ w683 w695 w721 w752 w773]
      tunnel: "last ? Hrs" -> [_ _ _ w619 _ w657 _ _ _ _ _]
      tunnel: w124 -> [_ w579 _ _ _ _ _ w694 _ w746 w757]
      tunnel: "T:Slow\nF:Fast" -> [_ _ _ w615 _ w652 _ _ _ _ _]
      tunnel: 0.004 ("最新時間") -> [_ _ _ w614 _ w651 _ _ _ _ _]
      event Timeout {
        n39 = event-data() -> ()  [unwired: 1 in, 3 out]
      }
      event "stop": Value Change {
        n40 = event-data() -> ("NewVal"=w592:bool)  [unwired: 1 in, 3 out]
        n41 = Get Date/Time In Seconds() -> (seconds since 1Jan1904=w585:timestamp)
        n42 = To Double Precision Float(number=w585) -> (double precision float=w584:dbl)
        n43 = Subtract(x=w584, y=43200.0) -> (x-y=w581:dbl)
        n44 = call "Main_Daily_path.vi"() -> ("Directory path"=w586:path)  [unwired: 10 in, 1 out]
        n45 = Greater?(x=w581, y=w579) -> (0:w582:bool)
        n46 = Select(t=w581, s=w582, f=w579) -> ()  [unwired: 1 out]
        n47 = call "B09_Save_new_lattice_files.vi"("For Test"=TRUE, "Directory Path"=w586) -> ()  [unwired: 10 in]
        n48 = call <vilib>:"Application Directory.vi"() -> ("Application Directory"=w580:path)
        n49 = local read "Diff list"() -> (w589:string[][])
        n50 = call "B07_Save_changed_PVs.vi"("For Test"=FALSE, "想要限制的筆數"=1000, "Directory Path"=w580, "紀錄起始時間  門檻"=w579, "diff_Value 2"=w589) -> ()  [unwired: 5 in, 2 out]
      }
      event "Open Button": Value Change {
        n51 = event-data() -> ()  [unwired: 1 in, 6 out]
        n52 = call <vilib>:"Beep.vi"("use system alert? (T)"=FALSE, "duration (msec)"=u32 40, "frequency (Hz)"=u32 1700) -> ()  [unwired: 9 in]
        n53 = call "Main_Daily_path.vi"() -> ("Directory path(STR)"=w597:string, "Directory path"=w596:path)  [unwired: 10 in]
        n54 = call <vilib>:"Check if File or Folder Exists.vi"("path"=w596) -> ("error out"=w602:errorcluster, "file or folder exists?"=w600:bool, "dup path"=w601:path)  [unwired: 8 in]
        n55 = case shown="False" w600 {
          tunnel: w601 -> [w609 w611]
          tunnel: w602 -> [w608 w610]
          tunnel: [w607 w611] -> _
          tunnel: [w606 w610] -> w599
          frame False {
            n56 = Create Folder(path (use dialog)=w609, error in=w608) -> (created path=w607:path, error out=w606:errorcluster)  [unwired: 1 in, 1 out]
          }
          frame True {
          }
        }
        n57 = Concatenate Strings("explorer ", w597) -> (w604:string)
        n58 = call <vilib>:"System Exec.vi"("wait until completion? (T)"=FALSE, "error in (no error)"=w599, "command line"=w604) -> ()  [unwired: 5 in, 4 out]
      }
      event "Trip Evt B": Value Change {
        n59 = event-data() -> ()  [unwired: 1 in, 1 out]
        n60 = flat-sequence {
          tunnel: w619 -> [w626]
          tunnel: [w626] -> w617
          tunnel: [w621] -> w616
          tunnel: w615 -> [w621]
          tunnel: w614 -> [w620]
          tunnel: [w620] -> w613
          tunnel: [w627] -> w618
          tunnel: w617 -> [w638]
          tunnel: w616 -> [w637]
          tunnel: w613 -> [w636]
          tunnel: [w644] -> w612
          tunnel: w618 -> [w644]
          frame #0 {
            n61 = property on="result" class="Str"("Visible"=FALSE) -> ()  [unwired: 2 in, 2 out]
            n62 = call <vilib>:"Beep.vi"("use system alert? (T)"=FALSE, "duration (msec)"=u32 40, "frequency (Hz)"=u32 1700) -> ()  [unwired: 9 in]
          }
          frame #1 {
            n63 = call "sub_plot_beamCurrent_and_trip_events.vi"("要看前幾個小時"=w638, "最新時間"=w636, "T:Slow\nF:Fast"=w637) -> ("Y min value"=w629:dbl, "Y max value"=w630:dbl, "X min value"=w631:dbl, "X max value"=w632:dbl, "BeamCurrent History"=w634:cluster{dbl[], dbl[]}[], "result"=→"result":string)  [unwired: 3 in]
            n64 = control-ref of="BeamCurrent History"() -> (w628:refnum<vi>)
            n65 = Index Array(array=w634, index=1) -> (element=w627:cluster{dbl[], dbl[]})
            n66 = property on="Property Node" class="XYGraph (strict)"(reference=w628, "XScale.Maximum"=w632, "XScale.Minimum"=w631, "YScale.Maximum"=w630, "YScale.Minimum"=w629) -> ()  [unwired: 1 in, 2 out]
          }
          frame #2 {
            n67 = local write "Trip Evt B"(FALSE ("Trip Evt B")) -> ()
            n68 = property on="result" class="Str"("Visible"=TRUE) -> ()  [unwired: 2 in, 2 out]
            n69 = call <vilib>:"Beep.vi"("use system alert? (T)"=FALSE, "duration (msec)"=u32 40, "frequency (Hz)"=u32 2000) -> ()  [unwired: 9 in]
          }
        }
      }
      event "Switch Tab": Value Change {
        n70 = event-data() -> ("NewVal"=w648:bool)  [unwired: 1 in, 1 out]
        n71 = Select(t=enum32{"_____", "           "}."_____" ("Tab Control"), s=w648, f=enum32{"_____", "           "}."           " ("Tab Control")) -> (s? t:f=→"Tab Control":enum32{"_____", "           "})
      }
      event "Refresh B": Value Change {
        n72 = event-data() -> ()  [unwired: 1 in, 6 out]
        n73 = flat-sequence {
          tunnel: w657 -> [w664]
          tunnel: [w664] -> w654
          tunnel: [w659] -> w653
          tunnel: w652 -> [w659]
          tunnel: w651 -> [w658]
          tunnel: [w658] -> w650
          tunnel: [w665] -> w655
          tunnel: w654 -> [w673]
          tunnel: w653 -> [w675]
          tunnel: w650 -> [w674]
          tunnel: [w682] -> w656
          tunnel: w655 -> [w682]
          frame #0 {
            n74 = property on="result" class="Str"("Visible"=FALSE) -> ()  [unwired: 2 in, 2 out]
            n75 = call <vilib>:"Beep.vi"("use system alert? (T)"=FALSE, "duration (msec)"=u32 40, "frequency (Hz)"=u32 1700) -> ()  [unwired: 9 in]
          }
          frame #1 {
            # "032  OPStatus    2195\n037  OPStatus    1899"
            n76 = call "sub_plot_beamCurrent_and_trip_events.vi"("要看前幾個小時"=w673, "最新時間"=w674, "T:Slow\nF:Fast"=w675) -> ("Y min value"=w669:dbl, "Y max value"=w670:dbl, "X min value"=w671:dbl, "X max value"=w672:dbl, "BeamCurrent History"=w667:cluster{dbl[], dbl[]}[], "result"=w668:string)  [unwired: 3 in]
            n77 = local write "result"(w668) -> ()
            n78 = control-ref of="BeamCurrent History"() -> (w676:refnum<vi>)
            n79 = property on="Property Node" class="XYGraph (strict)"(reference=w676, "XScale.Maximum"=w672, "XScale.Minimum"=w671, "YScale.Maximum"=w670, "YScale.Minimum"=w669) -> ()  [unwired: 1 in, 2 out]
            n80 = Index Array(array=w667, index=1) -> (element=w665:cluster{dbl[], dbl[]})
          }
          frame #2 {
            n81 = local write "Refresh B"(FALSE ("Trip Evt B")) -> ()
            n82 = property on="result" class="Str"("Visible"=TRUE) -> ()  [unwired: 2 in, 2 out]
            n83 = call <vilib>:"Beep.vi"("use system alert? (T)"=FALSE, "duration (msec)"=u32 40, "frequency (Hz)"=u32 2000) -> ()  [unwired: 9 in]
          }
        }
      }
      event "Save Lattice Button": Value Change {
        n84 = event-data() -> ()  [unwired: 1 in, 2 out]
        n85 = flat-sequence {
          frame #0 {
            n86 = call <vilib>:"Beep.vi"("use system alert? (T)"=FALSE, "duration (msec)"=u32 40, "frequency (Hz)"=u32 1700) -> ()  [unwired: 9 in]
          }
          frame #1 {
            n87 = call "Main_Daily_path.vi"() -> ("Directory path"=w687:path)  [unwired: 10 in, 1 out]
            n88 = call "B09_Save_new_lattice_files.vi"("For Test"=FALSE, "Directory Path"=w687) -> ()  [unwired: 10 in]
          }
          frame #2 {
            n89 = call <vilib>:"Beep.vi"("use system alert? (T)"=FALSE, "duration (msec)"=u32 40, "frequency (Hz)"=u32 2000) -> ()  [unwired: 9 in]
          }
        }
      }
      event "View Diff Button": Value Change {
        n90 = event-data() -> ()  [unwired: 1 in, 1 out]
        n91 = flat-sequence {
          tunnel: w694 -> [w700]
          tunnel: [w706] -> w692
          tunnel: [w711] -> w693
          tunnel: w692 -> [w711]
          tunnel: w693 -> [w713]
          frame #0 {
            # "12小時為43200sec"
            # "Save file"
            n92 = Get Date/Time In Seconds() -> (seconds since 1Jan1904=w705:timestamp)
            n93 = To Double Precision Float(number=w705) -> (double precision float=w704:dbl)
            n94 = call <vilib>:"Beep.vi"("use system alert? (T)"=FALSE, "duration (msec)"=u32 40, "frequency (Hz)"=u32 1700) -> ()  [unwired: 9 in]
            n95 = Subtract(x=w704, y=43200.0) -> (x-y=w701:dbl)
            n96 = Greater?(x=w701, y=w700) -> (0:w702:bool)
            n97 = Select(t=w701, s=w702, f=w700) -> (s? t:f=w699:dbl)
            n98 = local read "Diff list"() -> (w710:string[][])
            n99 = call "Main_Daily_path.vi"() -> ("Directory path"=w709:path)  [unwired: 10 in, 1 out]
            n100 = call "B07_Save_changed_PVs.vi"("For Test"=FALSE, "想要限制的筆數"=1000, "Directory Path"=w709, "紀錄起始時間  門檻"=w699, "diff_Value 2"=w710) -> ("saved file path"=w706:path)  [unwired: 5 in, 1 out]
          }
          frame #1 {
            # "Wait"
            n101 = Wait (ms)(milliseconds to wait=u32 300) -> ()  [unwired: 1 out]
          }
          frame #2 {
            # "Show"
            n102 = Path To String(path=w713) -> (string=w715:string)
            n103 = Concatenate Strings("explorer ", w715) -> (w714:string)
            n104 = call <vilib>:"System Exec.vi"("command line"=w714) -> ()  [unwired: 7 in, 4 out]
          }
          frame #3 {
            n105 = local write "View Diff Button"(FALSE ("View Diff Button")) -> ()
            n106 = call <vilib>:"Beep.vi"("use system alert? (T)"=FALSE, "duration (msec)"=u32 40, "frequency (Hz)"=u32 2000) -> ()  [unwired: 9 in]
          }
        }
      }
      event "Show Check list Button": Value Change {
        n107 = event-data() -> ()  [unwired: 1 in, 1 out]
        n108 = flat-sequence {
          frame #0 {
            n109 = call <vilib>:"Beep.vi"("use system alert? (T)"=FALSE, "duration (msec)"=u32 40, "frequency (Hz)"=u32 1700) -> ()  [unwired: 9 in]
          }
          frame #1 {
            n110 = local read "PV list"() -> (w725:string[])
            n111 = Array Size(array=w725) -> (size(s)=w726:i32)
            n112 = Array To Spreadsheet String(delimiter (Tab)="</BR>\n\r", array=w725, 3:"%s" ("format string")) -> (spreadsheet string=w737:string)
            n113 = Number To Decimal String(number=w726) -> (decimal integer string=w736:string)  [unwired: 1 in]
            n114 = call <vilib>:"Application Directory.vi"() -> ("Application Directory"=w727:path)
            n115 = Concatenate Strings("Tatal Checked PVs: ", w736, "</BR>\n\r" ("string"), w737) -> (w738:string)
            n116 = Build Path(base path=w727, name or relative path="Checked PV list.html") -> (appended path=w739:path)
            n117 = Write to Text File(file (use dialog)=w739, text=w738) -> ()  [unwired: 2 in, 3 out]
            n118 = flat-sequence {
              tunnel: w739 -> [w741]
              tunnel: [w741] -> w740
              frame #0 {
                n119 = Wait (ms)(milliseconds to wait=u32 500) -> ()  [unwired: 1 out]
              }
            }
            n120 = Path To String(path=w740) -> (string=w730:string)
            n121 = Concatenate Strings("explorer ", w730) -> (w729:string)
            n122 = call <vilib>:"System Exec.vi"("command line"=w729) -> ()  [unwired: 7 in, 4 out]
          }
          frame #2 {
            n123 = call <vilib>:"Beep.vi"("use system alert? (T)"=FALSE, "duration (msec)"=u32 40, "frequency (Hz)"=u32 2000) -> ()  [unwired: 9 in]
          }
        }
      }
      event Panel Close? {
        n124 = event-data() -> ()  [unwired: 1 in, 4 out]
        n125 = call "Main_Daily_path.vi"() -> ("Directory path"=w748:path)  [unwired: 10 in, 1 out]
        n126 = call "B09_Save_new_lattice_files.vi"("For Test"=TRUE, "Directory Path"=w748) -> ()  [unwired: 10 in]
        n127 = call <vilib>:"Application Directory.vi"() -> ("Application Directory"=w747:path)
        n128 = local read "Diff list"() -> (w751:string[][])
        n129 = call "B07_Save_changed_PVs.vi"("For Test"=FALSE, "想要限制的筆數"=1000, "Directory Path"=w747, "紀錄起始時間  門檻"=w746, "diff_Value 2"=w751) -> ()  [unwired: 5 in, 2 out]
        n130 = event-data() -> ()  [unwired: 2 in, 1 out]
      }
      event "Save Button": Value Change {
        n131 = event-data() -> ()  [unwired: 1 in, 1 out]
        n132 = Get Date/Time In Seconds() -> (seconds since 1Jan1904=w763:timestamp)
        n133 = To Double Precision Float(number=w763) -> (double precision float=w762:dbl)
        n134 = call <vilib>:"Beep.vi"("use system alert? (T)"=FALSE, "duration (msec)"=u32 40, "frequency (Hz)"=u32 1700) -> ()  [unwired: 9 in]
        n135 = Subtract(x=w762, y=43200.0) -> (x-y=w759:dbl)
        n136 = Greater?(x=w759, y=w757) -> (0:w760:bool)
        n137 = Select(t=w759, s=w760, f=w757) -> (s? t:f=w758:dbl)
        n138 = local read "Diff list"() -> (w767:string[][])
        n139 = call "Main_Daily_path.vi"() -> ("Directory path"=w766:path)  [unwired: 10 in, 1 out]
        n140 = call "B07_Save_changed_PVs.vi"("For Test"=FALSE, "想要限制的筆數"=1000, "Directory Path"=w766, "紀錄起始時間  門檻"=w758, "diff_Value 2"=w767) -> ()  [unwired: 5 in, 2 out]
        n141 = Get Date/Time In Seconds() -> (seconds since 1Jan1904=w775:timestamp)
        n142 = Format Date/Time String(time format string (%c)="%Y", seconds (now)=w775, UTC format=FALSE) -> (date/time string=w793:string)
        n143 = Format Date/Time String(time format string (%c)="%d", seconds (now)=w775, UTC format=FALSE) -> (date/time string=w802:string)
        n144 = call "to_be_2_string.vi"("string 2"=w802) -> ("substring 2"=w803:string)  [unwired: 10 in]
        n145 = Format Date/Time String(time format string (%c)="%m", seconds (now)=w775, UTC format=FALSE) -> (date/time string=w797:string)
        n146 = Format Date/Time String(time format string (%c)="%Y%m%d%H%M%S", seconds (now)=w775) -> (date/time string=w781:string)  [unwired: 1 in]
        n147 = Concatenate Strings("D" ("磁碟位置"), ":\\LOG運轉紀錄\\", w793, "\\", w797, "\\", w803) -> (w786:string)
        n148 = String To Path(string=w786) -> (path=w789:path)
        n149 = call <vilib>:"Check if File or Folder Exists.vi"("path"=w789) -> ("error out"=w787:errorcluster, "file or folder exists?"=w801:bool, "dup path"=w788:path)  [unwired: 8 in]
        n150 = invoke on="Cluster" class="Clust (strict)" method="Get Image"() -> ("image data"=w756:T4)  [unwired: 6 in, 5 out]
        n151 = case shown="False" w801 {
          tunnel: w788 -> [w814 w816]
          tunnel: w787 -> [w813 w815]
          tunnel: [w812 w816] -> w774
          tunnel: [w811 w815] -> _
          frame False {
            n152 = Create Folder(path (use dialog)=w814, error in=w813) -> (created path=w812:path, error out=w811:errorcluster)  [unwired: 1 in, 1 out]
          }
          frame True {
          }
        }
        n153 = Path To String(path=w774) -> (string=w785:string)
        n154 = call "Main_Daily_path.vi"() -> ("Directory path"=w768:path)  [unwired: 10 in, 1 out]
        n155 = Concatenate Strings(w785, "\\" ("string"), w781) -> (w776:string)
        n156 = call "B09_Save_new_lattice_files.vi"("For Test"=FALSE, "Directory Path"=w768) -> ()  [unwired: 10 in]
        n157 = Concatenate Strings(w776, ".jpg" ("file format")) -> (w777:string)
        n158 = String To Path(string=w777) -> (path=w780:path)
        n159 = call <vilib>:"Draw Flattened Pixmap.vi"("image data"=w756) -> ("new picture"=w754:picture)  [unwired: 8 in]
        "new picture" <- w754
        n160 = call <vilib>:"Write JPEG File.vi"("quality (80)"=100, "image data"=w756, "path to JPEG file"=w780) -> ("error out"=w755:errorcluster)  [unwired: 7 in, 1 out]
        "error out 3" <- w755
        n161 = flat-sequence {
          tunnel: w755 -> [w806]
          tunnel: w754 -> [_]
          frame #0 {
            n162 = Temporary Directory() -> (w805:path)
            n163 = control-ref of="new picture"() -> (w810:refnum<vi>)
            n164 = invoke class="Pict" method="Export Image"(reference=w810, error in=w806, "File Type"=enum32{"BMP", "EPS", "EMF", "PICT"}."BMP", "Target"=enum32{"File", "Clipboard"}."Clipboard", "Path"=w805, "Hide Grid"=TRUE ("Always Overwrite")) -> (error out=→"error out":errorcluster)  [unwired: 1 in, 6 out]
          }
        }
      }
    }
    n165 = call-poly <userlib>:"CaLabGet.vi"("PV Names"=string[] ["FE-DI-XBPM-051:signals:sa.X", "FE-DI-XBPM-051:signals:sa.Y", "FE-DI-XBPM-091:SA:SA_X_MONITOR", "FE-DI-XBPM-091:SA:SA_Y_MONITOR", "FE-DI-XBPM-211:SA:SA_X_MONITOR", "FE-DI-XBPM-211:SA:SA_Y_MONITOR", "FE-DI-XBPM-231:SA:SA_X_MONITOR", "FE-DI-XBPM-231:SA:SA_Y_MONITOR", "FE-DI-XBPM-251:SA:SA_X_MONITOR", "FE-DI-XBPM-251:SA:SA_Y_MONITOR", "FE-DI-XBPM-411:SA:SA_X_MONITOR", "FE-DI-XBPM-411:SA:SA_Y_MONITOR", "FE-DI-XBPM-451:SA:SA_X_MONITOR", "FE-DI-XBPM-451:SA:SA_Y_MONITOR", "FE-DI-XBPM-052:signals:sa.X", "FE-DI-XBPM-052:signals:sa.Y", "FE-DI-XBPM-092:SA:SA_X_MONITOR", "FE-DI-XBPM-092:SA:SA_Y_MONITOR", "FE-DI-XBPM-212:SA:SA_X_MONITOR", "FE-DI-XBPM-212:SA:SA_Y_MONITOR", "FE-DI-XBPM-232:SA:SA_X_MONITOR", "FE-DI-XBPM-232:SA:SA_Y_MONITOR", "FE-DI-XBPM-252:SA:SA_X_MONITOR", "FE-DI-XBPM-252:SA:SA_Y_MONITOR", "FE-DI-XBPM-412:SA:SA_X_MONITOR", "FE-DI-XBPM-412:SA:SA_Y_MONITOR", "FE-DI-XBPM-452:SA:SA_X_MONITOR", "FE-DI-XBPM-452:SA:SA_Y_MONITOR"] ("appended array")) -> ("1rst Value (number)"=w398:dbl[])  [unwired: 8 in, 6 out]
    n166 = Multiply(x=w398, y=0.001) -> (x*y=w397:dbl[])
    n167 = disable-structure shown="Disabled" {
      frame Disabled {
        n168 = To Long Integer() -> (32bit integer=w861:i32)  [unwired: 1 in]
        n169 = case shown="1" w861 {
          tunnel: ["Decay" "Top-Up"] -> _
          frame 0, Default {
          }
          frame 1 {
          }
        }
      }
      frame Enabled {
      }
    }
    n170 = call-poly <userlib>:"CaLabGet.vi"("PV Names"=string[] ["SR-DI-FP:CurrentBuffer", "BR-DI-FP:CurrentBuffer"]) -> ("Value Array (number)"=w468:dbl[][])  [unwired: 8 in, 6 out]
    n171 = Index Array(array=w468, index (row) #1=0 ("index"), index (row) #2=1 ("index (row)")) -> (element #1=w116:dbl[], element #2=w107:dbl[])  [unwired: 2 in]
    n172 = Index Array(array=w397, index #1=0 ("index"), index #2=1 ("index"), index #3=2 ("index"), index #4=3 ("index"), index #5=4 ("index"), index #6=5 ("index"), index #7=6 ("index"), index #8=7 ("index"), index #9=8 ("index"), index #10=9 ("index"), index #11=10 ("index"), index #12=11 ("index"), index #13=12 ("index"), index #14=13 ("index"), index #15=14 ("index"), index #16=15 ("index"), index #17=16 ("index"), index #18=17 ("index"), index #19=18 ("index"), index #20=19 ("index"), index #21=20 ("index"), index #22=21 ("index"), index #23=22 ("index"), index #24=23 ("index"), index #25=24 ("index"), index #26=25 ("index"), index #27=26 ("index"), index #28=27 ("index")) -> (element #1=w316:dbl, element #2=w309:dbl, element #3=w315:dbl, element #4=w308:dbl, element #5=w314:dbl, element #6=w307:dbl, element #7=w313:dbl, element #8=w306:dbl, element #9=w312:dbl, element #10=w305:dbl, element #11=w311:dbl, element #12=w304:dbl, element #13=w310:dbl, element #14=w303:dbl, element #15=w210:dbl, element #16=w209:dbl, element #17=w208:dbl, element #18=w207:dbl, element #19=w198:dbl, element #20=w197:dbl, element #21=w192:dbl, element #22=w191:dbl, element #23=w190:dbl, element #24=w189:dbl, element #25=w158:dbl, element #26=w157:dbl, element #27=w156:dbl, element #28=w155:dbl)
    n173 = Build Array (concatenate)(w116, w116) -> (w114:dbl[])
    n174 = for {
      tunnel: w114 -> [w576] mode=indexing
      shift-right: [w570] -> _
      shift-left: _ -> [w569]
      shift-right: [w573] -> _
      shift-left: 0 -> [w574]
      tunnel: [w571] -> w118 mode=indexing if=w564
      w575 = 0.05  # Threshold
      n175 = Increment(x=w574) -> (x+1=w571:i32)
      n176 = Less Or Equal?(x=w576, y=w575) -> (x <= y?=w570:bool)
      n177 = Not Equal?(x=w570, y=w569) -> ()  [unwired: 1 out]
      n178 = Equal?(x=w570, y=TRUE) -> (x = y?=w561:bool)
      n179 = Equal?(x=w569, y=FALSE) -> (x = y?=w560:bool)
      n180 = Equal?(x=w570, y=FALSE) -> (x = y?=w566:bool)
      n181 = Equal?(x=w569, y=TRUE) -> (x = y?=w565:bool)
      n182 = And(x=w561, y=w560) -> (x .and. y?=w559:bool)
      n183 = And(x=w566, y=w565) -> (x .and. y?=w564:bool)
      n184 = Select(t=0, s=w559, f=w571) -> (s? t:f=w573:i32)
    }
    n185 = Array Max & Min(array=w118) -> (max value=w119:i32)  [unwired: 3 out]
    n186 = Multiply(x=w119, y=2) -> (x*y=w115:i32)
    n187 = Add Array Elements(numeric array=w107) -> (sum=w110:dbl)
    n188 = call-poly <userlib>:"CaLabGet.vi"("PV Names"=string[] ["LI-ES-CPS-01:PULSEMODE", "LI-ES-BPS-01:SETU:GRID", "LI-ES-BPS-01:SETU:MBM", "LI-ES-BPS-01:SETU:SBM", "LI-RF-HVP-31:SET:U", "CPCITM-TI-EVRTG:Pulse6DelaySet", "CPCITM-TI-EVRTG:Pulse7DelaySet", "CPCITM-TI-EVRTG:Pulse6WidthSet", "CPCITM-TI-EVRTG:Pulse7WidthSet", "CPCITM-TI-EVRTG:GTX6CtrlGTXPHSet", "CPCITM-TI-EVRTG:GTX7CtrlGTXPHSet", "CPCITM-TI-EVRTG:GTX6DlySet", "CPCITM-TI-EVRTG:GTX7DlySet"]) -> ("1rst Value (string)"=w460:string[], "1rst Value (number)"=w511:dbl[])  [unwired: 8 in, 5 out]
    n189 = call-poly <userlib>:"CaLabGet.vi"("PV Names"=string[] ["BR-PS-INJ-SE:setHV", "BR-PS-INJ-KI:setHV", "BR-PS-EXT-K1:setHV", "BR-PS-EXT-K2:setHV", "BR-PS-EXT-SE1:setHV", "BR-PS-EXT-SE2:setHV", "SR-PS-INJ-SE1:setHV", "SR-PS-INJ-SE2:setHV", "SR-PS-INJ-K1:setHV", "SR-PS-INJ-K2:setHV", "SR-PS-INJ-K3:setHV", "SR-PS-INJ-K4:setHV"]) -> ("1rst Value (number)"=w513:dbl[])  [unwired: 8 in, 6 out]
    n190 = call-poly <userlib>:"CaLabGet.vi"("PV Names"=string[] ["SR-RF-MSG:setFreq", "SR-RF2-LLRF:local", "SR-RF2-LLRF:getOperationMode", "SR-RF2-LLRF:getGapVoltage", "SR-RF2-LLRF:setGapVoltage", "SR-RF2-LLRF:setStationPhase", "SR-RF3-LLRF:local", "SR-RF3-LLRF:getOperationMode", "SR-RF3-LLRF:getGapVoltage", "SR-RF3-LLRF:setGapVoltage", "SR-RF3-LLRF:setStationPhase"]) -> ("1rst Value (number)"=w486:dbl[])  [unwired: 8 in, 6 out]
    n191 = Greater Or Equal?(x=w110, y=0.05) -> (x >= y?=w108:bool)
    n192 = call-poly <userlib>:"CaLabGet.vi"("PV Names"=string[] ["TI-INJ-PROC:TopupHiLowStart", "SR-DI-DCCT:BeamCurrent", "SR-DI-DCCT:BeamLifetime", "SR-DI-XPC-40:SigmaX", "SR-DI-XPC-40:SigmaY", "SR-DI-TUNE:nux", "SR-DI-TUNE:nuy", "IGPF:TPSX:SRAM:VEC:PEAKFREQ2", "IGPF:TPSY:SRAM:VEC:PEAKFREQ2", "TI-INJ-PROC:setBucketAddressStart", "TI-INJ-PROC:setBucketAddressLast", "TI-INJ-PROC:setBucketAddressStep"]) -> ("1rst Value (number)"=w547:dbl[])  [unwired: 8 in, 6 out]
    n193 = call-poly <userlib>:"CaLabGet.vi"("PV Names"=string[] ["LI:restoreFilename", "LTB:restoreFilename", "BR:restoreFilename", "BTS:restoreFilename", "SR:restoreFilename"]) -> ("1rst Value (string)"=w470:string[])  [unwired: 8 in, 6 out]
    n194 = Index Array(array=w460, index=0) -> (element=w458:string)
    n195 = Index Array(array=w511, index #1=0 ("index"), index #2=1 ("index"), index #3=2 ("index"), index #4=3 ("index"), index #5=4 ("index"), index #6=5 ("index"), index #7=6 ("index"), index #8=7 ("index"), index #9=8 ("index"), index #10=9 ("index"), index #11=10 ("index"), index #12=11 ("index"), index #13=12 ("index")) -> (element #2=w348:dbl, element #3=w462:dbl, element #4=w461:dbl, element #5=w346:dbl, element #8=w457:dbl, element #9=w456:dbl, element #10=w455:dbl, element #11=w454:dbl, element #12=w453:dbl, element #13=w452:dbl)  [unwired: 3 out]
    n196 = Index Array(array=w513, index #1=0 ("index"), index #2=1 ("index"), index #3=2 ("index"), index #4=3 ("index"), index #5=4 ("index"), index #6=5 ("index"), index #7=6 ("index"), index #8=7 ("index"), index #9=8 ("index"), index #10=9 ("index"), index #11=10 ("index"), index #12=11 ("index")) -> (element #1=w361:dbl, element #2=w360:dbl, element #3=w359:dbl, element #4=w358:dbl, element #5=w357:dbl, element #6=w356:dbl, element #7=w355:dbl, element #8=w354:dbl, element #9=w353:dbl, element #10=w352:dbl, element #11=w351:dbl, element #12=w350:dbl)
    n197 = Index Array(array=w486, index #1=0 ("index"), index #2=1 ("index"), index #3=2 ("index"), index #4=3 ("index"), index #5=4 ("index"), index #6=5 ("index"), index #7=6 ("index"), index #8=7 ("index"), index #9=8 ("index"), index #10=9 ("index"), index #11=10 ("index")) -> (element #1=w340:dbl, element #2=w483:dbl, element #3=w481:dbl, element #5=w264:dbl, element #6=w265:dbl, element #7=w478:dbl, element #8=w477:dbl, element #10=w336:dbl, element #11=w337:dbl)  [unwired: 2 out]
    n198 = Index Array(array=w547, index #1=0 ("index"), index #2=1 ("index"), index #3=2 ("index"), index #4=3 ("index"), index #5=4 ("index"), index #6=5 ("index"), index #7=6 ("index"), index #8=7 ("index"), index #9=8 ("index"), index #10=9 ("index"), index #11=10 ("index"), index #12=11 ("index")) -> (element #1=w545:dbl, element #2=w87:dbl, element #3=w369:dbl, element #4=w533:dbl, element #5=w531:dbl, element #6=w530:dbl, element #7=w529:dbl, element #8=w528:dbl, element #9=w526:dbl, element #10=w364:dbl, element #11=w363:dbl, element #12=w362:dbl)
    n199 = call-poly <userlib>:"CaLabGet.vi"("PV Names"=w240) -> ("1rst Value (number)"=w242:dbl[])  [unwired: 8 in, 6 out]
    n200 = Index Array(array=w470, index #1=0 ("index"), index #2=1 ("index"), index #3=2 ("index"), index #4=3 ("index"), index #5=4 ("index")) -> (element #1=w332:string, element #2=w331:string, element #3=w335:string, element #4=w334:string, element #5=w333:string)
    n201 = call-poly <userlib>:"CaLabGet.vi"("PV Names"=w431) -> ("1rst Value (string)"=w439:string[])  [unwired: 8 in, 6 out]
    n202 = To Byte Integer(number=w242) -> (8bit integer=w241:i8[])
    n203 = feedback #1() -> (w103:string)  [unwired: 1 in]
    n204 = case shown="True" w108 {
      tunnel: w107 -> [_ w558]
      tunnel: [w556 w558] -> w105
      tunnel: w106 -> [w556 _]
      tunnel: [w555 w557] -> w104
      tunnel: w103 -> [w555 _]
      frame False {
      }
      frame True {
        n205 = local read "NOW time"() -> (w557:string)
      }
    }
    n206 = feedback-in #1(w104) -> ()
    n207 = for {
      tunnel: w241 -> [w820] mode=indexing
      tunnel: [w817] -> w218 mode=indexing
      n208 = Number To Boolean Array(number=w820) -> (Boolean array=w819:bool[])
      n209 = Index Array(array=w819, index=0) -> (element=w817:bool)
    }
    n210 = for {
      tunnel: w439 -> [w830] mode=indexing
      tunnel: [w829] -> w440 mode=indexing
      n211 = case shown="\"Enable\"" w830 {
        tunnel: [FALSE TRUE] -> w829
        frame "Disable", Default {
        }
        frame "Enable" {
        }
      }
    }
    n212 = call-poly <userlib>:"CaLabGet.vi"("PV Names"=w450) -> ("1rst Value (string)"=w442:string[])  [unwired: 8 in, 6 out]
    n213 = call-poly <userlib>:"CaLabGet.vi"("PV Names"=string[] ["SR-ID-IU22-05:getGap", "SR-ID-IU22A-09:getGap", "SR-ID-IU22B-09:getGap", "SR-ID-IUT22-21:getGap", "SR-ID-IU22-23:getGap", "SR-ID-IU22A-25:getGap", "SR-ID-IU22B-25:getGap", "SR-ID-EPU48A-41:getGap", "SR-ID-EPU48A-41:getPhase", "SR-ID-EPU48B-41:getGap", "SR-ID-EPU48B-41:getPhase", "SR-ID-EPU46-45:getGap", "SR-ID-EPU46-45:getPhase", "SR-ID-IUT22-21:getGapTaper", "SR-ID-EPU48PS-41:getGap"]) -> ("1rst Value (number)"=w430:dbl[])  [unwired: 8 in, 6 out]
    n214 = for {
      tunnel: w442 -> [w834] mode=indexing
      tunnel: [w833] -> w441 mode=indexing
      n215 = case shown="\"enable\"" w834 {
        tunnel: [FALSE TRUE] -> w833
        frame "disable", Default {
        }
        frame "enable" {
        }
      }
    }
    n216 = call-poly <userlib>:"CaLabGet.vi"("PV Names"=string[] ["SR-ID-IU22-05:gapMotorOff", "SR-ID-IU22A-09:gapMotorOff", "SR-ID-IU22B-09:gapMotorOff", "SR-ID-IUT22-21:gapMotorOff", "SR-ID-IU22-23:gapMotorOff", "SR-ID-IU22A-25:gapMotorOff", "SR-ID-IU22B-25:gapMotorOff", "SR-ID-EPU48A-41:gapMotorOff", "SR-ID-EPU48B-41:gapMotorOff", "SR-ID-EPU46-45:gapMotorOff", "SR-ID-EPU48A-41:phaseMotorOff", "SR-ID-EPU48B-41:phaseMotorOff", "SR-ID-EPU46-45:phaseMotorOff"]) -> ("1rst Value (string)"=w382:string[])  [unwired: 8 in, 6 out]
    n217 = To Long Integer(number=w481) -> (32bit integer=w482:i32)
    n218 = To Long Integer(number=w483) -> (32bit integer=w484:i32)
    n219 = To Long Integer(number=w477) -> (32bit integer=w480:i32)
    n220 = To Long Integer(number=w478) -> (32bit integer=w479:i32)
    n221 = Index Array(array=w430, index #1=0 ("index"), index #2=1 ("index"), index #3=2 ("index"), index #4=3 ("index"), index #5=4 ("index"), index #6=5 ("index"), index #7=6 ("index"), index #8=7 ("index"), index #9=8 ("index"), index #10=9 ("index"), index #11=10 ("index"), index #12=11 ("index"), index #13=12 ("index"), index #14=13 ("index"), index #15=14 ("index")) -> (element #1=w330:dbl, element #2=w329:dbl, element #3=w328:dbl, element #4=w327:dbl, element #5=w326:dbl, element #6=w325:dbl, element #7=w324:dbl, element #8=w323:dbl, element #9=w322:dbl, element #10=w321:dbl, element #11=w320:dbl, element #12=w319:dbl, element #13=w318:dbl, element #14=w263:dbl, element #15=w317:dbl)
    n222 = for {
      tunnel: w382 -> [w826] mode=indexing
      tunnel: [w825] -> w381 mode=indexing
      n223 = case shown="\"1\", Default" w826 {
        tunnel: [FALSE TRUE] -> w825
        frame "1", Default {
        }
        frame "0" {
        }
      }
    }
    n224 = Index Array(array=w218, index #1=0 ("index"), index #2=1 ("index"), index #3=2 ("index"), index #4=3 ("index"), index #5=4 ("index"), index #6=5 ("index"), index #7=6 ("index"), index #8=7 ("index"), index #9=8 ("index"), index #10=9 ("index"), index #11=10 ("index"), index #12=11 ("index"), index #13=12 ("index"), index #14=13 ("index"), index #15=14 ("index"), index #16=15 ("index"), index #17=16 ("index"), index #18=17 ("index"), index #19=18 ("index"), index #20=19 ("index"), index #21=20 ("index")) -> (element #1=w215:bool, element #2=w214:bool, element #3=w213:bool, element #4=w202:bool, element #5=w201:bool, element #6=w200:bool, element #7=w195:bool, element #8=w194:bool, element #9=w193:bool, element #10=w184:bool, element #11=w183:bool, element #12=w182:bool, element #13=w177:bool, element #14=w176:bool, element #15=w175:bool, element #16=w174:bool, element #17=w173:bool, element #18=w172:bool, element #19=w171:bool, element #20=w170:bool, element #21=w169:bool)
    n225 = case shown="1" w484 {
      tunnel: [FALSE TRUE] -> w342
      frame 0, Default {
      }
      frame 1 {
      }
    }
    n226 = case shown="1" w479 {
      tunnel: [FALSE TRUE] -> w339
      frame 0, Default {
      }
      frame 1 {
      }
    }
    n227 = case shown="0" w482 {
      tunnel: [TRUE FALSE] -> w341
      frame 0 {
      }
      frame 1, Default {
      }
    }
    n228 = case shown="0" w480 {
      tunnel: [TRUE FALSE] -> w338
      frame 0 {
      }
      frame 1, Default {
      }
    }
    n229 = To Long Integer(number=w545) -> (32bit integer=w548:i32)
    n230 = Negate(x=w263) -> (-x=w262:dbl)
    n231 = case shown="1" w548 {
      tunnel: ["Decay" "Top-Up"] -> w370
      frame 0, Default {
      }
      frame 1 {
      }
    }
    n232 = Index Array(array=w440, index #1=0 ("index"), index #2=1 ("index"), index #3=2 ("index"), index #4=3 ("index"), index #5=4 ("index"), index #6=5 ("index"), index #7=6 ("index")) -> (element #1=w216:bool, element #2=w212:bool, element #3=w196:bool, element #4=w179:bool, element #5=w178:bool, element #6=w160:bool, element #7=w159:bool)
    n233 = case shown="\"MBM\", Default" w458 {
      tunnel: ["MBM" "SBM"] -> w349
      tunnel: w462 -> [w840 _]
      tunnel: [w840 w845] -> w347
      tunnel: w461 -> [_ w845]
      tunnel: w457 -> [_ w844]
      tunnel: w456 -> [w839 _]
      tunnel: [w839 w844] -> w345
      tunnel: w455 -> [_ w843]
      tunnel: w454 -> [w838 _]
      tunnel: [w838 w843] -> w344
      tunnel: w453 -> [_ w842]
      tunnel: w452 -> [w837 _]
      tunnel: [w837 w842] -> w343
      frame "MBM", Default {
      }
      frame "SBM" {
      }
    }
    n234 = Multiply(x=w533, y=w532) -> (x*y=w368:dbl)
    n235 = Divide(x=w528, y=w527) -> (x/y=w366:dbl)
    n236 = Multiply(x=w531, y=w532) -> (x*y=w367:dbl)
    n237 = Divide(x=w526, y=w527) -> (x/y=w365:dbl)
    n238 = Index Array(array=w441, index #1=0 ("index"), index #2=1 ("index"), index #3=2 ("index"), index #4=3 ("index"), index #5=4 ("index"), index #6=5 ("index"), index #7=6 ("index")) -> (element #1=w217:bool, element #2=w211:bool, element #3=w199:bool, element #4=w181:bool, element #5=w180:bool, element #6=w162:bool, element #7=w161:bool)
    n239 = call "FE_PAB_OpenState.vi"("FE"=w217, "XBPMX 2"=w210, "XBPMY 2"=w209, "Hutch"=w216, "PAB"=w215, "MGV"=w214, "FCV"=w213) -> ("XBPMX 2"=w206:string, "XBPMY 2"=w205:string)  [unwired: 7 in]
    n240 = call "FE_PAB_OpenState.vi"("FE"=w211, "XBPMX 2"=w208, "XBPMY 2"=w207, "Hutch"=w212, "PAB"=w202, "MGV"=w201, "FCV"=w200) -> ("XBPMX 2"=w204:string, "XBPMY 2"=w203:string)  [unwired: 7 in]
    n241 = call-poly <userlib>:"CaLabGet.vi"("PV Name"="TI-INJ-PROC:getTrig-SR-KICKER") -> ("1rst Value (string)"=w465:string)  [unwired: 8 in, 6 out]
    n242 = Index Array(array=w381, index #1=0 ("index"), index #2=1 ("index"), index #3=2 ("index"), index #4=3 ("index"), index #5=4 ("index"), index #6=5 ("index"), index #7=6 ("index"), index #8=7 ("index"), index #9=8 ("index"), index #10=9 ("index"), index #11=10 ("index"), index #12=11 ("index"), index #13=12 ("index")) -> (element #1=w302:bool, element #2=w301:bool, element #3=w300:bool, element #4=w299:bool, element #5=w298:bool, element #6=w297:bool, element #7=w296:bool, element #8=w295:bool, element #9=w294:bool, element #10=w293:bool, element #11=w292:bool, element #12=w291:bool, element #13=w290:bool)
    n243 = call-poly <userlib>:"CaLabGet.vi"("PV Names"=w372) -> ("1rst Value (number)"=w374:dbl[])  [unwired: 8 in, 6 out]
    n244 = call-poly <userlib>:"CaLabGet.vi"("PV Names"=w373) -> ("1rst Value (number)"=w376:dbl[])  [unwired: 8 in, 6 out]
    n245 = call "FE_PAB_OpenState.vi"("FE"=w199, "XBPMX 2"=w198, "XBPMY 2"=w197, "Hutch"=w196, "PAB"=w195, "MGV"=w194, "FCV"=w193) -> ("XBPMX 2"=w188:string, "XBPMY 2"=w187:string)  [unwired: 7 in]
    n246 = call-poly <userlib>:"CaLabGet.vi"("PV Names"=string[] ["SR-DI-FOFB-H:getStatus", "SR-DI-FOFB-V:getStatus", "IGPF:TPSX:FBCTRL", "IGPF:TPSY:FBCTRL", "TPS-SR-022:bpm3:ilk:enabled", "SR-DI-ANGLE-ILK:StatusX", "SR-DI-ANGLE-ILK:StatusY", "SR-DI-RF-FB:getStatus"]) -> ("1rst Value (string)"=w278:string[], "1rst Value (number)"=w279:dbl[])  [unwired: 8 in, 5 out]
    n247 = Get Date/Time In Seconds() -> (seconds since 1Jan1904=w89:timestamp)
    n248 = call "FE_PAB_OpenState.vi"("FE"=w181, "XBPMX 2"=w192, "XBPMY 2"=w191, "Hutch"=w179, "PAB"=w184, "MGV"=w183, "FCV"=w182) -> ("XBPMX 2"=w186:string, "XBPMY 2"=w185:string)  [unwired: 7 in]
    n249 = Multiply(x=w374, y=w375) -> (x*y=w98:dbl[])
    n250 = To Byte Integer(number=w279) -> (8bit integer=w275:i8[])
    n251 = Multiply(x=w376, y=w375) -> (x*y=w97:dbl[])
    n252 = for {
      tunnel: w275 -> [w822] mode=indexing
      tunnel: [w821] -> w285 mode=indexing
      n253 = case shown="1" w822 {
        tunnel: [TRUE FALSE] -> w821
        frame 1 {
        }
        frame 0, Default {
        }
      }
    }
    n254 = Subtract(x=w88, y=w87) -> (x-y=w94:dbl)
    n255 = Array Max & Min(array=w98) -> (max value=w102:dbl, min value=w101:dbl)  [unwired: 2 out]
    n256 = Array Max & Min(array=w97) -> (max value=w100:dbl, min value=w99:dbl)  [unwired: 2 out]
    n257 = Format Date/Time String(time format string (%c)="%Y%m%d_%H%M%S", seconds (now)=w89) -> (date/time string=w90:string)  [unwired: 1 in]
    n258 = Greater?(x=w94, y=150.0) -> (0:w92:bool)
    n259 = call "FE_PAB_OpenState.vi"("FE"=w180, "XBPMX 2"=w190, "XBPMY 2"=w189, "Hutch"=w178, "PAB"=w177, "MGV"=w176, "FCV"=w175) -> ("XBPMX 2"=w168:string, "XBPMY 2"=w167:string)  [unwired: 7 in]
    n260 = Index Array(array=w278, index #1=0 ("index"), index #2=1 ("index"), index #3=7 ("index")) -> (element #1=w273:string, element #2=w272:string, element #3=w125:string)
    n261 = case shown="True" w92 {
      tunnel: w90 -> [_ w550]
      frame False {
      }
      frame True {
        n262 = flat-sequence {
          tunnel: [w552] -> w551
          tunnel: w550 -> [w552]
          tunnel: w551 -> [w554]
          frame #0 {
            n263 = Wait Until Next ms Multiple(millisecond multiple=u32 30000) -> ()  [unwired: 1 out]
          }
          frame #1 {
            n264 = call "Save_PM_BPM_data.vi"("date_time"=w554) -> ()  [unwired: 11 in]
          }
        }
      }
    }
    n265 = property on="BPMY Graph 2" class="XYGraph (strict)"("YScale.Maximum"=w100, "YScale.Minimum"=w99) -> ()  [unwired: 2 in, 2 out]
    n266 = property on="BPMX Graph 2" class="XYGraph (strict)"("YScale.Maximum"=w102, "YScale.Minimum"=w101) -> ()  [unwired: 2 in, 2 out]
    n267 = call "FE_PAB_OpenState.vi"("FE"=w162, "XBPMX 2"=w158, "XBPMY 2"=w157, "Hutch"=w160, "PAB"=w174, "MGV"=w173, "FCV"=w172) -> ("XBPMX 2"=w166:string, "XBPMY 2"=w165:string)  [unwired: 7 in]
    n268 = call "FE_PAB_OpenState.vi"("FE"=w161, "XBPMX 2"=w156, "XBPMY 2"=w155, "Hutch"=w159, "PAB"=w171, "MGV"=w170, "FCV"=w169) -> ("XBPMX 2"=w164:string, "XBPMY 2"=w163:string)  [unwired: 7 in]
    n269 = Bundle("Array of X axis  平均分配至各段"=w123, w98) -> (w122:cluster{"Array of X axis  平均分配至各段":dbl[], dbl[]})  [unwired: 1 in]
    n270 = Bundle("Array of X axis  平均分配至各段"=w123, w97) -> (w121:cluster{"Array of X axis  平均分配至各段":dbl[], dbl[]})  [unwired: 1 in]
    n271 = Index Array(array=w285, index #1=2 ("index"), index #2=3 ("index"), index #3=4 ("index"), index #4=5 ("index"), index #5=6 ("index")) -> (element #1=w271:bool, element #2=w270:bool, element #3=w269:bool)  [unwired: 2 out]
    n272 = Equal?(x="1" ("1rst Value (string)"), y=w465) -> (x = y?=w463:bool)
    "x = y?" <- w463
    n273 = case shown="True" TRUE {
      tunnel: w130 -> [_ w577]
      frame False {
      }
      frame True {
        n274 = Quit LabVIEW(quit? (T)=w577) -> ()
      }
    }
    n275 = case shown="True" w463 {
      tunnel: w530 -> [_ w850]
      tunnel: w529 -> [_ w849]
      tunnel: [w848 w850] -> w261
      tunnel: [w847 w849] -> w260
      tunnel: w259 -> [w848 _]
      tunnel: w258 -> [w847 _]
      frame False {
      }
      frame True {
        n276 = local read "NOW date"() -> (→"date kickeron":string)
        n277 = local read "NOW time"() -> (→"time kickeron":string)
      }
    }
    n278 = Wait Until Next ms Multiple(millisecond multiple=u32 630) -> ()  [unwired: 1 out]
    n279 = local read "date kickeron"() -> (w267:string)
    n280 = local read "time kickeron"() -> (w266:string)
    n281 = Get Date/Time In Seconds() -> (seconds since 1Jan1904=w378:timestamp)
    n282 = call-poly <userlib>:"CaLabGet.vi"("PV Names"=w154) -> ("1rst Value (string)"=w143:string[])  [unwired: 8 in, 6 out]
    n283 = Format Date/Time String(time format string (%c)="%Y/%m/%d", seconds (now)=w378) -> (date/time string=→"NOW date":string)  [unwired: 1 in]
    n284 = Format Date/Time String(time format string (%c)="%Y/%m/%d", seconds (now)=w378) -> (date/time string=w289:string)  [unwired: 1 in]
    n285 = Format Date/Time String(time format string (%c)="%H:%M:%S", seconds (now)=w378) -> (date/time string=w288:string)  [unwired: 1 in]
    "NOW time" <- w288
    n286 = Index Array(array=w143, index #1=0 ("index"), index #2=1 ("index"), index #3=2 ("index"), index #4=3 ("index"), index #5=4 ("index"), index #6=5 ("index"), index #7=6 ("index"), index #8=7 ("index"), index #9=8 ("index"), index #10=9 ("index")) -> (element #1=w142:string, element #2=w141:string, element #3=w140:string, element #4=w139:string, element #5=w138:string, element #6=w137:string, element #7=w136:string, element #8=w135:string, element #9=w134:string, element #10=w133:string)
    n287 = Bundle By Name(cluster=T1 {"SR Fill Pattern"=[], "Beam Current(mA"=320.769453, "Beam Lifetime(min)"=354.3939151043138, "Beamsize X(um)"=63.15189373514937, "Beamsize Y(um)"=38.03691397287648, "Tune X(from BPM)"=0.1487279843444227, "Tune Y(from BPM)"=0.2309197651663405, "Mode"="Top-Up", "NuX(from BBF) "=0.15142063757609414, "NuY(from BBF)"=0.22496346361412184, "IU22-23gap(R)"=7.0, "IU22-05gap(R)"=7.372, "IU22-05M"=TRUE, "IU22A-09gap(R)"=8.05, "IU22A-09M"=TRUE, "IU22B-09gap(R)"=40.001, "IU22B-09M"=FALSE, "IUT22-21gap(R)"=7.0, "IUT22-21M"=TRUE, "IU22-23M"=TRUE, "IU22A-25gap(R)"=7.0, "IU22A-25M"=TRUE, "IU22B-25gap(R)"=40.0, "IU22B-25M"=FALSE, "EPU48A-41gap(R)"=65.00055, "EPU48A-41gM"=FALSE, "EPU48B-41gap(R)"=27.450000000000003, "EPU48B-41gM"=TRUE, "EPU46-45gap(R)"=44.99850000000001, "EPU46-45gM"=FALSE, "EPU48A-41phase(R)"=0.00055, "EPU48B-41phase(R)"=0.0, "EPU46-45phase(R)"=5e-05, "Grid volt.(V)[S]"=33.0, "Gun mode"="MBM", "Mod.3 HV(kV)[S]"=35.37999999999996, "SR"="SR_DMB_2017_1024_0300LOCO.data", "BR"="Booster_2017_1023_0900.data", "LI"="Linac_2017_0413_1015.data", "LTB"="LTB_JT_2017_0828_1050.data", "BTS"="BTS_2017_1023_0900.data", "RF2 remote"=TRUE, "RF2 OP mode"=TRUE, "RF2 phase.[S]"=-42.0, "RF Freq.(s)"=499655365.67399085, "RF2 gap volt[S]"=1600.0, "RF3 remote"=TRUE, "RF3 OP mode"=TRUE, "RF3 phase.[S]"=1.1999999999999995, "RF3 gap volt.[S]"=1600.0, "BBF V"=TRUE, "BBF H"=TRUE, "BR ext. kicker1(kV)"=17.666, "BR ext. kicker2(kV)"=17.666, "BR ext. sep.1(V)"=322.14, "BR ext. sep.2(V)"=441.1, "BR inj. sep.(V)"=104.95, "BR inj. kicker(kV)"=13.449999999999969, "SR kicker4(kV)"=7.945, "SR kicker3(kV)"=8.02, "SR kicker2(kV)"=8.142, "SR kicker1(kV)"=8.1, "SR inj. sep.2(V)"=397.2, "SR inj. sep.1(V)"=398.04, "Bucket Start"=100.0, "Bucket Last"=450.0, "Bucket Step"=10.0, "Orbit ILK(P)"=TRUE, "IU22-05 Hutch Enable"=TRUE, "IU22A-09M Hutch Enable"=TRUE, "IUT22-21M Hutch Enable"=TRUE, "IU22-23M Hutch Enable"=TRUE, "IU22A-25M Hutch Enable"=TRUE, "EPU48A-41M Hutch Enable"=TRUE, "EPU46-45M Hutch Enable"=FALSE, "EPU46-45 FE Enable"=TRUE, "EPU48A-41 FE Enable"=TRUE, "IU22A-25 FE Enable"=TRUE, "IU22-23 FE Enable"=TRUE, "IUT22-21 FE Enable"=TRUE, "IU22A-09 FE Enable"=TRUE, "IU22-05 FE Enable"=TRUE, "EPU48A-41pM"=FALSE, "EPU48B-41pM"=TRUE, "EPU46-45pM"=FALSE, "Gun volt.(V)[S]"=23.5, "Width count"=75.0, "2ns step"=2.0, "10ps delay"=150.0, "phase shifter"=130.0015, "Taper"=1.0899999999999999, "05XBPMX 1"=14.279, "09XBPMX 1"=-34.837, "21XBPMX 1"=-36.466, "23XBPMX 1"=-38.547000000000004, "25XBPMX 1"=-40.08, "41XBPMX 1"=-513.551, "45XBPMX 1"=-12.86, "05XBPMY 1"=51.999, "09XBPMY 1"=30.004, "21XBPMY 1"=-4.771, "23XBPMY 1"=19.080000000000002, "25XBPMY 1"=-4.366, "41XBPMY 1"=309.241, "45XBPMY 1"=1.842, "FOFB H"="On", "FOFB V"="On", "time string"="15:45:09", "date"="2017/10/28", "date (last kicker ON)"="", "time string (last kicker ON)"="", "Radio Buttons 2"=enum."absolute", "09XBPMX 2"="23.77", "09XBPMY 2"="-18.01", "05XBPMY 2"="-459.85", "05XBPMX 2"="-403.56", "21XBPMY 2"="-134.87", "21XBPMX 2"="-31.92", "23XBPMY 2"="233.82", "23XBPMX 2"="11.09", "25XBPMY 2"="5171.53", "25XBPMX 2"="2152.43", "41XBPMY 2"=" closed", "41XBPMX 2"=" PAB ", "45XBPMX 2"=" Hutch ", "45XBPMY 2"=" closed", "05 mode"="Follow", "09A mode"="Follow", "09B mode"="Follow", "21 mode"="Follow", "23 mode"="Follow", "25A mode"="Follow", "25B mode"="Follow", "41A mode"="Follow", "41B mode"="Follow", "46 mode"="Follow", "BeamCurrent History"={"BPM NO.  1_172"=array[4319 elements], array[4319 elements]}, "SR Beam Current in            hours"=12.0, "RF FB"="On", "gap value："=0, "BR Fill Pattern"=[], "time string (last INJ) "="", "BPMX Graph 2"={"Array of X axis  平均分配至各段"=[1.0, 1.1666666666666667, 1.3333333333333333, 1.5, 1.6666666666666665, 1.8333333333333333, 2.0, 2.142857142857143, 2.2857142857142856, 2.4285714285714284, 2.571428571428571, 2.7142857142857144, 2.857142857142857, 3.0, 3.142857142857143, 3.2857142857142856, 3.4285714285714284, 3.571428571428571, 3.7142857142857144, 3.857142857142857, 4.0, 4.125, 4.25, 4.375, 4.5, 4.625, 4.75, 4.875, 5.0, 5.125, 5.25, 5.375, 5.5, 5.625, 5.75, 5.875, 6.0, 6.142857142857143, 6.285714285714286, 6.428571428571429, 6.571428571428571, 6.714285714285714, 6.857142857142857, 7.0, 7.142857142857143, 7.285714285714286, 7.428571428571429, 7.571428571428571, 7.714285714285714, 7.857142857142857, 8.0, 8.142857142857142, 8.285714285714286, 8.428571428571429, 8.571428571428571, 8.714285714285714, 8.857142857142858, 9.0, 9.142857142857142, 9.285714285714286, 9.428571428571429, 9.571428571428571, 9.714285714285714, 9.857142857142858, 10.0, 10.142857142857142, 10.285714285714286, 10.428571428571429, 10.571428571428571, 10.714285714285714, 10.857142857142858, 11.0, 11.142857142857142, 11.285714285714286, 11.428571428571429, 11.571428571428571, 11.714285714285714, 11.857142857142858, 12.0, 12.125, 12.25, 12.375, 12.5, 12.625, 12.75, 12.875, 13.0, 13.125, 13.25, 13.375, 13.5, 13.625, 13.75, 13.875, 14.0, 14.142857142857142, 14.285714285714286, 14.428571428571429, 14.571428571428571, 14.714285714285714, 14.857142857142858, 15.0, 15.142857142857142, 15.285714285714286, 15.428571428571429, 15.571428571428571, 15.714285714285714, 15.857142857142858, 16.0, 16.142857142857142, 16.285714285714285, 16.428571428571427, 16.571428571428573, 16.714285714285715, 16.857142857142858, 17.0, 17.142857142857142, 17.285714285714285, 17.428571428571427, 17.571428571428573, 17.714285714285715, 17.857142857142858, 18.0, 18.142857142857142, 18.285714285714285, 18.428571428571427, 18.571428571428573, 18.714285714285715, 18.857142857142858, 19.0, 19.142857142857142, 19.285714285714285, 19.428571428571427, 19.571428571428573, 19.714285714285715, 19.857142857142858, 20.0, 20.125, 20.25, 20.375, 20.5, 20.625, 20.75, 20.875, 21.0, 21.125, 21.25, 21.375, 21.5, 21.625, 21.75, 21.875, 22.0, 22.142857142857142, 22.285714285714285, 22.428571428571427, 22.571428571428573, 22.714285714285715, 22.857142857142858, 23.0, 23.142857142857142, 23.285714285714285, 23.428571428571427, 23.571428571428573, 23.714285714285715, 23.857142857142858, 24.0, 24.166666666666668, 24.333333333333332, 24.5, 24.666666666666668, 24.833333333333332], [-104.35000000000001, -27.61, -81.269, 31.074, 6.062, -136.0, 99.494, -88.141, -46.889, -165.06900000000002, 6.021, -84.98, 1.75, -8.811, 8.532, -133.949, -96.848, 24.799, 5.059, -100.301, 144.643, -9.353, 21.271, -55.053000000000004, 53.308, 191.175, 158.868, 222.566, -123.501, -26.869, 534.8770000000001, 573.141, -225.076, -6.779, 120.711, -75.419, 85.256, 50.948, -59.4, -203.09900000000002, -20.847, 130.465, -112.508, 76.115, 15.039, -35.207, -105.659, -16.897000000000002, 68.91, -141.159, 107.378, 144.351, -55.053000000000004, -193.076, 129.21, 58.157000000000004, -162.566, 153.643, 28.149, 9.358, -84.211, 85.112, 22.422, -31.252, 89.379, -47.49, 54.793, -68.275, 110.611, -118.584, -371.90500000000003, -20.115000000000002, -329.103, -249.097, -146.817, 118.556, -25.749, -98.32600000000001, 55.269, -122.093, 50.967, -55.89, 88.019, -0.462, -608.1560000000001, -139.752, -304.999, -215.022, 93.23400000000001, 44.699, -65.235, 37.049, -3.491, -169.852, 216.458, 50.398, -92.285, -132.13400000000001, -12.869, 66.74, -188.53300000000002, 148.653, -5.112, -71.334, -177.681, 41.168, -12.532, -184.913, 194.919, 52.414, -75.628, -80.415, -36.814, 105.73100000000001, -104.36800000000001, 110.101, 49.669000000000004, -67.327, -157.372, 29.624000000000002, 22.156, -105.663, 47.799, 11.591000000000001, -75.285, -79.821, 34.331, -24.937, -158.703, 177.15, 200.872, -165.849, -60.67, 20.183, -15.311, -111.206, 107.58800000000001, 26.489, 69.547, -41.230000000000004, 81.986, 54.43, 253.076, 378.43600000000004, -117.003, -304.999, 131.013, 2.21, -158.435, 94.489, 63.017, -82.94500000000001, 99.147, 65.752, -37.261, -102.577, 41.791000000000004, 66.599, -163.73, 160.137, -7.15, -51.275, -140.353, 33.772, 54.203, -147.597, 128.696, 58.22, -47.144, -184.493, 56.980000000000004, 67.437, -54.227000000000004, -0.031]}, "BPMY Graph 2"={"Array of X axis  平均分配至各段"=[1.0, 1.1666666666666667, 1.3333333333333333, 1.5, 1.6666666666666665, 1.8333333333333333, 2.0, 2.142857142857143, 2.2857142857142856, 2.4285714285714284, 2.571428571428571, 2.7142857142857144, 2.857142857142857, 3.0, 3.142857142857143, 3.2857142857142856, 3.4285714285714284, 3.571428571428571, 3.7142857142857144, 3.857142857142857, 4.0, 4.125, 4.25, 4.375, 4.5, 4.625, 4.75, 4.875, 5.0, 5.125, 5.25, 5.375, 5.5, 5.625, 5.75, 5.875, 6.0, 6.142857142857143, 6.285714285714286, 6.428571428571429, 6.571428571428571, 6.714285714285714, 6.857142857142857, 7.0, 7.142857142857143, 7.285714285714286, 7.428571428571429, 7.571428571428571, 7.714285714285714, 7.857142857142857, 8.0, 8.142857142857142, 8.285714285714286, 8.428571428571429, 8.571428571428571, 8.714285714285714, 8.857142857142858, 9.0, 9.142857142857142, 9.285714285714286, 9.428571428571429, 9.571428571428571, 9.714285714285714, 9.857142857142858, 10.0, 10.142857142857142, 10.285714285714286, 10.428571428571429, 10.571428571428571, 10.714285714285714, 10.857142857142858, 11.0, 11.142857142857142, 11.285714285714286, 11.428571428571429, 11.571428571428571, 11.714285714285714, 11.857142857142858, 12.0, 12.125, 12.25, 12.375, 12.5, 12.625, 12.75, 12.875, 13.0, 13.125, 13.25, 13.375, 13.5, 13.625, 13.75, 13.875, 14.0, 14.142857142857142, 14.285714285714286, 14.428571428571429, 14.571428571428571, 14.714285714285714, 14.857142857142858, 15.0, 15.142857142857142, 15.285714285714286, 15.428571428571429, 15.571428571428571, 15.714285714285714, 15.857142857142858, 16.0, 16.142857142857142, 16.285714285714285, 16.428571428571427, 16.571428571428573, 16.714285714285715, 16.857142857142858, 17.0, 17.142857142857142, 17.285714285714285, 17.428571428571427, 17.571428571428573, 17.714285714285715, 17.857142857142858, 18.0, 18.142857142857142, 18.285714285714285, 18.428571428571427, 18.571428571428573, 18.714285714285715, 18.857142857142858, 19.0, 19.142857142857142, 19.285714285714285, 19.428571428571427, 19.571428571428573, 19.714285714285715, 19.857142857142858, 20.0, 20.125, 20.25, 20.375, 20.5, 20.625, 20.75, 20.875, 21.0, 21.125, 21.25, 21.375, 21.5, 21.625, 21.75, 21.875, 22.0, 22.142857142857142, 22.285714285714285, 22.428571428571427, 22.571428571428573, 22.714285714285715, 22.857142857142858, 23.0, 23.142857142857142, 23.285714285714285, 23.428571428571427, 23.571428571428573, 23.714285714285715, 23.857142857142858, 24.0, 24.166666666666668, 24.333333333333332, 24.5, 24.666666666666668, 24.833333333333332], [-143.858, -13.775, -13.785, 122.665, -66.475, 31.541, 2.118, -24.67, 28.275000000000002, 0.139, -36.578, -28.396, 48.925000000000004, 9.287, -3.412, 70.053, -21.479, 14.89, -7.234, 5.521, -3.164, 19.558, -37.538000000000004, 37.11, -77.159, -13.755, 77.63, 28.249000000000002, -209.114, -44.569, 92.851, 173.641, -70.156, -22.722, 17.795, -6.59, 25.654, -41.882, 53.713, 9.237, -26.164, 18.357, 63.695, -8.542, 5.183, -5.99, 9.508000000000001, -5.462, -29.446, 36.574, -52.552, 51.439, -48.502, 0.73, -23.836000000000002, -3.648, -9.628, -5.485, -68.679, 95.486, -62.041000000000004, 54.633, -58.791000000000004, 68.305, -49.682, 29.838, -8.459, 3.213, -5.561, -80.617, 58.144, 15.346, -158.743, -40.726, 5.259, 3.258, 41.128, -54.377, 5.01, 18.84, 11.403, -20.73, 21.792, -17.296, 27.29, 0.783, -6.804, -137.476, 116.70700000000001, -6.929, 17.846, -3.586, 11.754, 6.341, 0.292, -0.911, -8.236, -5.312, 14.939, -29.945, 30.573, -9.991, -49.344, 82.117, -27.45, 22.291, -6.636, -9.389, 10.034, -14.218, 14.215, -7.3, 12.409, -44.302, 50.197, -36.089, -9.120000000000001, 45.881, 14.836, -27.324, 10.765, -10.139, -33.252, 2.737, -9.99, -6.019, -53.329, -28.159, 2.676, -36.9, -2.372, 8.92, 13.599, -25.723, -16.436, 7.722, -0.088, -29.122, 32.814, -20.521, 30.155, -45.734, 36.611000000000004, 74.528, 68.482, -22.548000000000002, -31.398, 134.603, -45.587, -0.981, -40.156, 24.441, 20.477, -31.424, 19.5, -11.789, 16.394000000000002, -38.567, 9.523, 0.09, -0.058, -4.8500000000000005, 11.71, 25.637, -10.51, -18.101, -12.389000000000001, 95.417, -138.726, 30.355, 96.245, -48.666000000000004, 40.851, -0.71]}} ("Cluster"), "Tune X(from BPM)"=w261, "Tune Y(from BPM)"=w260, "date (last kicker ON)"=w267, "time string (last kicker ON)"=w266, "date"=w289, "time string"=w288, "Mode"=w370, "Beam Current(mA"=w87, "Beam Lifetime(min)"=w369, "Beamsize X(um)"=w368, "Beamsize Y(um)"=w367, "NuX(from BBF)"=w366, "NuY(from BBF)"=w365, "Bucket Start"=w364, "Bucket Last"=w363, "Bucket Step"=w362, "BR inj. sep.(V)"=w361, "BR inj. kicker(kV)"=w360, "BR ext. kicker1(kV)"=w359, "BR ext. kicker2(kV)"=w358, "BR ext. sep.1(V)"=w357, "BR ext. sep.2(V)"=w356, "SR inj. sep.1(V)"=w355, "SR inj. sep.2(V)"=w354, "SR kicker1(kV)"=w353, "SR kicker2(kV)"=w352, "SR kicker3(kV)"=w351, "SR kicker4(kV)"=w350, "Gun mode"=w349, "Grid volt.(V)[S]"=w348, "Gun volt.(V)[S]"=w347, "Mod.3 HV(kV)[S]"=w346, "Width count"=w345, "2ns step"=w344, "10ps delay"=w343, "RF2 remote"=w342, "RF2 OP mode"=w341, "RF2 phase.[S]"=w265, "RF Freq.(s)"=w340, "RF2 gap volt[S]"=w264, "RF3 remote"=w339, "RF3 OP mode"=w338, "RF3 phase.[S]"=w337, "RF3 gap volt.[S]"=w336, "BR"=w335, "BTS"=w334, "LI"=w332, "LTB"=w331, "SR"=w333, "SR Fill Pattern"=w116, "IU22-05 Hutch Enable"=w216, "IU22A-09M Hutch Enable"=w212, "IUT22-21M Hutch Enable"=w196, "IU22-23M Hutch Enable"=w179, "IU22A-25M Hutch Enable"=w178, "EPU48A-41M Hutch Enable"=w160, "EPU46-45M Hutch Enable"=w159, "EPU46-45 FE Enable"=w161, "EPU48A-41 FE Enable"=w162, "IU22A-25 FE Enable"=w180, "IU22-23 FE Enable"=w181, "IUT22-21 FE Enable"=w199, "IU22A-09 FE Enable"=w211, "IU22-05 FE Enable"=w217, "IU22-05gap(R)"=w330, "IU22A-09gap(R)"=w329, "IU22B-09gap(R)"=w328, "IUT22-21gap(R)"=w327, "IU22-23gap(R)"=w326, "IU22A-25gap(R)"=w325, "IU22B-25gap(R)"=w324, "EPU48A-41gap(R)"=w323, "EPU48A-41phase(R)"=w322, "EPU48B-41gap(R)"=w321, "EPU48B-41phase(R)"=w320, "EPU46-45gap(R)"=w319, "EPU46-45phase(R)"=w318, "Taper"=w262, "phase shifter"=w317, "05XBPMX 1"=w316, "09XBPMX 1"=w315, "21XBPMX 1"=w314, "23XBPMX 1"=w313, "25XBPMX 1"=w312, "41XBPMX 1"=w311, "45XBPMX 1"=w310, "05XBPMY 1"=w309, "09XBPMY 1"=w308, "21XBPMY 1"=w307, "23XBPMY 1"=w306, "25XBPMY 1"=w305, "41XBPMY 1"=w304, "45XBPMY 1"=w303, "IU22-05M"=w302, "IU22A-09M"=w301, "IU22B-09M"=w300, "IUT22-21M"=w299, "IU22-23M"=w298, "IU22A-25M"=w297, "IU22B-25M"=w296, "EPU48A-41gM"=w295, "EPU48B-41gM"=w294, "EPU46-45gM"=w293, "EPU48A-41pM"=w292, "EPU48B-41pM"=w291, "EPU46-45pM"=w290, "BPMX Graph 2"=w122, "BPMY Graph 2"=w121, "Radio Buttons 2"=enum32{"absolute", "different with"}."absolute", "FOFB H"=w273, "FOFB V"=w272, "BBF H"=w271, "BBF V"=w270, "Orbit ILK(P)"=w269, "05XBPMX 2"=w206, "05XBPMY 2"=w205, "09XBPMX 2"=w204, "09XBPMY 2"=w203, "21XBPMX 2"=w188, "21XBPMY 2"=w187, "23XBPMX 2"=w186, "23XBPMY 2"=w185, "25XBPMX 2"=w168, "25XBPMY 2"=w167, "41XBPMX 2"=w166, "41XBPMY 2"=w165, "45XBPMX 2"=w164, "45XBPMY 2"=w163, "05 mode"=w142, "09A mode"=w141, "09B mode"=w140, "21 mode"=w139, "23 mode"=w138, "25A mode"=w137, "25B mode"=w136, "41A mode"=w135, "41B mode"=w134, "46 mode"=w133, "BeamCurrent History"=w129, "RF FB"=w125, "gap value："=w115, "BR Fill Pattern"=w105, "time string (last INJ)"=w103) -> (→"Cluster":T1)
  }
  n288 = List Folder(path=w19) -> (filenames=w15:string[])  [unwired: 3 in, 3 out]
  n289 = Index Array(array=w15, index=w16) -> (element=w14:string)
  n290 = Build Path(base path=w19, name or relative path=w14) -> (appended path=w13:path)
  "appended path" <- w13
  n291 = while {
    tunnel: w31 -> [_]
    shift-right: [w883] -> _
    shift-left: string[] [] -> [w880]
    shift-right: [w871] -> _
    shift-left: string[][] [] -> [w874]
    tunnel: w39 -> [w877]
    i -> [w875]
    stop <- w876 stop-if-true
    w868 = 1000  # limit
    # "為了使檯面上記憶體不要使用太多而做的筆數限制"
    n292 = flat-sequence {
      tunnel: [w939] -> w884
      tunnel: [w938] -> w881
      tunnel: w880 -> [w938]
      tunnel: [w937] -> w878
      tunnel: w877 -> [w937]
      tunnel: [w949] -> w885
      tunnel: w884 -> [w949]
      tunnel: [w947] -> w882
      tunnel: w881 -> [w948]
      tunnel: [w941] -> w879
      tunnel: w878 -> [w940]
      tunnel: w885 -> [w972]
      tunnel: [w970] -> w883
      tunnel: w882 -> [w970]
      tunnel: w879 -> [w969]
      tunnel: [w969] -> w866
      frame #0 {
        n293 = Tick Count (ms)() -> (millisecond timer value=w939:u32)
      }
      frame #1 {
        n294 = Get Date/Time In Seconds() -> (seconds since 1Jan1904=w944:timestamp)
        n295 = To Double Precision Float(number=w944) -> (double precision float=w943:dbl)
        n296 = Format Date/Time String(time format string (%c)="%Y/%m/%d %H:%M:%S", seconds (now)=w944) -> (date/time string=w945:string)  [unwired: 1 in]
        n297 = Number To Fractional String(number=w943) -> (F-format string=w942:string)  [unwired: 3 in]
        n298 = call-poly <userlib>:"CaLabGet.vi"("PV Names"=w940) -> ("1rst Value (string)"=w947:string[])  [unwired: 8 in, 6 out]
        n299 = for {
          tunnel: w948 -> [w951] mode=indexing
          tunnel: w947 -> [w950] mode=indexing
          tunnel: w940 -> [w959] mode=indexing
          tunnel: w945 -> [w958]
          tunnel: [w957] -> w941 mode=indexing if=w955
          tunnel: w942 -> [w956]
          i -> [w954]
          n300 = Greater Or Equal?(x=w954, y=1) -> (x >= y?=w952:bool)
          n301 = case shown="True" w952 {
            tunnel: w959 -> [_ w968]
            tunnel: w951 -> [_ w967]
            tunnel: w950 -> [_ w966]
            tunnel: w958 -> [_ w965]
            tunnel: [string[] [] w964] -> w957
            tunnel: w956 -> [_ w963]
            tunnel: [FALSE w962] -> w955
            frame False {
            }
            frame True {
              n302 = Not Equal?(x=w967, y=w966) -> (x != y?=w962:bool)
              n303 = Build Array(w965, w968, w967, w966, w963) -> (w964:string[])
            }
          }
        }
      }
      frame #2 {
        n304 = Tick Count (ms)() -> (millisecond timer value=w973:u32)
        n305 = Subtract(x=w973, y=w972) -> (x-y=→"dT":u32)
      }
    }
    n306 = while {
      i -> [w930]
      stop <- w934 stop-if-true
      # "每60秒，表示法:\n100 600"
      # "每十秒，表示法:\n100 100"
      n307 = local read "stop"() -> (w933:bool)
      n308 = Multiply(x="Check period", y=10) -> (x*y=w931:i32)
      n309 = Greater Or Equal?(x=w930, y=w931) -> (x >= y?=w935:bool)
      n310 = Wait Until Next ms Multiple(millisecond multiple=u32 99) -> ()  [unwired: 1 out]
      n311 = Or(x=w935, y=w933) -> (x .or. y?=w934:bool)
    }
    n312 = Array Size(array=w874) -> (size(s)=w873:i32[])
    n313 = Build Array (concatenate)(w874, w866) -> (w870:string[][])
    n314 = Index Array(array=w873, index=0) -> (element=w869:i32)
    "EVENTs" <- w869
    n315 = Greater Or Equal?(x=w869, y=w868) -> (x >= y?=w867:bool)
    n316 = disable-structure shown="Disabled" {
      disable-tunnel: w866 -> [w886 _]
      frame Disabled {
        # "不好，因為會卡住檔案\n有人操作時會造成錯誤。"
        n317 = call "Main_Daily_path.vi"() -> ("Directory path"=w888:path)  [unwired: 10 in, 1 out]
        n318 = Build Path(base path=w888, name or relative path="Association\\changedPVsBKUP.csv" ("string")) -> (appended path=w887:path)
        n319 = call <vilib>:"Check if File or Folder Exists.vi"("path"=w887) -> ("file or folder exists?"=w889:bool, "dup path"=w890:path)  [unwired: 8 in, 1 out]
        n320 = case shown="False" w889 {
          tunnel: w890 -> [w893 w907]
          tunnel: w886 -> [w892 w906]
          frame False {
            w905 = "\n" ("time format string (%c)")
            n321 = Get Date/Time In Seconds() -> (seconds since 1Jan1904=w898:timestamp)
            n322 = Build Array (concatenate)(string[] ["Event Time      ", "PV_name        ", "Ori_Value", "New_Value "] ("diff_Value"), w892) -> (w903:string[][])
            n323 = Format Date/Time String(time format string (%c)="%Y/%m/%d %H:%M:%S", seconds (now)=w898) -> (date/time string=w897:string)  [unwired: 1 in]
            n324 = Array To Spreadsheet String(delimiter (Tab)=",", array=w903, 3:"%s" ("format string")) -> (spreadsheet string=w904:string)
            n325 = Concatenate Strings("#Start Recording Time: " ("time format string (%c)"), w897, w905, "#Note: This file recorded PVs(set values) that were changed \n#(RF frequency was not recorded in this file)\n#Delimiter: ," ("time format string (%c)"), w905, w904, w905) -> (w894:string)
            n326 = Write to Text File(file (use dialog)=w893, text=w894) -> ()  [unwired: 2 in, 3 out]
          }
          frame True {
            n327 = call-poly <vilib>:"Write To Spreadsheet File.vi"("delimiter (\\t)"="," ("delimiter (\\t)"), "transpose? (no:F)"=FALSE, "append to file? (new file:F)"=TRUE, "2D data"=w906, "file path (dialog if empty)"=w907) -> ()  [unwired: 3 in, 1 out]
          }
        }
      }
      frame Enabled {
      }
    }
    n328 = case shown="True" w867 {
      tunnel: w870 -> [w911 w922]
      tunnel: [w911 w926] -> w871
      tunnel: w869 -> [_ w917]
      tunnel: w868 -> [_ w916]
      frame False {
      }
      frame True {
        n329 = call "Main_Daily_path.vi"() -> ("Directory path"=w913:path)  [unwired: 10 in, 1 out]
        n330 = Array Subset(array=w922, index (row)=0 ("index"), length (row)=w916, index (col)=0 ("index"), length (col)=5 ("length")) -> (w921:string[][])
        n331 = Build Path(base path=w913, name or relative path="Association\\changedPVsBKUPov1k.csv" ("string")) -> (appended path=w912:path)
        n332 = Subtract(x=w917, y=w916) -> (x-y=w915:i32)
        n333 = call-poly <vilib>:"Write To Spreadsheet File.vi"("delimiter (\\t)"="," ("delimiter (\\t)"), "transpose? (no:F)"=FALSE, "append to file? (new file:F)"=TRUE, "2D data"=w921, "file path (dialog if empty)"=w912) -> ()  [unwired: 3 in, 1 out]
        n334 = Array Subset(array=w922, index (row)=w916, length (row)=w915, index (col)=0 ("index"), length (col)=5 ("length")) -> (w926:string[][])
      }
    }
    "Diff list" <- w871
    n335 = local read "stop"() -> (w876:bool)
    "check loop" <- w875
  }
  n336 = Path To String(path=w13) -> (string=w1:string)
  n337 = property class="IWMPPlayer4"(reference="WindowsMediaPlayer", "enabled"=TRUE, "uiMode"="invisible") -> (reference out=w12:refnum<k7>, error out=w5:errorcluster, "settings"=w9:refnum<k7>, "controls"=w18:refnum<k7>)  [unwired: 1 in]
  n338 = property on="new picture" class="Pict"("Visible"=TRUE) -> ()  [unwired: 2 in, 2 out]
  n339 = property class="IWMPSettings"(reference=w9, error in=w5, "autoStart"=FALSE) -> (error out=w3:errorcluster, "volume"=w10:i32)  [unwired: 1 out]
  n340 = local write "Vol."(w10) -> ()
  n341 = property class="IWMPPlayer4"(reference=w12, error in=w3, "URL"=w1) -> (reference out=w17:refnum<k7>)  [unwired: 1 out]
  n342 = while {
    tunnel: w17 -> [w976]
    tunnel: w18 -> [w981]
    tunnel: w19 -> [w978]
    stop <- w974 stop-if-true
    n343 = flat-sequence {
      tunnel: w976 -> [w986]
      tunnel: [w986] -> w975
      frame #0 {
        n344 = Wait (ms)(milliseconds to wait=u32 300 ("millisecond multiple")) -> ()  [unwired: 1 out]
      }
    }
    n345 = property class="IWMPPlayer4"(reference=w975) -> (reference out=w979:refnum<k7>, error out=w977:errorcluster, "status"=w985:string)  [unwired: 1 in]
    "status" <- w985
    n346 = local read "Play Button"() -> (w982:bool)
    n347 = Equal?(x=w985, y="已停止") -> (x = y?=w983:bool)
    n348 = And(x=w983, y=w982) -> (x .and. y?=w980:bool)
    n349 = case shown="True" w980 {
      tunnel: w981 -> [_ w1003]
      tunnel: w979 -> [_ w992]
      tunnel: w978 -> [_ w991]
      tunnel: w977 -> [_ w988]
      frame False {
      }
      frame True {
        n350 = local read "index"() -> (w994:i32)
        n351 = List Folder(path=w991) -> (filenames=w995:string[])  [unwired: 3 in, 3 out]
        n352 = Increment(x=w994) -> (x+1=w993:i32)
        n353 = Array Size(array=w995) -> (size(s)=w1001:i32)
        n354 = Decrement(x=w1001) -> (x-1=w1002:i32)
        n355 = Greater?(x=w993, y=w1002) -> (0:w996:bool)
        n356 = Select(t=0, s=w996, f=w993) -> (s? t:f=w989:i32)
        n357 = Index Array(array=w995, index=w989) -> (element=w998:string)
        n358 = Build Path(base path=w991, name or relative path=w998) -> (appended path=w999:path)
        n359 = Path To String(path=w999) -> (string=w1000:string)
        n360 = property class="IWMPPlayer4"(reference=w992, error in=w988, "URL"=w1000) -> (error out=w990:errorcluster)  [unwired: 1 out]
        n361 = local write "index"(w989) -> ()
        n362 = invoke class="IWMPControls" method="play"(reference=w1003, error in=w990) -> ()  [unwired: 1 in, 3 out]
      }
    }
    n363 = local read "stop"() -> (w974:bool)
  }
  n364 = while {
    tunnel: w18 -> [w1011]
    tunnel: [w1010] -> w4
    tunnel: w9 -> [w1009]
    shift-right: [w1005] -> _
    shift-left: w16 -> [w1008]
    tunnel: w19 -> [w1007]
    tunnel: w17 -> [w1006]
    stop <- w1004 stop-if-true
    n365 = event shown="[1] \"Pause Button\": Value Change" {
      selector: _ -> [_ _ _ _ _]
      dyn-events: _ -> [_ _ _ _ _]
      timeout: _ -> [_ _ _ _ _]
      tunnel: w1011 -> [w1014 w1017 w1024 w1038 _]
      tunnel: [w1013 w1016 _ _ _] -> w1010
      tunnel: w1009 -> [_ _ _ _ w1054]
      tunnel: w1008 -> [w1012 w1015 w1036 w1051 w1053]
      tunnel: w1007 -> [_ _ w1030 w1044 _]
      tunnel: w1006 -> [_ _ w1037 w1052 _]
      tunnel: [w1012 w1015 w1031 w1046 w1053] -> w1005
      event "Play Button": Value Change {
        n366 = event-data() -> ()  [unwired: 1 in, 1 out]
        n367 = invoke class="IWMPControls" method="play"(reference=w1014) -> (error out=w1013:errorcluster)  [unwired: 2 in, 2 out]
      }
      event "Pause Button": Value Change {
        n368 = event-data() -> ("NewVal"=w1018:bool)  [unwired: 1 in]
        n369 = case shown="False" w1018 {
          tunnel: w1017 -> [w1019 w1022]
          tunnel: [w1020 w1021] -> w1016
          frame False {
            n370 = invoke class="IWMPControls" method="play"(reference=w1019) -> (error out=w1020:errorcluster)  [unwired: 2 in, 2 out]
          }
          frame True {
            n371 = invoke class="IWMPControls" method="pause"(reference=w1022) -> (error out=w1021:errorcluster)  [unwired: 2 in, 2 out]
          }
        }
      }
      event "Skip Forward Button": Value Change {
        n372 = event-data() -> ()  [unwired: 1 in, 1 out]
        n373 = List Folder(path=w1030) -> (filenames=w1035:string[])  [unwired: 3 in, 3 out]
        n374 = Increment(x=w1036) -> (x+1=w1033:i32)
        n375 = Array Size(array=w1035) -> (size(s)=w1026:i32)
        n376 = Decrement(x=w1026) -> (x-1=w1025:i32)
        n377 = Greater?(x=w1033, y=w1025) -> (0:w1034:bool)
        n378 = Select(t=0, s=w1034, f=w1033) -> (s? t:f=w1031:i32)
        n379 = Index Array(array=w1035, index=w1031) -> (element=w1029:string)
        n380 = Build Path(base path=w1030, name or relative path=w1029) -> (appended path=w1028:path)
        n381 = Path To String(path=w1028) -> (string=w1027:string)
        n382 = property class="IWMPPlayer4"(reference=w1037, "URL"=w1027) -> (error out=w1023:errorcluster)  [unwired: 1 in, 1 out]
        n383 = invoke class="IWMPControls" method="play"(reference=w1024, error in=w1023) -> ()  [unwired: 1 in, 3 out]
      }
      event "Skip Back Button": Value Change {
        n384 = event-data() -> ()  [unwired: 1 in, 1 out]
        n385 = List Folder(path=w1044) -> (filenames=w1050:string[])  [unwired: 3 in, 3 out]
        n386 = Decrement(x=w1051) -> (x-1=w1048:i32)
        n387 = Array Size(array=w1050) -> (size(s)=w1041:i32)
        n388 = Decrement(x=w1041) -> (x-1=w1040:i32)
        n389 = Less?(x=w1048, y=0) -> (x < y?=w1049:bool)
        n390 = Select(t=w1040, s=w1049, f=w1048) -> (s? t:f=w1046:i32)
        n391 = Index Array(array=w1050, index=w1046) -> (element=w1042:string)
        n392 = Build Path(base path=w1044, name or relative path=w1042) -> (appended path=w1045:path)
        n393 = Path To String(path=w1045) -> (string=w1043:string)
        n394 = property class="IWMPPlayer4"(reference=w1052, "URL"=w1043) -> (error out=w1039:errorcluster)  [unwired: 1 in, 1 out]
        n395 = invoke class="IWMPControls" method="play"(reference=w1038, error in=w1039) -> ()  [unwired: 1 in, 3 out]
      }
      event "Vol.": Value Change {
        n396 = event-data() -> ()  [unwired: 1 in, 1 out]
        n397 = property class="IWMPSettings"(reference=w1054, "volume"="Vol.") -> ()  [unwired: 1 in, 2 out]
      }
    }
    "index" <- w1005
    n398 = local read "stop"() -> (w1004:bool)
  }
  n399 = local write "stop"(FALSE ("stop")) -> ()
  n400 = invoke class="IWMPPlayer4" method="close"(reference=w17, error in=w4) -> ()  [unwired: 1 in, 3 out]
